vi "ADS1299EVM_Main.vi"() -> ()   [LabVIEW 2010]
doc: "ADS1292ECG-FE Software"
uses:
  Controls/Register/TYP_Reg_CHxSET.ctl
  Controls/Register/TYP_Reg_CONFIG1.ctl
  Controls/Register/TYP_Reg_CONFIG2.ctl
  Controls/Register/TYP_Reg_CONFIG3.ctl
  Controls/Register/TYP_Reg_LOFF.ctl
  Controls/Register/TYP_Reg_GPIO.ctl
  Controls/Register/TYP_Reg_MISC1.ctl
  Controls/Register/TYP_Reg_CONFIG4.ctl
  Controls/TYP_ACAnalysisParam.ctl
  lib_1299/Enqueue Classes/EVM Command class/EVMQueueCommand.lvclass
  lib_1299/Enqueue Classes/UserInput Command class/UserInput Command.lvclass
  lib_1299/Enqueue Classes/InternalState Command class/Internal State Command.lvclass
  Controls/Misc/TYP_DisableProp.ctl
  Modules/Estyx/TYP_ADS1299Estyx File Enum.ctl
  lib_1299/Enqueue Classes/UserDefined Command class/UserDefined Command class.lvclass
  Controls/Misc/TYP_PollingNotifierState.ctl
  Controls/Misc/TYP_PollingStatus.ctl
  Controls/Misc/TYP_SetTimeout.ctl
  Modules/Filter/TYP_FilterSettings.ctl
  <vilib>/event_ctls.llb/eventvkey.ctl
  lib_1299/Styx/lvstyx/Write/lvstyx_write_path_bool.vi
  <userlib>/Common/Queue with Cluster/Enqueue - Multiple Commands.vi
  lib_1299/Styx/lvstyx/Read/lvstyx_read_all_path_bool.vi
  lib_1299/Styx/lvstyx/Write/lvstyx_write_path_int.vi
  <vilib>/Utility/config.llb/Read Key (String).vi
  <vilib>/Utility/file.llb/Write To Spreadsheet File (string).vi
  <vilib>/Utility/file.llb/Write To Spreadsheet File (DBL).vi
  <vilib>/Utility/file.llb/Write To Spreadsheet File (I64).vi
  lib_1299/Styx/lvstyx/Read/lvstyx_read_all_path_hex.vi
  lib_1299/Styx/lvstyx/Read/lvstyx_read_all_path_int.vi
  lib_1299/lib1299.lvlib
  <vilib>/Analysis/NI_AALBase.lvlib
  <vilib>/Utility/config.llb/NI_LVConfig.lvlib
panel:
  in  "Normalize Data":bool=TRUE caption="Analysis Data is input referred"
  in  "Samples/CH":u32=1000
  in  "Show/Poll Lead Off Status":bool
  out "Status box":string="Connection Failure"
  in  "Acq - Single":bool
  out "Data Rate":dbl=500.0 format="%^#_6gSPS"
  in  "Acq - Continuous":bool
  out "Progress":u8(slide) caption="100%" scale=0.0..100.0
  out "ADC_ReadbackValue":u8 format="%.0x"
  in  "ADC_WriteValue":u8 format="%.0x"
  in  "ADC_Write2ADC":bool
  out "error out":errorcluster
  in  "error in (no error)":errorcluster
  in  "MainTab":T1(tab)
  out "About_FW_Ver":string caption="Firmware Version"
  out "About_DEV_ID":enum8{"ADS1299"}(ring) caption="Device ID"
  out "About_REV_ID":u8 caption="Rev"
  in  "Reset Mode":enum32{"Reset2Device", "Reset2Programmed"}(radio)=enum."Reset2Programmed"
  in  "RESET":bool caption="Reset"
  in  "STANDBY":bool caption="Standby"
  in  "Registers Tab":T2(tab)
  in  "CH8SET":T3={"PD#"=enum."Normal Operation", "GAIN#"=enum."24", "SRB2"=enum."Open (Off)", "MUX#"=enum."Normal Electrode"} caption="Channel 8 Control Register (CH8SET)"
  in  "CH7SET":T3={"PD#"=enum."Normal Operation", "GAIN#"=enum."24", "SRB2"=enum."Open (Off)", "MUX#"=enum."Normal Electrode"} caption="Channel 7 Control Register (CH7SET)"
  in  "CH6SET":T3={"PD#"=enum."Normal Operation", "GAIN#"=enum."24", "SRB2"=enum."Open (Off)", "MUX#"=enum."Normal Electrode"} caption="Channel 6 Control Register (CH6SET)"
  in  "CH5SET":T3={"PD#"=enum."Normal Operation", "GAIN#"=enum."24", "SRB2"=enum."Open (Off)", "MUX#"=enum."Normal Electrode"} caption="Channel 5 Control Register (CH5SET)"
  in  "CH4SET":T3={"PD#"=enum."Normal Operation", "GAIN#"=enum."24", "SRB2"=enum."Open (Off)", "MUX#"=enum."Normal Electrode"} caption="Channel 4 Control Register (CH4SET)"
  in  "CH3SET":T3={"PD#"=enum."Normal Operation", "GAIN#"=enum."24", "SRB2"=enum."Open (Off)", "MUX#"=enum."Normal Electrode"} caption="Channel 3 Control Register (CH3SET)"
  in  "CH2SET":T3={"PD#"=enum."Normal Operation", "GAIN#"=enum."24", "SRB2"=enum."Open (Off)", "MUX#"=enum."Normal Electrode"} caption="Channel 2 Control Register (CH2SET)"
  in  "CH1SET":T3={"PD#"=enum."Normal Operation", "GAIN#"=enum."24", "SRB2"=enum."Open (Off)", "MUX#"=enum."Normal Electrode"} caption="Channel 1 Control Register (CH1SET)"
  in  "Globally Set Channels":T3={"PD#"=enum."Normal Operation", "GAIN#"=enum."24", "SRB2"=enum."Open (Off)", "MUX#"=enum."Normal Electrode"}
  in  "CONFIG3":T4={"PD_REFBUF"=enum."Enabled", "BIAS_MEAS"=enum."Open", "BIASREF_INT"=enum."BIASREF fed externally", "PD_BIAS"=enum."Disabled"} caption="Configuration Register 3 (CONFIG3)"
  in  "CONFIG2":T5 caption="Configuration Register 2 (CONFIG2)"
  in  "CONFIG1":T6 caption="Configuration Register 1 (CONFIG1)"
  in  "LOFF":T7 caption="Lead-Off Control Register (LOFF)"
  in  "LOFF_FLIP_All":bool caption="Set All LOFF FLIP Bits"
  in  "LOFFN_All":bool caption="Set All LOFFN Bits"
  in  "LOFFP_All":bool caption="Set All LOFFP Bits"
  in  "LOFF_SENSP":bool[](array[boolean])=[FALSE, FALSE, FALSE, FALSE, FALSE, FALSE, FALSE, FALSE] caption="Lead Off Sense Positive Electrode"
  in  "LOFF_SENSN":bool[](array[boolean])=[FALSE, FALSE, FALSE, FALSE, FALSE, FALSE, FALSE, FALSE] caption="Lead Off Sense Negative Electrode"
  in  "LOFF_FLIP":bool[](array[boolean])=[FALSE, FALSE, FALSE, FALSE, FALSE, FALSE, FALSE, FALSE] caption="Lead Off Current Direction"
  in  "BIASSENSN":bool[](array[boolean])=[FALSE, FALSE, FALSE, FALSE, FALSE, FALSE, FALSE, FALSE] caption="Bias Sense Negative Electrode"
  in  "BIASSENSP":bool[](array[boolean])=[FALSE, FALSE, FALSE, FALSE, FALSE, FALSE, FALSE, FALSE] caption="Bias Sense Positive Electrode"
  in  "BIASSENSP_All":bool caption="Set All BIASSENSP Bits"
  in  "BIASSENSN_All":bool caption="Set All BIASSENSN Bits"
  in  "GPIO":T8={"GPIOC1"=TRUE, "GPIOC2"=TRUE, "GPIOC3"=TRUE, "GPIOC4"=TRUE, "GPIOD1"=FALSE, "GPIOD2"=FALSE, "GPIOD3"=FALSE, "GPIOD4"=FALSE} caption="General-Purpose I/O Register (GPIO)"
  in  "MISC1":T9
  in  "CONFIG4":T10 caption="Configuration Register 4 (CONFIG4)"
  in  "Refresh_ShadowReg":bool
  out "ShadowRegister":string[][](table) caption="Device Registers"
  in  "Analysis Control":enum32{"Scope", "Histogram", "FFT"}(tab)
  in  "Notch Freq":u16(ring)=60 items=["50Hz"=50, "60Hz"=60]
  in  "LPF Cutoff":dbl=0.1 caption="Cutoff Freq" format="%0.4fHz"
  in  "LPF Order":i32=3 caption="Filter Order"
  in  "LPF Enable":bool
  in  "Notch Order":i32=2 caption="Filter Order"
  in  "Notch Enable":bool
  in  "HPF Cutoff":dbl=0.1 caption="Cutoff Freq" format="%0.4fHz"
  in  "HPF Order":i32=3 caption="Filter Order"
  in  "HPF Enable":bool
  in  "Table_Scope":bool
  out "Graph - Scope":dbl[][](graph) caption="Scope Channels"
  in  "Plot Selector - Scope":u16(ring) caption="Plot" items=["All Channels", "Channel 1", "Channel 2", "Channel 3", "Channel 4", "Channel 5", "Channel 6", "Channel 7", "Channel 8"]
  in  "Histogram Bins":i32=10
  out "Graph - Histogram":T11(graph)
  in  "Plot Selector - Histogram":u16(ring) caption="Plot" items=["All Channels", "Channel 1", "Channel 2", "Channel 3", "Channel 4", "Channel 5", "Channel 6", "Channel 7", "Channel 8"]
  in  "Table_Histogram":bool
  in  "High Frequency":dbl=100.0 format="%.03pHz"
  out "Analysis - Dynamic Range":string[][](table) caption="Dynamic Range"
  in  "AC Analysis Parameters":T12={"DC Leakage"=5, "Number of Harmonics"=6, "HarmLeakage"=3, "FundLeakage"=15, "LoFreq (Hz)"=50.0, "HiFreq (Hz)"=100.0, "Window"=enum."None ", "Reference"=TRUE} {"HiFreq (Hz)" format="%.03pHz"; "LoFreq (Hz)" format="%.03pHz"; "FundLeakage" min=1 step=2; "HarmLeakage" min=1 step=2; "DC Leakage" min=1 step=1}
  in  "AinFreq_Desired":dbl=60.0 caption="Desired Ain Frequency" format="%0.3pHz"
  out "AinFreq_Ideal":dbl=60.1 caption="Ideal Ain Frequency" format="%.06pHz"
  in  "Input Amplitude(Vpp)":dbl=0.5 format="%.3g"
  out "Graph - FFT":cluster{i32, dbl, dbl[]}[](graph) caption="FFT Magnitude Plot (dB)"
  in  "Plot Selector - FFT":u16(ring) caption="Plot" items=["All Channels", "Channel 1", "Channel 2", "Channel 3", "Channel 4", "Channel 5", "Channel 6", "Channel 7", "Channel 8"]
  in  "Table_FFT":bool
  in  "Low Frequency":dbl=50.0 format="%.03pHz"
  in  "Save Data:Volts":bool caption="Data - Volts"
  in  "Save Analysis:FFT":bool caption="FFT Analysis"
  in  "Save_CH8":bool=TRUE caption="CH 8"
  in  "Save_CH7":bool=TRUE caption="CH 7"
  in  "Save_CH6":bool=TRUE caption="CH 6"
  in  "Save_CH5":bool=TRUE caption="CH 5"
  in  "Save_CH4":bool=TRUE caption="CH 4"
  in  "Save_CH3":bool=TRUE caption="CH 3"
  in  "Save_CH2":bool=TRUE caption="CH 2"
  in  "Save_CH1":bool=TRUE caption="CH 1"
  in  "Save Data:Histogram":bool caption="Histogram Data"
  in  "Save Data:FFT":bool caption="FFT Data"
  in  "Save Analysis:Scope":bool caption="Scope Analysis"
  in  "Save Analysis:Histogram":bool caption="Histogram Analysis"
  in  "Save Analysis:ShadowRegister":bool caption="Register Settings"
  in  "User Comments":string
  in  "Save Data:Codes":bool caption="Data - Codes"
  in  "Directory to Save Files":path=path "C:/Program Files/ADS1299ECG-FE/saved"
  in  "Record ID":i32 caption="Record Number"
  in  "Save to File":bool
  # "ADS1299EEG-FE"
  # "Debug - Manual Register Write"
  # "Product Safety Warnings, Restrictions and Disclaimers\n\nThe following Evaluation Board ADS1299ECG-FE set-up, use and application requirements must be followed:\n\n1.  NOT for diagnostic use.\n2.  NOT for for direct use with, or use in proximity of, an energized Defibrillator.\n3.  ONLY for Feasibility Evaluation in Laboratory/Development Environments.\n4.  The ADS1299ECG-FE intended application is solely for use in a laboratory/development environment, restricted to feasibility evaluation and development purposes, and not for\n     diagnostic purposes and/or interface with human beings and/or animals.\n5.  ONLY for use by qualified engineers and technicians familiar with the potential electrical shock, fire and personal injury risks associated in handling subassembly electrical and\n     mechanical components.\n6.  Use in conjunction with and/or adjacent to a defibrillator is strictly prohibited; application interface electronics shall not exceed their intended ratings. Refer to user instructions\n     and the ADS1299ECG-FE for further interface details.\n\n\nFor further information on application safety, refer to the standard TI terms and conditions documentation XXXXXXXXX"
  # "Motherboard:  MMB0\nTexas Instruments Inc (c) 2010"
  # "Reset Options"
  # "Global Channel Registers"
  # "Channel Control Registers"
  # "Lead-Off Detection and Current Direction Control Registers"
  # "LOFFP8             LOFFP7            LOFFP6             LOFFP5             LOFFP4             LOFFP3            LOFFP2             LOFFP1"
  # "LOFFN8             LOFFN7            LOFFN6             LOFFN5             LOFFN4            LOFFN3            LOFFN2             LOFFN1"
  # "LOFF_FLIP8      LOFF_FLIP7      LOFF_FLIP6      LOFF_FLIP5     LOFF_FLIP4      LOFF_FLIP3      LOFF_FLIP2     LOFF_FLIP1"
  # "BIAS Control Registers"
  # "BIASP8              BIASP7            BIASP6              BIASP5             BIASP4              BIASP3             BIASP2              BIASP1"
  # "BIASN8              BIASN7             BIASN6             BIASN5             BIASN4             BIASN3             BIASN2            BIASN1"
  # "Input"
  # "GPIOCx"
  # "Output"
  # "GPIODx"
  # "GPIO1                  GPIO2                 GPIO3                  GPIO4"
  # "(automatically updates if coming from another page)"
  # "Post Processing Filters"
  # "User Defined Dynamic Range"
  # "Coherent Frequency Calculator"
  # "User Comments/Notes"
  # "Analysis to Save:"
  # "Data to Save:"
  # "Channels to Save"
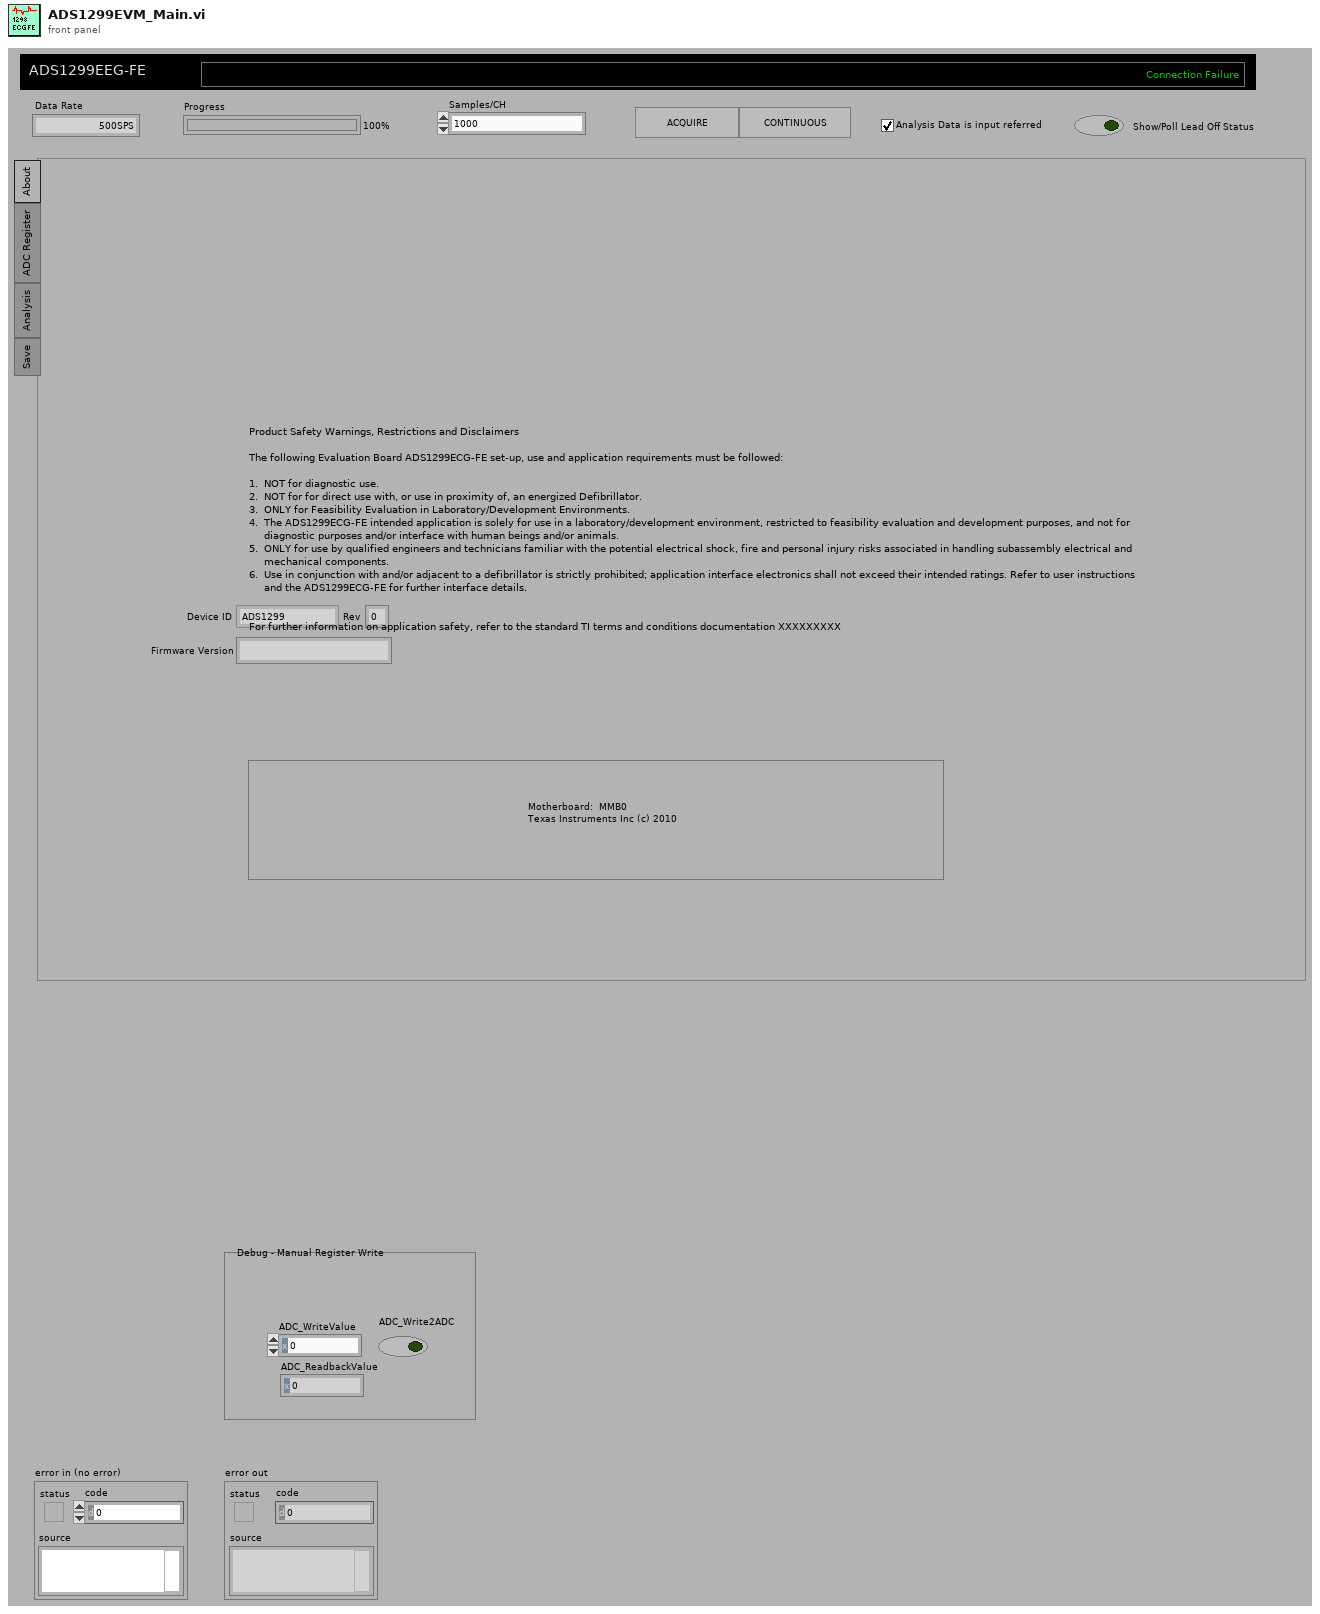
[diagram p1: front panel]
types:
  T1 = enum32{"About", "ADC Register", "Analysis", "Save"}
  T2 = enum32{"Channel Registers", "LOFF and BIAS", "GPIO and OTHER Registers", "Register Map"}
  T3 = typedef "TYP_Reg_CHxSET.ctl" = cluster{"PD#":enum16{"Normal Operation", "Power-down"}, "GAIN#":enum16{"1", "2", "4", "6", "8", "12", "24"}, "SRB2":enum16{"Open (Off)", "Closed (On)"}, "MUX#":enum16{"Normal Electrode", "Input Short", "BIAS Measurement", "MVDD", "Temperature Sensor", "Test Signal", "BIAS Positive Electrode Driver", "BIAS Negative Electrode Driver"}}
  T4 = typedef "TYP_Reg_CONFIG3.ctl" = cluster{"PD_REFBUF":enum16{"Disabled", "Enabled"}, "BIAS_MEAS":enum16{"Open", "BIASIN Routed"}, "BIASREF_INT":enum16{"BIASREF fed externally", "BIASREF = (AVDD-AVSS)/2"}, "PD_BIAS":enum16{"Disabled", "Enabled"}}
  T5 = typedef "TYP_Reg_CONFIG2.ctl" = cluster{"INT_CAL":enum16{"Driven Externally", "Generated Internally"}, "CAL_AMP":enum16{"(VREFP-VREFN)/2.4", "2x(VREFP-VREFN)/2.4"}, "CAL_FREQ":enum16{"f(CLK)/2^21", "f(CLK)/2^20", "N/A", "DC"}}
  T6 = typedef "TYP_Reg_CONFIG1.ctl" = cluster{"DAISY_EN":enum16{"Daisy Chain Mode", "Multiple Readback Mode"}, "CLK_EN":enum16{"Output Disabled", "Output Enabled"}, "DR":enum16{"f(MOD) /64", "f(MOD) /128", "f(MOD) /256", "f(MOD) /512", "f(MOD) /1024", "f(MOD) /2048", "f(MOD) /4096"}}
  T7 = typedef "TYP_Reg_LOFF.ctl" = cluster{"COMP_TH":enum16{"Positive - 95% : Negative - 5%", "Positive - 92.5% : Negative - 7.5%", "Positive - 90% : Negative - 10%", "Positive - 87.5% : Negative - 12.5%", "Positive - 85% : Negative - 15%", "Positive - 80% : Negative - 20%", "Positive - 75% : Negative - 25%", "Positive - 70% : Negative - 30%"}, "ILEAD_OFF":enum16{"6nA", "24nA", "6uA", "24uA"}, "FLEAD_OFF":enum16{"DC lead-off detection", "AC lead-off detection at SYS_CLK/(2^18)", "AC lead-off detection at SYS_CLK/(2^16)", "AC lead-off detection at fdr/4"}}
  T8 = typedef "TYP_Reg_GPIO.ctl" = cluster{"GPIOC1":bool, "GPIOC2":bool, "GPIOC3":bool, "GPIOC4":bool, "GPIOD1":bool, "GPIOD2":bool, "GPIOD3":bool, "GPIOD4":bool}
  T9 = typedef "TYP_Reg_MISC1.ctl" = cluster{"SRB1":enum16{"Open (Off)", "Closed (On)"}}
  T10 = typedef "TYP_Reg_CONFIG4.ctl" = cluster{"PD_LOFF_COMP":enum16{"Comparator Disabled", "Comparator Enabled"}}
  T11 = cluster{"X Values":dbl[], "Histogram: h(x)":i32[]}[]
  T12 = typedef "TYP_ACAnalysisParam.ctl" = cluster{"DC Leakage":i8, "Number of Harmonics":i8, "HarmLeakage":i8, "FundLeakage":i32, "LoFreq (Hz)":ext, "HiFreq (Hz)":ext, "Window":enum16{"None ", "Hanning", "Hamming", "Blackman-Harris", "Exact Blackman", "Blackman", "Flat Top", "4 Term B-Harris ", "7 Term B-Harris", "Low Sidelobe"}, "Reference":bool}
  T13 = typedef "TYP_ADS1299Estyx File Enum.ctl" = enum16{"|version", "|id", "ads1299evm|blocksize_samples", "ads1299evm|acquire", "ads1299evm|data", "conf|ch1set", "conf|ch2set", "conf|ch3set", "conf|ch4set", "conf|ch5set", "conf|ch6set", "conf|ch7set", "conf|ch8set", "conf|config1", "conf|config2", "conf|config3", "conf|devid", "conf|gpio", "conf|loff", "conf|loffflip", "conf|loffsensn", "conf|loffsensp", "conf|loffstatn", "conf|loffstatp", "conf|misc2", "conf|misc1", "conf|biassensn", "conf|biassensp", "conf|reset", "conf|sleep", "conf|config4", "led|dp", "led|seg", "led|ch", "mmb0|pll", "mmb0|clkout", "mmb0|clkfreq"}
  T14 = typedef "TYP_DisableProp.ctl" = u8
  T15 = typedef "TYP_PollingNotifierState.ctl" = cluster{"State":T16, "Data":i32}
  T16 = typedef "TYP_PollingStatus.ctl" = enum16{"Init", "Start", "Stop", "Pause", "Resume"}
  T17 = typedef "TYP_SetTimeout.ctl" = cluster{"Timeout (ms)":i16, "Timeout Enable?":bool}
  T18 = enum32{"invalid app kind", "Development System", "Run Time System", "Student Edition", "Embedded LabVIEW", "Evaluation", "Custom"}
  T19 = typedef "Rendezvous RefNum" = refnum<k1>
  T20 = typedef "TYP_AnalysisData.ctl" = cluster{"Status (Codes)":i32[], "Data (Codes)":i32[][], "Temp - Data (Volts)":dbl[][], "FFT":cluster{"FFT Data":cluster{i32, dbl, dbl[]}[], "Table Col Hdrs":string[], "Table Row Hdrs":string[], "Analysis Data":string[][], "CMRR/BW Table":string[][][]}, "Histogram":cluster{"Histogram Data":cluster{"X Values":dbl[], "Histogram: h(x)":i32[]}[], "Table Col Hdrs":string[], "Table Row Hdrs":string[], "Analysis Data":string[][]}, "Scope":cluster{"Table Col Hdrs":string[], "Table Row Hdrs":string[], "Analysis Data":string[][]}, "ECG":cluster{"AUX/LEAD":dbl[][], "Chest Leads":dbl[][], "Graph Labels (current)":string[]}, "Respiration":dbl[]}
  T21 = typedef "TYP_1299MainShifter.ctl" = cluster{"RegMap Data":T22[], "Register Names":string[], "ECG Zoom Limits":cluster{"Top":i32[], "Bottom":i32[]}, "Acq Timeout":u16, "f(CLK)":dbl, "Vref":dbl, "Word Bits":i32, "INI Info":cluster{"Data Dir":path, "Startup Dir":path, "Version":string, "Build":i16}, "Styx Enum Strings":string[]}
  T22 = typedef "TYP_ADSxxxx Register.ctl" = cluster{"Name":string, "Description":string, "Register":u16, "Default":u16, "Value":u16, "Base":u16, "RegMap Names":string[], "RegMap":T23[], "Item Count":u8}
  T23 = typedef "TYP_RegMap Item.ctl" = cluster{"Name":string, "MSB":u16, "LSB":u16, "Value":u16, "Mask":u16}
  T24 = typedef "eventvkey.ctl" = enum16{"ASCII", "Enter", "Return", "Shift", "Ctrl", "Alt", "Cmd", "Opt", "Caps", "NumLock", "Clear", "Break", "Up", "Down", "Left", "Right", "Insert", "Delete", "Home", "End", "PageUp", "PageDown", "Escape", "Help", "Pause", "ScrollLock", "F1", "F2", "F3", "F4", "F5", "F6", "F7", "F8", "F9", "F10", "F11", "F12", "F13", "F14", "F15", "F16", "F17", "F18", "F19", "F20", "F21", "F22", "F23", "F24", "Play", "VolumeUp", "VolumeDown", "Mute", "Two Byte Char"}
  T25 = enum32{"Channel Registers", "LOFF and RLD", "GPIO and OTHER Registers", "Register Map"}
  T26 = enum16{"DC lead-off detection", "AC lead-off detection at SYS_CLK/(2^18)", "AC lead-off detection at SYS_CLK/(2^16)", "AC lead-off detection at fdr/4"}
  T27 = enum16{"open", "replace", "create", "open or create", "replace or create", "replace or create with confirmation"}
  T28 = cluster{"LOFF_STATP":bool[], "LOFF_STATN":bool[]}
  T29 = enum16{"BIASREF fed externally", "BIASREF = (AVDD-AVSS)/2"}
  T30 = enum16{"Comparator Disabled", "Comparator Enabled"}
  T31 = typedef "TYP_Queue with Cluster Reference.ctl" = refnum<queue>
  T32 = typedef "lib1299.lvlib/TYP_EVM Plugin Pointers.ctl" = cluster{"Connection ptr":u32, "Client ptr":u32, "Data File ptr":u32}
  T33 = typedef "TYP_CtrlNameArray.ctl" = cluster{"References":refnum<vi>[], "Names/Labels":string[]}
  T34 = typedef "TYP_1299ShadowRegister.ctl" = cluster{"ID":T35, "Config1 ":T6, "Config2 ":T5, "Config3 ":T4, "Config4":T10, "CH1SET":T3, "CH2SET":T3, "CH3SET":T3, "CH4SET":T3, "CH5SET":T3, "CH6SET":T3, "CH7SET":T3, "CH8SET":T3, "MISC2":T36, "MISC1":T9, "LOFF ":T7, "BIASSENSP":bool[], "BIASSENSN":bool[], "LOFF_STATP":bool[], "LOFF_STATN":bool[], "LOFF_SENSP":bool[], "LOFF_SENSN":bool[], "LOFF_FLIP":bool[], "GPIO":cluster{"Data":bool[], "Direction":bool[]}}
  T35 = typedef "TYP_Reg_ID.ctl" = cluster{"REV_ID":u8, "DEV_ID":u16}
  T36 = typedef "TYP_Reg_MISC2.ctl" = cluster{"RegValue":dbl}
  T37 = typedef "TYP_CtrlRefShifter.ctl" = cluster{"Shadow Regs":cluster{"References":refnum<vi>[], "Names/Labels":string[]}, "Reg - PageCtrls":cluster{"References":refnum<vi>[], "Names/Labels":string[]}, "Reg - AllCtrls":cluster{"References":refnum<vi>[], "Names/Labels":string[]}, "Anlyz - PageCtrls":cluster{"References":refnum<vi>[], "Names/Labels":string[]}, "Anlyz - AllCtrls":cluster{"References":refnum<vi>[], "Names/Labels":string[]}}
  T38 = typedef "imagedata.ctl" = cluster{"image type":i32, "image depth":i32, "image":u8[], "mask":u8[], "colors":u32[], "Rectangle":cluster{"left":i16, "top":i16, "right":i16, "bottom":i16}}
  T39 = typedef "NI_LVConfig.lvlib/Config Data RefNum.ctl" = refnum<k1>
  T40 = typedef "TYP_Queue Cluster Element.ctl" = cluster{"Command":string, "Data":variant}
  T41 = typedef "TYP_FilterSettings.ctl" = cluster{"Cutoff":dbl, "Order":i32}
  T42 = cluster{"Freq (Hz)":dbl[][], "SNR (dBFS)":dbl[], "Fund(dB)":dbl}
  T43 = cluster{"SNR(dBFS)":dbl, "SNRD(dB)":dbl, "THD (dBc)":dbl, "SFDR(dBc)":dbl, "ENOB":dbl, "enob":dbl, "#ofHarm(SNR)":dbl, "WoSpur(dbFS)":dbl, "2nd HD (dBc)":dbl, "3rd HD (dBc)":dbl, "4th HD (dBc)":dbl, "5th HD (dBc)":dbl, "Ampl.":dbl}
  T44 = cluster{"X Values":dbl[], "Histogram: h(x)":i32[]}
  T45 = cluster{"DAISY_EN":enum16{"Daisy Chain Mode", "Multiple Readback Mode"}, "CLK_EN":enum16{"Output Disabled", "Output Enabled"}, "DR":enum16{"f(MOD) /64", "f(MOD) /128", "f(MOD) /256", "f(MOD) /512", "f(MOD) /1024", "f(MOD) /2048", "f(MOD) /4096"}}
  T46 = cluster{"INT_CAL":enum16{"Driven Externally", "Generated Internally"}, "CAL_AMP":enum16{"(VREFP-VREFN)/2.4", "2x(VREFP-VREFN)/2.4"}, "CAL_FREQ":enum16{"f(CLK)/2^21", "f(CLK)/2^20", "N/A", "DC"}}
  T47 = cluster{"PD_REFBUF":enum16{"Disabled", "Enabled"}, "BIAS_MEAS":enum16{"Open", "BIASIN Routed"}, "BIASREF_INT":enum16{"BIASREF fed externally", "BIASREF = (AVDD-AVSS)/2"}, "PD_BIAS":enum16{"Disabled", "Enabled"}}
  T48 = cluster{"PD_LOFF_COMP":enum16{"Comparator Disabled", "Comparator Enabled"}}
  T49 = enum16{"f(MOD) /64", "f(MOD) /128", "f(MOD) /256", "f(MOD) /512", "f(MOD) /1024", "f(MOD) /2048", "f(MOD) /4096"}
  T50 = cluster{"COMP_TH":enum16{"Positive - 95% : Negative - 5%", "Positive - 92.5% : Negative - 7.5%", "Positive - 90% : Negative - 10%", "Positive - 87.5% : Negative - 12.5%", "Positive - 85% : Negative - 15%", "Positive - 80% : Negative - 20%", "Positive - 75% : Negative - 25%", "Positive - 70% : Negative - 30%"}, "ILEAD_OFF":enum16{"6nA", "24nA", "6uA", "24uA"}, "FLEAD_OFF":enum16{"DC lead-off detection", "AC lead-off detection at SYS_CLK/(2^18)", "AC lead-off detection at SYS_CLK/(2^16)", "AC lead-off detection at fdr/4"}}
  T51 = cluster{"SRB1":enum16{"Open (Off)", "Closed (On)"}}
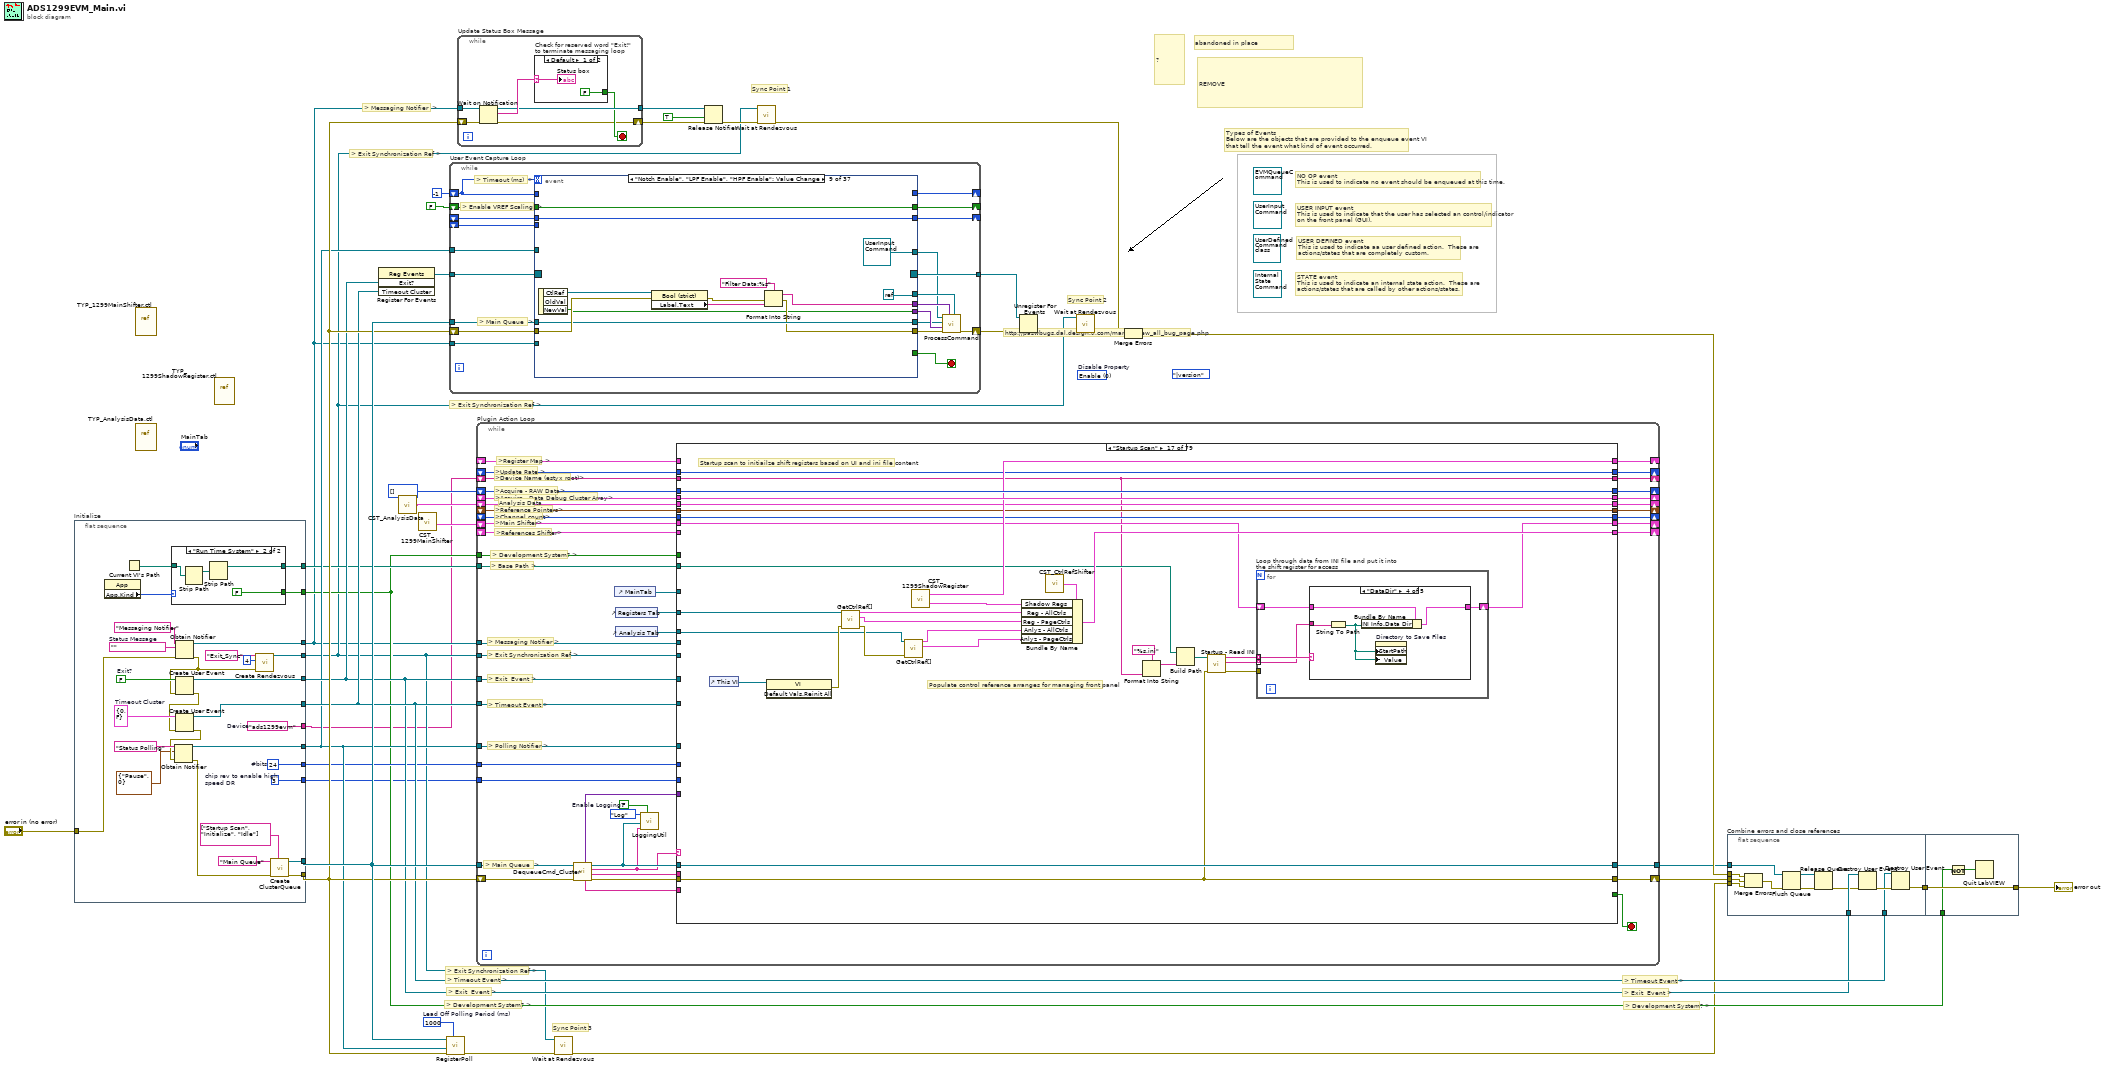
[diagram p0: block diagram]
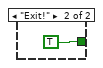
[diagram p2: hidden frame]
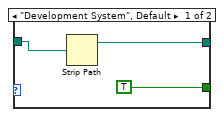
[diagram p3: hidden frame]
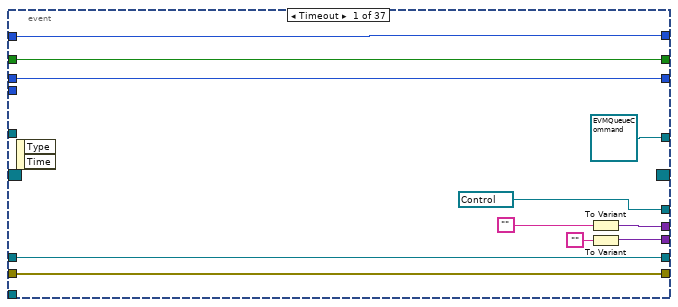
[diagram p4: hidden frame]
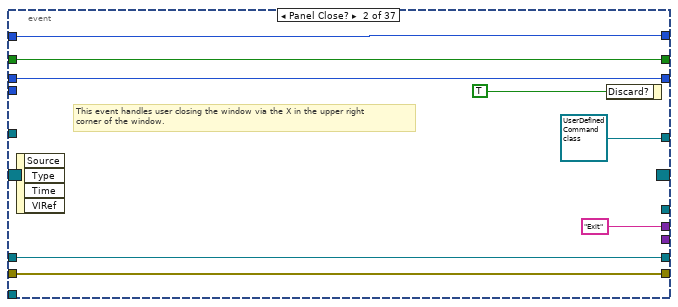
[diagram p5: hidden frame]
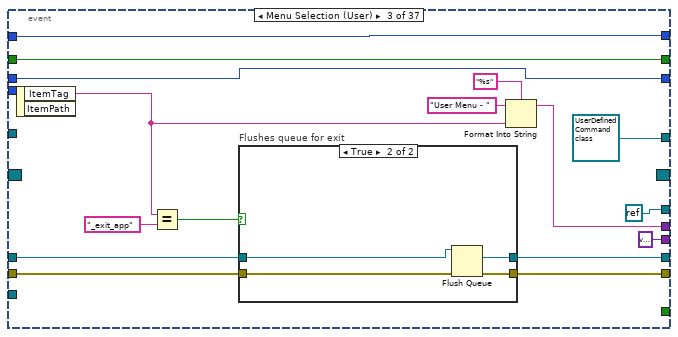
[diagram p6: hidden frame]
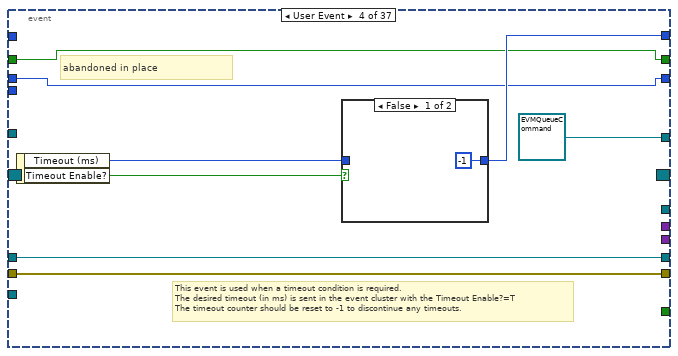
[diagram p8: hidden frame]
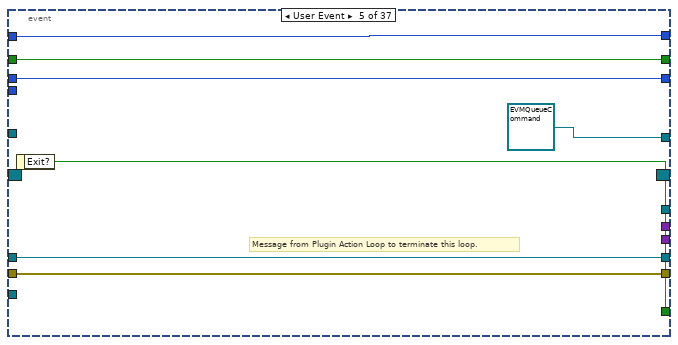
[diagram p10: hidden frame]
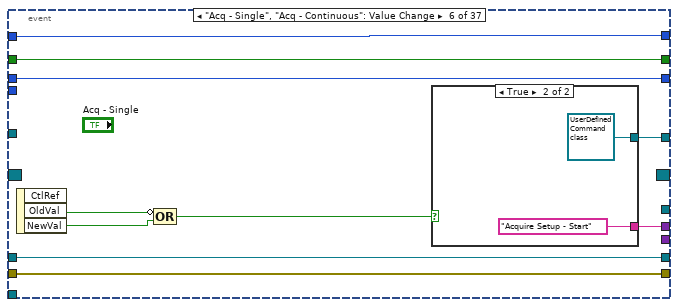
[diagram p11: hidden frame]
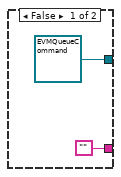
[diagram p12: hidden frame]
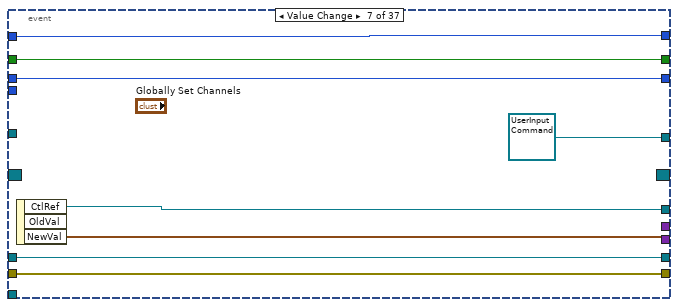
[diagram p13: hidden frame]
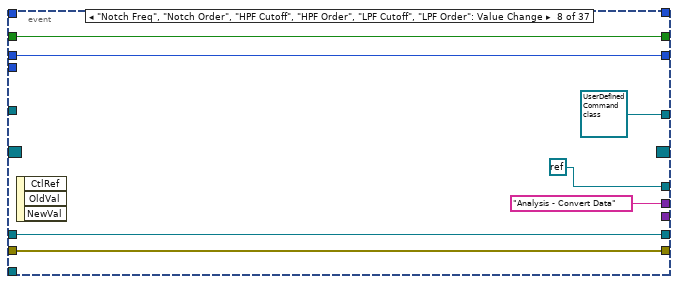
[diagram p14: hidden frame]
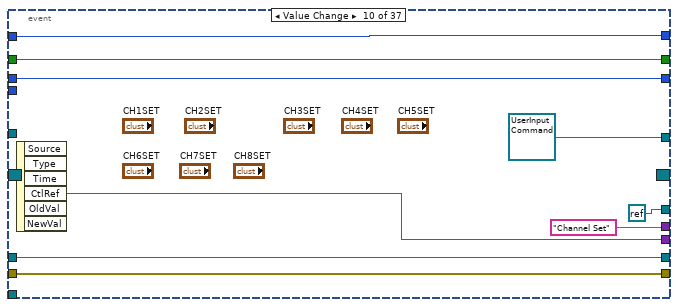
[diagram p15: hidden frame]
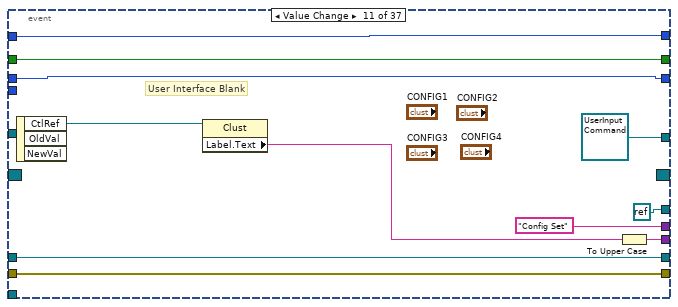
[diagram p16: hidden frame]
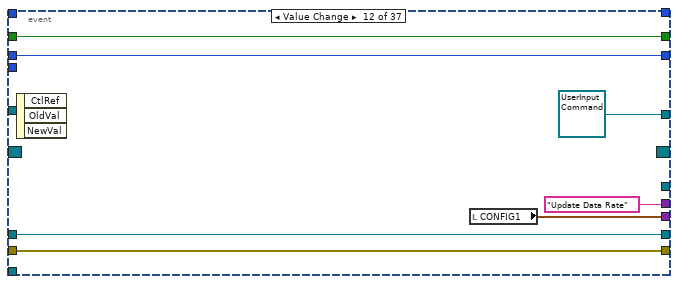
[diagram p17: hidden frame]
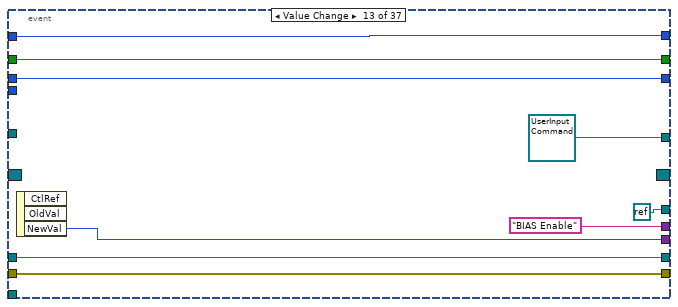
[diagram p18: hidden frame]
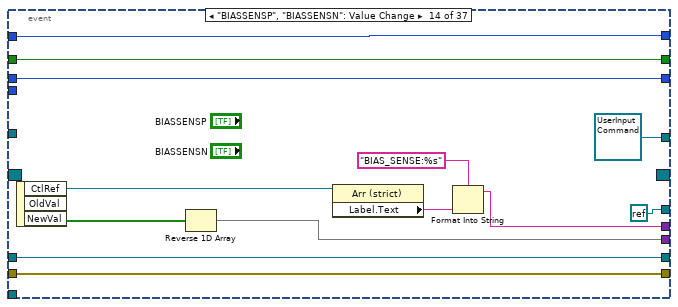
[diagram p19: hidden frame]
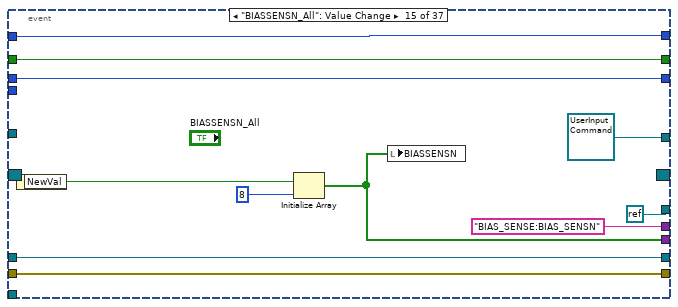
[diagram p20: hidden frame]
diagram:
  (unwired) refnum<class "UserDefined Command class.lvclass"> refnum ("UserDefined Command class.lvclass")
  (unwired) TYP_ADS1299Estyx_File_Enum."|version" ("Styx File Tags - Enum")
  w25 = 1000  # Lead Off Polling Period (ms)
  (unwired) T14 0 items=["Enable", "Disable", "Disable/Gray"]  # Disable Property
  (unwired) refnum<class "Internal State Command.lvclass"> refnum ("Internal State Command.lvclass")
  (unwired) refnum<class "UserInput Command.lvclass"> refnum ("UserInput Command.lvclass")
  (unwired) refnum<class "EVMQueueCommand.lvclass"> refnum ("EVMQueueCommand.lvclass")
  # "http://paswbugs.dal.design.ti.com/mantis/view_all_bug_page.php"
  # "Sync Point 3"
  # "Sync Point 2"
  # "Sync Point 1"
  # "> Exit Synchronization Ref >"
  # "> Exit Synchronization Ref >"
  # "> Exit Synchronization Ref >"
  # "> Development System? >"
  # "> Development System? >"
  # "abandoned in place"
  # "USER DEFINED event\nThis is used to indicate aa user defined action.  These are \nactions/states that are completely custom."
  # "REMOVE"
  # "?"
  # "STATE event\nThis is used to indicate an internal state action.  These are \nactions/states that are called by other actions/states."
  # "USER INPUT event\nThis is used to indicate that the user has selected an control/indicator\non the front panel (GUI)."
  # "NO OP event\nThis is used to indicate no event should be enqueued at this time."
  # "Types of Events\nBelow are the objects that are provided to the enqueue event VI\nthat tell the event what kind of event occurred."
  # "> Messaging Notifier  >"
  # "> Timeout Event >"
  # "> Exit  Event >"
  # "> Timeout Event >"
  # "> Exit  Event >"
  n1 = flat-sequence "Initialize" {
    tunnel: [w54] -> w24
    tunnel: [w55] -> w26
    tunnel: [w65] -> w21
    tunnel: [w62] -> w22
    tunnel: "error in (no error)" -> [w60]
    tunnel: [w58] -> w2
    tunnel: [w49] -> w20
    tunnel: [w47] -> w16
    tunnel: [w44] -> w15
    tunnel: [w43] -> w12
    tunnel: [w39] -> w5
    tunnel: [w38] -> w4
    tunnel: [w37] -> w1
    frame #0 {
      w37 = "ads1299evm"  # Device
      w38 = 3  # chip rev to enable high speed DR
      w47 = 24  # #bits
      w57 = ""  # Status Message
      w63 = T17 {"Timeout (ms)"=0, "Timeout Enable?"=FALSE}  # Timeout Cluster
      w64 = FALSE  # Exit?
      n2 = property class="App"() -> ("App.Kind"=w46:T18)  [unwired: 2 in, 2 out]
      n3 = Current VI's Path() -> (path=w45:path)
      n4 = case shown="\"Run Time System\"" w46 {
        tunnel: w45 -> [w68 w72]
        tunnel: [w67 w70] -> w44
        tunnel: [TRUE FALSE] -> w43
        frame "Development System", Default {
          n5 = Strip Path(path=w68) -> (stripped path=w67:path)  [unwired: 1 out]
        }
        frame "Run Time System" {
          n6 = Strip Path(path=w72) -> (stripped path=w71:path)  [unwired: 1 out]
          n7 = Strip Path(path=w71) -> (stripped path=w70:path)  [unwired: 1 out]
        }
      }
      n8 = Obtain Notifier(name (unnamed)="Messaging Notifier", notification data type=w57, error in (no error)=w60) -> (notifier out=w58:refnum<notifier>, error out=w42:errorcluster)  [unwired: 1 in, 1 out]
      n9 = Create User Event(user event datatype=w64, error in=w42) -> (user event=w65:refnum<user-event>, error out=w61:errorcluster)
      n10 = Create User Event(user event datatype=w63, error in=w61) -> (user event=w62:refnum<user-event>, error out=w51:errorcluster)
      n11 = Obtain Notifier(name (unnamed)="Status Polling", notification data type=T15 {"State"=enum."Pause", "Data"=0} ("PollingNotifier"), error in (no error)=w51) -> (notifier out=w49:refnum<notifier>, error out=w50:errorcluster)  [unwired: 1 in, 1 out]
      n12 = call <vilib>:"Create Rendezvous.vi"("error in (no error)"=w42, "size (2)"=4, "name (unnamed)"="Exit_Sync") -> ("rendezvous"=w39:T19)  [unwired: 4 out]
      n13 = call <userlib>:"Create ClusterQueue.vi"("Initial Commands"=string[] ["Startup Scan", "Initialize", "Idle"], "error in"=w50, "Queue Name"="Main Queue" ("name (unnamed)")) -> ("error out"=w54:errorcluster, "Queue Out"=w55:refnum<queue>)  [unwired: 7 out]
    }
  }
  n14 = vi-ref "TYP_1299MainShifter.ctl"() -> ()  [unwired: 1 out]
  n15 = vi-ref "TYP_AnalysisData.ctl"() -> ()  [unwired: 1 out]
  n16 = vi-ref "TYP_1299ShadowRegister.ctl"() -> ()  [unwired: 1 out]
  n17 = register-events(w21, w22) -> (reference out=w35:refnum<event-registration>)  [unwired: 2 in, 1 out]
  n18 = call "CST_AnalysisData.vi"() -> ("Analysis Data"=w18:T20)  [unwired: 1 out]
  n19 = call "CST_1299MainShifter.vi"() -> ("Main Shifter"=w19:T21)  [unwired: 11 out]
  n20 = call "RegisterPoll.vi"("Timeout (ms)"=w25, "error in (no error)"=w24, "Polling Notifier"=w20, "Main App Queue"=w26) -> ("error out"=w11:errorcluster)  [unwired: 7 out]
  n21 = while "User Event Capture Loop" {
    shift-right: [w85] -> w34
    shift-left: w24 -> [w93]
    tunnel: w26 -> [w92]
    shift-right: [w89] -> _
    shift-left: -1 -> [w90]
    tunnel: w35 -> [w88]
    tunnel: [w87] -> w33
    tunnel: w20 -> [w79]
    shift-right: [w78] -> _
    shift-left: _ -> [w77]
    shift-left: _ -> [w76]
    shift-right: [w74] -> _
    shift-left: FALSE -> [w75]
    tunnel: w2 -> [w73]
    stop <- w91 stop-if-true
    # "> Enable VREF Scaling  >"
    # "> Timeout (ms)  >"
    # "> Main Queue  >"
    n22 = event shown="[8] \"Notch Enable\", \"LPF Enable\", \"HPF Enable\": Value Change" {
      selector: w88 -> [_ _ _ _ _ _ _ _ _ _ _ _ _ _ _ _ _ _ _ _ _ _ _ _ _ _ _ _ _ _ _ _ _ _ _ _ _]
      dyn-events: [_ _ _ _ _ _ _ _ _ _ _ _ _ _ _ _ _ _ _ _ _ _ _ _ _ _ _ _ _ _ _ _ _ _ _ _ _] -> w87
      timeout: w90 -> [_ _ _ _ _ _ _ _ _ _ _ _ _ _ _ _ _ _ _ _ _ _ _ _ _ _ _ _ _ _ _ _ _ _ _ _ _]
      tunnel: [w103 w110 w123 w142 w151 w159 w172 w175 w184 w201 w212 w215 w228 w241 w248 w259 w272 w275 w312 w320 w328 w339 w350 w365 w379 w392 w398 w411 w420 w431 w437 w444 w450 w456 w468 w477 w487] -> w86
      tunnel: w93 -> [w103 w110 w115 w142 w151 w159 w172 w175 w188 w201 w212 w215 w228 w241 w248 w259 w272 w275 w312 w320 w328 w339 w350 w365 w379 w392 w398 w411 w420 w431 w437 w444 w450 w456 w468 w477 w487]
      tunnel: w92 -> [w96 w109 w124 w137 w147 w158 w169 w176 w187 w199 w210 w214 w227 w239 w249 w260 w270 w276 w310 w321 w329 w340 w351 w363 w377 w391 w399 w412 w419 w430 w436 w445 w451 w457 w471 w478 w484]
      tunnel: [_ _ _ _ w150 _ _ _ _ _ _ _ _ _ _ _ _ _ _ _ _ _ _ _ _ _ _ _ _ _ _ _ _ _ _ _ _] -> w91
      tunnel: w90 -> [w104 w111 w116 _ w149 w161 w173 _ _ w202 w213 _ w229 w242 w253 w264 w273 w279 w313 w322 w333 w344 w355 w366 w380 w393 w401 w414 w421 w432 w439 w446 w453 w460 w472 w480 w488]
      tunnel: [w104 w111 w116 w139 w149 w161 w173 _ _ w202 w213 _ w229 w242 w253 w264 w273 w279 w313 w322 w333 w344 w355 w366 w380 w393 w401 w414 w421 w432 w439 w446 w453 w460 w472 w480 w488] -> w89
      tunnel: [refnum<class "EVMQueueCommand.lvclass"> refnum ("EVMQueueCommand.lvclass") refnum<class "UserDefined Command class.lvclass"> refnum ("UserDefined Command class.lvclass") refnum<class "UserDefined Command class.lvclass"> refnum ("UserDefined Command class.lvclass") refnum<class "EVMQueueCommand.lvclass"> refnum ("EVMQueueCommand.lvclass") refnum<class "EVMQueueCommand.lvclass"> refnum ("EVMQueueCommand.lvclass") w160 refnum<class "UserInput Command.lvclass"> refnum ("UserInput Command.lvclass") refnum<class "UserDefined Command class.lvclass"> refnum ("UserDefined Command class.lvclass") refnum<class "UserInput Command.lvclass"> refnum ("UserInput Command.lvclass") refnum<class "UserInput Command.lvclass"> refnum ("UserInput Command.lvclass") refnum<class "UserInput Command.lvclass"> refnum ("UserInput Command.lvclass") refnum<class "UserInput Command.lvclass"> refnum ("UserInput Command.lvclass") refnum<class "UserInput Command.lvclass"> refnum ("UserInput Command.lvclass") refnum<class "UserInput Command.lvclass"> refnum ("UserInput Command.lvclass") refnum<class "UserInput Command.lvclass"> refnum ("UserInput Command.lvclass") refnum<class "UserInput Command.lvclass"> refnum ("UserInput Command.lvclass") refnum<class "UserInput Command.lvclass"> refnum ("UserInput Command.lvclass") refnum<class "EVMQueueCommand.lvclass"> refnum ("EVMQueueCommand.lvclass") refnum<class "UserInput Command.lvclass"> refnum ("UserInput Command.lvclass") refnum<class "UserInput Command.lvclass"> refnum ("UserInput Command.lvclass") refnum<class "UserInput Command.lvclass"> refnum ("UserInput Command.lvclass") refnum<class "UserInput Command.lvclass"> refnum ("UserInput Command.lvclass") refnum<class "UserInput Command.lvclass"> refnum ("UserInput Command.lvclass") refnum<class "UserInput Command.lvclass"> refnum ("UserInput Command.lvclass") refnum<class "UserInput Command.lvclass"> refnum ("UserInput Command.lvclass") refnum<class "UserDefined Command class.lvclass"> refnum ("UserDefined Command class.lvclass") refnum<class "Internal State Command.lvclass"> refnum ("Internal State Command.lvclass") w408 refnum<class "UserDefined Command class.lvclass"> refnum ("UserDefined Command class.lvclass") refnum<class "UserDefined Command class.lvclass"> refnum ("UserDefined Command class.lvclass") refnum<class "UserDefined Command class.lvclass"> refnum ("UserDefined Command class.lvclass") refnum<class "UserDefined Command class.lvclass"> refnum ("UserDefined Command class.lvclass") refnum<class "UserDefined Command class.lvclass"> refnum ("UserDefined Command class.lvclass") refnum<class "UserDefined Command class.lvclass"> refnum ("UserDefined Command class.lvclass") refnum<class "EVMQueueCommand.lvclass"> refnum ("EVMQueueCommand.lvclass") refnum<class "UserDefined Command class.lvclass"> refnum ("UserDefined Command class.lvclass") refnum<class "UserInput Command.lvclass"> refnum ("UserInput Command.lvclass")] -> w81
      tunnel: [w102 "Exit" w118 _ _ w157 _ "Analysis - Convert Data" w183 "Channel Set" "Config Set" "Update Data Rate" "BIAS Enable" w233 "BIAS_SENSE:BIAS_SENSN" "BIAS_SENSE:BIAS_SENSP" _ _ w304 "Lead-off Detect Enable" "LOFF_ARRAY:LOFF_SENSN" "LOFF_ARRAY:LOFF_SENSP" "LOFF_ARRAY:LOFF_FLIP" w360 w371 w384 "ReadUserRegisters" "ReadUserRegisters" "Analysis - Convert Data" "Analysis Table" ("initial string") "Analysis - Histogram" "CalculateFin" "CalculateFin" "Analysis - FFT" _ "Save to File" "WriteReadADC"] -> w83
      tunnel: [refnum<vi> refnum ("CtlRef") _ refnum<k0> refnum ("Not a Refnum Constant") _ _ _ w170 refnum<k0> refnum ("Not a Refnum Constant") refnum<k0> refnum ("Not a Refnum Constant") refnum<k0> refnum ("Not a Refnum Constant") refnum<k0> refnum ("Not a Refnum Constant") _ refnum<k0> refnum ("Not a Refnum Constant") refnum<k0> refnum ("Not a Refnum Constant") refnum<k0> refnum ("Not a Refnum Constant") refnum<k0> refnum ("Not a Refnum Constant") w268 _ refnum<k0> refnum ("Not a Refnum Constant") refnum<k0> refnum refnum<k0> refnum ("Not a Refnum Constant") refnum<k0> refnum ("Not a Refnum Constant") refnum<k0> refnum ("Not a Refnum Constant") refnum<k0> refnum refnum<k0> refnum ("Not a Refnum Constant") _ _ _ _ _ _ _ _ _ _ _ _] -> w84
      tunnel: [w98 _ variant ("NewVal") _ _ _ w168 _ w181 w198 w206 w216 w223 w237 w245 w256 w267 _ w308 w317 w325 w336 w347 w359 w376 _ FALSE FALSE _ w425 _ _ _ _ _ _ w483] -> w82
      tunnel: [w96 w109 w122 w137 w147 w158 w169 w176 w187 w199 w210 w214 w227 w239 w249 w260 w270 w276 w310 w321 w329 w340 w351 w363 w377 w391 w399 w412 w419 w430 w436 w445 w451 w457 w471 w478 w484] -> w80
      tunnel: w79 -> [_ _ _ _ _ _ _ _ _ _ _ _ _ _ _ _ _ _ _ _ _ _ _ _ _ _ _ _ _ _ _ _ _ _ w469 _ _]
      tunnel: [w95 w106 w114 w136 w146 w153 w167 w180 w193 w194 w204 w220 w222 w231 w244 w255 w266 w282 w302 w315 w324 w335 w346 w357 w368 w382 w395 w403 w416 w423 w434 w441 w448 w455 w462 w475 w482] -> w78
      tunnel: w77 -> [w95 w106 w114 w136 w146 w153 w167 w180 w193 w194 w204 w220 w222 w231 w244 w255 w266 w280 w302 w315 w324 w335 w346 w357 w368 w382 w395 w403 w416 w423 w434 w441 w448 w455 w462 w475 w482]
      tunnel: w76 -> [_ _ _ _ _ _ _ _ _ _ _ _ _ _ _ _ _ w281 _ _ _ _ _ _ _ _ _ _ _ _ _ _ _ _ _ _ _]
      tunnel: w75 -> [w94 w105 w113 w135 w145 w152 w166 w179 w192 w195 w203 w219 w221 w230 w243 w254 w265 w278 w301 w314 w323 w334 w345 w356 w367 w381 w394 w402 w415 w422 w433 w440 w447 w454 w461 w474 w481]
      tunnel: [w94 w105 w113 w135 w145 w152 w166 w179 w192 w195 w203 w219 w221 w230 w243 w254 w265 w277 w301 w314 w323 w334 w345 w356 w367 w381 w394 w402 w415 w422 w433 w440 w447 w454 w461 w474 w481] -> w74
      tunnel: w73 -> [_ _ _ _ _ _ _ _ _ _ _ _ _ _ _ _ _ w274 _ _ _ _ _ _ _ _ _ _ _ _ _ _ _ _ _ _ _]
      event Timeout {
        n23 = event-data() -> ()  [unwired: 3 out]
        n24 = To Variant(anything="" ("Empty String Constant")) -> (Variant=w102:variant)
        n25 = To Variant(anything="" ("Empty String Constant")) -> (Variant=w98:variant)
      }
      event Panel Close? {
        # "This event handles user closing the window via the X in the upper right\ncorner of the window."
        n26 = event-data() -> ()  [unwired: 5 out]
        n27 = event-data ("Event Filter Node")("Discard?"=TRUE) -> ()  [unwired: 1 in, 1 out]
      }
      event Menu Selection (User) {
        n28 = event-data() -> ("ItemTag"=w121:string)  [unwired: 2 out]
        n29 = Equal?(x=w121, y="_exit_app") -> (x = y?=w125:bool)
        n30 = case "Flushes queue for exit" shown="True" w125 {
          tunnel: w115 -> [w129 w131]
          tunnel: w124 -> [w130 w134]
          tunnel: [w130 w133] -> w122
          tunnel: [w129 w132] -> w123
          frame False {
          }
          frame True {
            n31 = Flush Queue(queue=w134, error in (no error)=w131) -> (queue out=w133:refnum<queue>, error out=w132:errorcluster)  [unwired: 1 out]
          }
        }
        n32 = Format Into String(format string="%s", initial string="User Menu - ", w121) -> (resulting string=w118:string)  [unwired: 1 in, 1 out]
      }
      event User Event {
        # "abandoned in place"
        # "This event is used when a timeout condition is required.\nThe desired timeout (in ms) is sent in the event cluster with the Timeout Enable?=T\nThe timeout counter should be reset to -1 to discontinue any timeouts."
        n33 = event-data() -> ("Timeout (ms)"=w140:i16, "Timeout Enable?"=w141:bool)  [unwired: 1 out]
        n34 = case shown="False" w141 {
          tunnel: w140 -> [_ w144]
          tunnel: [i16 -1 ("Timeout (ms)") w144] -> w139
          frame False {
          }
          frame True {
          }
        }
      }
      event User Event {
        # "Message from Plugin Action Loop to terminate this loop."
        n35 = event-data() -> ("Exit?"=w150:bool)  [unwired: 1 out]
      }
      event "Acq - Single", "Acq - Continuous": Value Change {
        n36 = event-data() -> ("OldVal"=w156:bool, "NewVal"=w155:bool)  [unwired: 2 out]
        n37 = Compound Arithmetic op=OR(invert w156, w155) -> (w154:bool)
        n38 = case shown="True" w154 {
          tunnel: [refnum<class "EVMQueueCommand.lvclass"> refnum ("EVMQueueCommand.lvclass") refnum<class "UserDefined Command class.lvclass"> refnum ("UserDefined Command class.lvclass")] -> w160
          tunnel: ["" "Acquire Setup - Start"] -> w157
          frame False {
          }
          frame True {
          }
        }
      }
      event Value Change {
        n39 = event-data() -> ("CtlRef"=w170:refnum<vi>, "NewVal"=w168:T3)  [unwired: 2 out]
      }
      event "Notch Freq", "Notch Order", "HPF Cutoff", "HPF Order", "LPF Cutoff", "LPF Order": Value Change {
        n40 = event-data() -> ()  [unwired: 4 out]
      }
      event "Notch Enable", "LPF Enable", "HPF Enable": Value Change {
        n41 = event-data() -> ("CtlRef"=w189:refnum<vi>, "NewVal"=w181:bool)  [unwired: 2 out]
        n42 = property class="Bool (strict)"(reference=w189, error in=w188) -> (error out=w185:errorcluster, "Label.Text"=w191:string)  [unwired: 1 out]
        n43 = Format Into String(format string="Filter Data:%s", error in=w185, w191) -> (resulting string=w183:string, error out=w184:errorcluster)  [unwired: 1 in]
      }
      event Value Change {
        n44 = event-data() -> ("CtlRef"=w198:refnum<vi>)  [unwired: 6 out]
      }
      event Value Change {
        # "User Interface Blank"
        n45 = event-data() -> ("CtlRef"=w208:refnum<vi>)  [unwired: 3 out]
        n46 = property on="Property Node" class="Clust"(reference=w208) -> ("Label.Text"=w205:string)  [unwired: 1 in, 2 out]
        n47 = To Upper Case(1:w205) -> (0:w206:string)
      }
      event Value Change {
        n48 = event-data() -> ()  [unwired: 4 out]
        n49 = local read "CONFIG1"() -> (w216:T6)
      }
      event Value Change {
        n50 = event-data() -> ("NewVal"=w223:enum16{"Disabled", "Enabled"})  [unwired: 3 out]
      }
      event "BIASSENSP", "BIASSENSN": Value Change {
        n51 = event-data() -> ("CtlRef"=w236:refnum<vi>, "NewVal"=w238:bool[])  [unwired: 2 out]
        n52 = Reverse 1D Array(array=w238) -> (reversed array=w237:bool[])
        n53 = property on="Property Node" class="Arr (strict)"(reference=w236) -> ("Label.Text"=w235:string)  [unwired: 1 in, 2 out]
        n54 = Format Into String(format string="BIAS_SENSE:%s", w235) -> (resulting string=w233:string)  [unwired: 2 in, 1 out]
      }
      event "BIASSENSN_All": Value Change {
        n55 = event-data() -> ("NewVal"=w246:bool)  [unwired: 1 out]
        n56 = Initialize Array(w246, 8 ("dimension size")) -> (w245:bool[])
        n57 = local write "BIASSENSN"(w245) -> ()
      }
      event "BIASSENSP_All": Value Change {
        n58 = event-data() -> ("NewVal"=w257:bool)  [unwired: 3 out]
        n59 = Initialize Array(w257, 8 ("dimension size")) -> (w256:bool[])
        n60 = local write "BIASSENSP"(w256) -> ()
      }
      event Value Change {
        n61 = event-data() -> ("CtlRef"=w269:refnum<vi>)  [unwired: 6 out]
        n62 = property on="Property Node" class="Clust"(reference=w269) -> (reference out=w268:refnum<vi>, "Label.Text"=w267:string)  [unwired: 1 in, 1 out]
      }
      event Key Down {
        w288 = i16 71  # "G"
        n63 = event-data() -> ("Char"=w283:i16, "VKey"=w282:T24)  [unwired: 2 out]
        n64 = Equal?(x=w280, y=eventvkey."Shift") -> (x = y?=w289:bool)
        n65 = Equal?(x=w288, y=w283) -> (x = y?=w292:bool)
        n66 = Equal?(x=w281, y=eventvkey."Ctrl") -> (x = y?=w290:bool)
        n67 = Equal?(x=eventvkey."ASCII" ("y"), y=w282) -> (x = y?=w291:bool)
        n68 = Compound Arithmetic op=AND(w289, w290, w291, w292) -> (w293:bool)
        n69 = case shown="True" w293 {
          tunnel: w278 -> [w294 w300]
          tunnel: [w294 w296] -> w277
          tunnel: w274 -> [_ w299]
          frame False {
          }
          frame True {
            n70 = Not(x=w300) -> (.not. x?=w296:bool)
            n71 = Select(t="Vref Scaling Mode Active" ("notification"), s=w296, f="Ready..." ("notification")) -> (s? t:f=w297:string)
            n72 = Send Notification(notification=w297, notifier=w299) -> ()  [unwired: 1 in, 2 out]
          }
        }
      }
      event "LOFF_SENSP", "LOFF_SENSN", "LOFF_FLIP": Value Change {
        n73 = event-data() -> ("CtlRef"=w307:refnum<vi>, "NewVal"=w309:bool[])  [unwired: 2 out]
        n74 = Reverse 1D Array(array=w309) -> (reversed array=w308:bool[])
        n75 = property on="Property Node" class="Arr (strict)"(reference=w307) -> ("Label.Text"=w306:string)  [unwired: 1 in, 2 out]
        n76 = Format Into String(format string="LOFF_ARRAY:%s", w306) -> (resulting string=w304:string)  [unwired: 2 in, 1 out]
      }
      event Value Change {
        n77 = event-data() -> ("NewVal"=w317:T26)  [unwired: 3 out]
      }
      event "LOFFN_All": Value Change {
        n78 = event-data() -> ("NewVal"=w326:bool)  [unwired: 1 out]
        n79 = Initialize Array(w326, 8 ("dimension size")) -> (w325:bool[])
        n80 = local write "LOFF_SENSN"(w325) -> ()
      }
      event "LOFFP_All": Value Change {
        n81 = event-data() -> ("NewVal"=w337:bool)  [unwired: 3 out]
        n82 = Initialize Array(w337, 8 ("dimension size")) -> (w336:bool[])
        n83 = local write "LOFF_SENSP"(w336) -> ()
      }
      event "LOFF_FLIP_All": Value Change {
        n84 = event-data() -> ("NewVal"=w348:bool)  [unwired: 1 out]
        n85 = Initialize Array(w348, 8 ("dimension size")) -> (w347:bool[])
        n86 = local write "LOFF_FLIP"(w347) -> ()
      }
      event Value Change {
        n87 = event-data() -> ("OldVal"=w362:T8, "NewVal"=w361:T8)  [unwired: 2 out]
        n88 = call "GPIO_RegChangeID.vi"("GPIO Register New"=w361, "GPIO Register Old"=w362) -> ("GPIO Reg Value"=w359:u32, "Command String"=w360:string)  [unwired: 8 out]
      }
      event "STANDBY", "RESET": Value Change {
        n89 = event-data() -> ("CtlRef"=w375:refnum<vi>, "NewVal"=w376:bool)  [unwired: 2 out]
        n90 = property on="Property Node" class="Bool"(reference=w375) -> ("Label.Text"=w374:string)  [unwired: 1 in, 2 out]
        n91 = To Upper Case(1:w374) -> (0:w369:string)
        n92 = Format Into String(format string="%s", initial string="Device Status:", w369) -> (resulting string=w371:string)  [unwired: 1 in, 1 out]
      }
      event "Plot Selector - Scope", "Plot Selector - Histogram", "Plot Selector - FFT": Value Change {
        n93 = event-data() -> ("CtlRef"=w389:refnum<vi>)  [unwired: 3 out]
        n94 = property on="Property Node" class="Ring (strict)"(reference=w389) -> ("Label.Text"=w388:string)  [unwired: 1 in, 2 out]
        n95 = Scan From String(format string="%[^-]- %s", input string=w388) -> (output 2=w386:string)  [unwired: 2 in, 6 out]
        n96 = Format Into String(format string="%s", initial string="Plot - Update " ("format string"), w386) -> (resulting string=w384:string)  [unwired: 1 in, 1 out]
      }
      event "Refresh_ShadowReg": Value Change {
        n97 = event-data() -> ()  [unwired: 7 out]
      }
      event "Registers Tab": Value Change {
        n98 = event-data() -> ("NewVal"=w409:T2)  [unwired: 6 out]
        n99 = Equal?(x=T25."Register Map" ("Registers Tab"), y=w409) -> (x = y?=w405:bool)
        n100 = Select(t=refnum<class "Internal State Command.lvclass"> refnum ("Internal State Command.lvclass"), s=w405, f=refnum<class "EVMQueueCommand.lvclass"> refnum ("EVMQueueCommand.lvclass")) -> (s? t:f=w408:refnum<class "EVMQueueCommand.lvclass">)
      }
      event "Analysis Control": Value Change {
        n101 = event-data() -> ()  [unwired: 4 out]
      }
      event "Table_Scope", "Table_Histogram", "Table_FFT": Value Change {
        n102 = event-data() -> ("CtlRef"=w428:refnum<vi>)  [unwired: 3 out]
        n103 = property class="Bool"(reference=w428) -> ("Label.Text"=w427:string)  [unwired: 1 in, 2 out]
        n104 = Scan From String(format string="Table_%s", input string=w427) -> (output 1=w425:string)  [unwired: 2 in, 4 out]
      }
      event "Histogram Bins": Value Change {
        n105 = event-data() -> ()  [unwired: 4 out]
      }
      event "Samples/CH": Value Change {
        n106 = event-data() -> ()  [unwired: 7 out]
      }
      event "AinFreq_Desired", "Data Rate": Value Change {
        n107 = event-data() -> ()  [unwired: 7 out]
      }
      event "Input Amplitude(Vpp)": Value Change {
        n108 = event-data() -> ()  [unwired: 4 out]
      }
      event "Show/Poll Lead Off Status": Value Change {
        n109 = event-data() -> ("NewVal"=w470:bool)  [unwired: 3 out]
        n110 = Select(t=TYP_PollingStatus."Resume" ("notification"), s=w470, f=TYP_PollingStatus."Pause" ("notification")) -> (s? t:f=w464:T16)
        n111 = Bundle By Name(cluster=cluster{"State":T16, "Data":i32} {"State"=enum."Pause", "Data"=0}, "State"=w464) -> (w463:cluster{"State":T16, "Data":i32})
        n112 = Send Notification(notification=w463, notifier=w469, error in (no error)=w468) -> ()  [unwired: 2 out]
      }
      event "Save to File": Value Change {
        n113 = event-data() -> ()  [unwired: 4 out]
      }
      event "ADC_Write2ADC": Value Change {
        # "abandoned in place"
        n114 = event-data() -> ("NewVal"=w483:bool)  [unwired: 3 out]
      }
    }
    n115 = call-dynamic "ProcessCommand.vi"("Ctl Refnum"=w84, "Command"=w83, "error in (no error)"=w86, "Data"=w82, "Queue with Cluster Reference"=w80, "EVM Command in"=w81) -> ("error out"=w85:errorcluster)  [unwired: 5 out]
  }
  n116 = while "Update Status Box Message" {
    tunnel: w2 -> [w493]
    tunnel: [w491] -> w32
    shift-right: [w489] -> w31
    shift-left: w24 -> [w494]
    stop <- w490 stop-if-true
    n117 = Wait on Notification(notifier=w493, error in (no error)=w494) -> (notifier out=w491:refnum<notifier>, notification=w492:string, error out=w489:errorcluster)  [unwired: 3 out]
    n118 = case "Check for reserved word \"Exit!\"\nto terminate messaging loop" shown="Default" w492 {
      selector: w492 -> [w495 _]
      tunnel: [FALSE TRUE] -> w490
      frame Default {
        "Status box" <- w495
      }
      frame "Exit!" {
      }
    }
  }
  n119 = while "Plugin Action Loop" {
    shift-right: [w538] -> _
    shift-left: w1 -> [w540]
    shift-right: [w537] -> _
    shift-left: u32[] [] -> [w539]
    shift-right: [w536] -> _
    shift-left: _ -> [w535]
    shift-right: [w505] -> w23
    shift-left: w24 -> [w506]
    shift-right: [w533] -> _
    shift-left: _ -> [w522]
    shift-right: [w534] -> _
    shift-left: _ -> [w532]
    tunnel: w26 -> [w507]
    tunnel: [w521] -> w27
    shift-right: [w530] -> _
    shift-left: _ -> [w531]
    tunnel: w21 -> [w529]
    tunnel: w22 -> [w528]
    tunnel: w2 -> [w527]
    shift-right: [w526] -> _
    shift-left: _ -> [w525]
    shift-right: [w524] -> _
    shift-left: w18 -> [w523]
    tunnel: w20 -> [w520]
    shift-right: [w517] -> _
    shift-left: _ -> [w518]
    shift-right: [w515] -> _
    shift-left: w19 -> [w516]
    tunnel: w16 -> [w512]
    tunnel: w15 -> [w510]
    tunnel: w12 -> [w509]
    tunnel: w5 -> [w508]
    tunnel: w4 -> [w504]
    stop <- w541 stop-if-true
    w502 = FALSE  # Enable Logging?
    # "> Exit Synchronization Ref >"
    # ">References Shifter>"
    # "> Development System? >"
    # "> Base Path >"
    # "> Polling Notifier >"
    # ">Register Map >"
    # "> Main Queue  >"
    # "> Timeout Event >"
    # "> Exit  Event >"
    # "> Messaging Notifier >"
    # ">Update Rate >"
    # ">Acquire - Data Debug Cluster Array>"
    # ">Main Shifter>"
    # ">Channel count>"
    # ">Reference Pointers>"
    # "Analysis Data"
    # ">Acquire - RAW Data>"
    # ">Device Name (estyx root)>"
    n120 = call <userlib>:"DequeueCmd_Cluster.vi"("error in (no error)"=w506, "Queue In"=w507) -> ("error out"=w542:errorcluster, "arg[0]"=w498:string, "command"=w501:string, "queue (dup)"=w503:T31, "arguments"=w499:string[], "Data"=w519:variant)  [unwired: 1 in, 3 out]
    n121 = control-ref of="MainTab"() -> (w513:refnum<vi>)
    n122 = control-ref of="Registers Tab"() -> (w514:refnum<vi>)
    n123 = control-ref of="Analysis Tab"() -> (w511:refnum<vi>)
    n124 = call "LoggingUtil.vi"("Enable"=w502, "Log Item"=w501, "Queue"=w503, "Command"=enum16{"Log", "Terminate"}."Log") -> ()  [unwired: 8 in]
    n125 = case shown="\"Startup Scan\"" w501 {
      selector: w501 -> [_ _ _ _ _ _ _ _ _ _ _ _ _ _ _ _ _ w1088 _ _ _ _ _ _ _ _ _ _ _ _ _ _ _ _ _ _ _ _ _ _ _ _ _ _ _ _ _ _ _ _ _ _ _ _ _ _ w2771 _ _ _ _ _ _ _ _ _ _ _ _ _ _ _ _ _ _ _ _ _ _]
      tunnel: w498 -> [_ _ _ _ _ _ _ _ _ _ _ _ _ _ _ _ _ _ _ _ _ _ _ _ _ _ _ _ _ _ _ w1455 w1535 w1661 _ _ _ _ _ w1963 _ _ _ w2197 _ _ _ _ _ _ _ _ w2530 _ _ _ _ _ _ _ _ _ _ _ w2981 w3012 _ _ _ _ _ w3300 w3329 _ _ w3424 _ _ _]
      tunnel: w542 -> [w553 w561 w594 w607 w676 w694 w740 w770 w822 w853 w870 w909 w937 w949 w959 w973 w1029 w1080 w1105 w1128 w1137 w1156 w1162 w1193 w1219 w1286 w1303 w1319 w1335 w1375 w1385 w1492 _ w1679 w1862 w1886 w1904 w1925 w1939 w1965 w2154 w2171 w2182 w2214 w2231 w2246 w2261 w2293 w2350 w2391 w2446 w2473 w2551 w2601 w2637 w2709 w2785 w2823 w2848 w2861 w2890 w2918 w2952 w2967 w2985 w3016 w3094 w3150 w3220 w3249 w3259 w3312 w3341 w3366 w3407 w3446 w3475 w3513 _]
      tunnel: w503 -> [w554 w562 w588 w608 w680 w695 w735 w777 w823 w838 w888 w914 w933 w950 w960 w1000 w1033 w1079 w1106 w1129 w1138 w1157 w1185 w1194 w1221 w1287 w1301 w1321 w1359 w1376 w1392 w1487 w1554 w1677 w1855 w1887 w1912 w1926 w1940 w1966 w2155 w2172 w2193 w2220 w2232 w2247 w2269 w2294 w2352 w2401 w2447 w2467 w2547 w2602 w2629 w2710 w2786 w2824 w2849 w2873 w2900 w2930 w2953 w2968 w2979 w3018 w3108 w3151 w3221 w3250 w3260 w3313 w3342 w3367 w3415 w3454 w3465 w3514 w3553]
      tunnel: [_ _ _ _ _ _ _ _ _ _ _ _ _ _ _ _ _ _ _ _ _ _ TRUE _ _ _ _ _ _ _ _ _ _ _ _ _ _ _ _ _ _ _ _ _ _ _ _ _ _ _ _ _ _ _ _ _ _ _ _ _ _ _ _ _ _ _ _ _ _ _ _ _ _ _ _ _ _ _ _] -> w541
      tunnel: w540 -> [w557 w569 w602 w622 w683 w703 w747 w780 w830 w864 w891 w917 w945 w957 w971 w978 w1020 w1086 w1109 w1132 w1145 w1160 w1189 w1201 w1230 w1299 w1318 w1333 w1371 w1383 w1411 w1506 w1564 w1690 w1874 w1894 w1921 w1933 w1962 w1988 w2162 w2178 w2196 w2223 w2238 w2253 w2282 w2302 w2375 w2396 w2453 w2487 w2562 w2612 w2652 w2730 w2788 w2833 w2859 w2882 w2909 w2939 w2963 w2975 w2996 w3032 w3113 w3167 w3229 w3253 w3270 w3319 w3348 w3381 w3422 w3461 w3491 w3524 w3556]
      tunnel: w539 -> [w556 w568 w601 w621 w659 w691 w725 w779 w829 w863 w890 w916 _ w956 w970 w1006 w1048 w1085 w1108 w1131 w1144 w1159 w1188 w1200 w1229 w1298 w1317 w1332 w1370 w1382 w1402 w1497 w1556 w1671 w1865 w1893 w1920 w1932 w1961 w1987 w2161 w2177 w2195 w2222 w2237 w2252 w2281 w2301 w2374 w2403 w2452 w2486 w2561 w2611 w2651 w2729 w2787 w2832 w2858 w2881 w2908 w2938 w2962 w2974 w2995 w3031 w3112 w3166 w3228 w3252 w3269 w3318 w3347 w3380 w3421 w3460 w3490 w3523 w3555]
      tunnel: [w557 w569 w602 w622 w683 w703 w747 w780 w830 w864 w891 w917 w945 w957 w971 w978 w1020 w1086 w1109 w1132 w1145 w1160 w1189 w1201 w1230 w1299 w1318 w1333 w1371 w1383 w1411 w1506 w1564 w1690 w1874 w1894 w1921 w1933 w1962 w1988 w2162 w2178 w2196 w2223 w2238 w2253 w2282 w2302 w2375 w2396 w2453 w2487 w2562 w2612 w2652 w2730 w2788 w2833 w2859 w2882 w2909 w2939 w2963 w2975 w2996 w3032 w3113 w3167 w3229 w3253 w3270 w3319 w3348 w3381 w3422 w3461 w3491 w3524 w3556] -> w538
      tunnel: [w556 w568 w601 w621 w659 w691 w723 w779 w829 w863 w890 w916 u32[] [] w956 w970 w1006 w1048 w1085 w1108 w1131 w1144 w1159 w1188 w1200 w1229 w1298 w1317 w1332 w1370 w1382 w1402 w1497 w1556 w1671 w1865 w1893 w1920 w1932 w1961 w1987 w2161 w2177 w2195 w2222 w2237 w2252 w2281 w2301 w2374 w2403 w2452 w2486 w2561 w2611 w2651 w2729 w2787 w2832 w2858 w2881 w2908 w2938 w2962 w2974 w2995 w3031 w3112 w3166 w3228 w3252 w3269 w3318 w3347 w3380 w3421 w3460 w3490 w3523 w3555] -> w537
      tunnel: [w555 w567 w600 w616 w682 w693 w722 w778 w828 w862 w889 w915 w944 w955 w969 w1007 w1049 w1084 w1107 w1130 w1143 w1158 w1187 w1199 w1228 w1297 w1316 w1331 w1369 w1381 w1410 w1505 w1563 w1689 w1873 w1892 w1919 w1931 w1960 w1986 w2160 w2176 w2194 w2221 w2236 w2251 w2272 w2295 w2373 w2402 w2451 w2485 w2560 w2610 w2650 w2728 w2774 w2825 w2857 w2874 w2901 w2931 w2961 w2973 w2994 w3030 w3111 w3165 w3227 w3251 w3268 w3317 w3346 w3379 w3420 w3459 w3489 w3522 w3554] -> w536
      tunnel: w535 -> [w555 w567 w600 w616 w682 w693 _ w778 w828 w862 w889 w915 w944 w955 w969 w1007 w1049 w1084 w1107 w1130 w1143 w1158 w1187 w1199 w1228 w1297 w1316 w1331 w1369 w1381 w1410 w1505 w1563 w1689 w1873 w1892 w1919 w1931 w1960 w1986 w2160 w2176 w2194 w2221 w2236 w2251 w2272 w2295 w2373 w2402 w2451 w2485 w2560 w2610 w2650 w2728 w2774 w2825 w2857 w2874 w2901 w2931 w2961 w2973 w2994 w3030 w3111 w3165 w3227 w3251 w3268 w3317 w3346 w3379 w3420 w3459 w3489 w3522 w3554]
      tunnel: [w552 w562 w587 w620 w671 w695 w737 w775 w823 w834 w887 w913 w932 w950 w960 w999 w1033 w1078 w1104 w1127 w1138 w1155 w1185 w1194 w1220 w1278 w1301 w1323 w1361 w1376 w1394 w1486 w1554 w1677 w1855 w1887 w1911 w1926 w1940 w1966 w2155 w2172 w2185 w2219 w2232 w2247 w2265 w2294 w2364 w2400 w2447 w2466 w2547 w2602 w2635 w2708 w2784 w2824 w2849 w2873 w2900 w2930 w2953 w2968 w2976 w3017 w3108 w3151 w3219 w3248 w3258 w3313 w3342 w3369 w3415 w3454 w3465 w3512 w3552] -> w521
      tunnel: [w551 w561 w586 w619 w669 w694 w736 w774 w822 w833 w886 w912 w931 w949 w959 w998 w1029 w1077 w1103 w1126 w1137 w1154 w1172 w1193 w1203 w1277 w1300 w1322 w1360 w1375 w1393 w1485 w1555 w1678 w1853 w1886 w1910 w1925 w1939 w1965 w2154 w2171 w2186 w2218 w2231 w2246 w2264 w2293 w2365 w2399 w2446 w2459 w2549 w2601 w2636 w2707 w2783 w2823 w2848 w2860 w2889 w2917 w2952 w2967 w2977 w3015 w3093 w3150 w3218 w3247 w3257 w3312 w3341 w3368 w3406 w3445 w3475 w3511 w3551] -> w505
      tunnel: w522 -> [w548 w564 w597 w615 w681 w700 w745 w776 w825 w858 w884 w910 w943 w952 w966 _ w1032 w1083 w1102 w1125 w1141 w1153 w1176 w1196 w1205 w1294 w1310 w1325 w1363 w1378 w1407 w1503 w1561 w1686 w1870 w1889 w1915 w1928 w1957 w1983 w2157 w2170 w2190 w2217 w2235 w2250 w2278 w2298 w2369 w2395 w2445 w2480 w2555 w2607 w2649 w2727 w2780 w2829 w2854 w2878 w2905 w2935 w2958 w2970 w2992 w3019 w3107 w3162 w3226 w3245 w3266 w3311 w3340 w3375 w3414 w3453 w3486 w3520 w3545]
      tunnel: w532 -> [w550 w566 w599 w618 w657 w702 w720 w764 w827 w860 w882 w907 w942 w954 w967 _ w1031 w1082 w1101 w1124 w1140 w1152 w1184 w1198 w1227 w1295 w1315 w1330 w1368 w1380 w1409 w1504 w1562 w1688 w1872 w1891 w1918 w1930 w1959 w1985 w2159 w2175 w2192 w2216 w2234 w2249 w2280 w2300 w2372 w2398 w2450 w2484 w2559 w2609 w2648 w2701 w2782 w2831 w2856 w2880 w2907 w2937 w2960 w2972 w2991 w3029 w3110 w3164 w3225 w3246 w3267 w3316 w3345 w3378 w3419 w3458 w3488 w3521 w3550]
      tunnel: [w548 w564 w597 w615 w681 w700 w745 w776 w825 w857 w884 w910 w943 w952 w966 w1002 w1032 w1083 w1102 w1125 w1141 w1153 w1176 w1196 w1205 w1294 w1310 w1325 w1363 w1378 w1407 w1503 w1561 w1686 w1870 w1889 w1914 w1928 w1957 w1983 w2157 w2170 w2190 w2217 w2235 w2250 w2278 w2298 w2368 w2394 w2445 w2480 w2555 w2607 w2649 w2727 w2780 w2829 w2854 w2878 w2905 w2935 w2958 w2970 w2992 w3019 w3107 w3162 w3226 w3245 w3266 w3311 w3340 w3375 w3414 w3453 w3486 w3520 w3545] -> w533
      tunnel: [w550 w566 w599 w618 w657 w702 w720 w764 w827 w860 w882 w907 w942 w954 w967 w1005 w1031 w1082 w1101 w1124 w1140 w1152 w1184 w1198 w1227 w1295 w1315 w1330 w1368 w1380 w1409 w1504 w1562 w1688 w1872 w1891 w1918 w1930 w1959 w1985 w2159 w2175 w2192 w2216 w2234 w2249 w2280 w2300 w2372 w2398 w2450 w2484 w2559 w2609 w2648 w2701 w2782 w2831 w2856 w2880 w2907 w2937 w2960 w2972 w2991 w3029 w3110 w3164 w3225 w3246 w3267 w3316 w3345 w3378 w3419 w3458 w3488 w3521 w3550] -> w534
      tunnel: [w549 w565 w598 w617 w654 w701 w746 w760 w826 w861 w885 w911 w919 w953 w968 w975 w1024 w1081 w1100 w1123 w1139 w1151 w1183 w1197 w1208 w1296 w1314 w1329 w1367 w1379 w1408 w1496 w1538 w1687 w1871 w1890 w1917 w1929 w1958 w1974 w2158 w2174 w2191 w2215 w2233 w2248 w2271 w2292 w2371 w2380 w2449 w2464 w2528 w2608 w2645 w2703 w2781 w2830 w2855 w2879 w2906 w2936 w2959 w2971 w2990 w3028 w3088 w3149 w3202 w3235 w3261 w3315 w3344 w3377 w3418 w3457 w3474 w3515 w3549] -> w515
      tunnel: w516 -> [w549 w565 w598 w617 w654 w701 w746 w762 w826 w861 w885 w911 w920 w953 w968 w976 w1025 w1081 w1100 w1123 w1139 w1151 w1183 w1197 w1208 w1296 w1314 w1329 w1367 w1379 w1408 w1496 w1538 w1687 w1871 w1890 w1917 w1929 w1958 w1974 w2158 w2174 w2191 w2215 w2233 w2248 w2263 w2292 w2371 w2380 w2449 w2464 w2528 w2608 w2645 w2703 w2781 w2830 w2855 w2879 w2906 w2936 w2959 w2971 w2990 w3028 w3088 w3149 w3203 w3236 w3261 w3315 w3344 w3377 w3418 w3457 w3474 w3515 w3549]
      tunnel: w519 -> [_ _ _ w611 _ _ _ _ _ _ w881 _ _ _ _ _ _ _ _ _ _ _ _ _ _ _ _ _ _ _ _ w1499 w1558 w1682 w1863 _ _ _ _ w1981 _ _ _ w2212 w2230 w2245 _ _ _ _ w2443 w2469 w2550 _ _ _ _ w2821 _ _ _ _ _ _ w2986 w3024 w3105 w3160 w3214 w3239 w3262 w3307 w3336 w3373 w3417 w3456 w3484 w3516 _]
      tunnel: w531 -> [w547 w563 w596 w614 w679 w699 w743 w773 w824 w844 w878 _ w939 w951 w965 _ w1030 w1076 w1094 w1122 w1136 w1150 w1182 w1195 w1226 w1293 w1313 w1328 w1366 w1377 w1406 w1502 w1560 w1685 w1869 w1888 w1908 w1927 w1956 w1984 w2156 w2173 w2183 w2213 w2228 w2243 w2279 w2299 w2363 w2392 w2448 w2483 w2558 w2606 w2653 w2726 w2779 w2828 w2853 w2877 w2904 w2934 w2957 w2969 w2997 w3027 w3109 w3163 w3224 w3244 w3265 w3314 w3343 w3376 w3416 w3455 w3487 w3519 w3548]
      tunnel: [w547 w563 w596 w614 w679 w699 w743 w772 w824 w844 w878 w895 w939 w951 w965 w1001 w1030 w1076 w1094 w1122 w1136 w1150 w1182 w1195 w1226 w1293 w1313 w1328 w1366 w1377 w1406 w1502 w1560 w1685 w1869 w1888 w1908 w1927 w1956 w1984 w2156 w2173 w2183 w2213 w2228 w2243 w2279 w2299 w2363 w2392 w2448 w2483 w2558 w2606 w2653 w2726 w2779 w2828 w2853 w2877 w2904 w2934 w2957 w2969 w2997 w3027 w3109 w3163 w3224 w3244 w3265 w3314 w3343 w3376 w3416 w3455 w3487 w3519 w3548] -> w530
      tunnel: w529 -> [_ _ _ _ _ _ _ _ _ _ _ _ _ _ _ _ _ _ _ _ _ _ w1165 _ _ _ _ _ _ _ _ _ _ _ _ _ _ _ _ _ _ _ _ _ _ _ _ _ _ _ _ _ _ _ _ _ _ _ _ _ _ _ _ _ _ _ _ _ _ _ _ _ _ _ _ _ _ _ _]
      tunnel: w528 -> [_ _ _ _ _ _ _ _ _ _ _ _ _ _ _ _ _ _ _ _ _ _ _ _ _ _ _ _ _ _ _ _ _ _ _ _ _ _ _ _ _ _ _ _ _ _ _ _ _ _ _ _ _ _ _ _ _ _ _ _ _ _ _ _ _ _ _ _ _ _ _ _ _ _ _ _ _ _ _]
      tunnel: w527 -> [_ _ w595 _ w678 _ w742 _ _ w850 _ _ _ _ w961 _ _ _ _ _ _ _ w1163 _ w1222 w1289 _ _ _ _ _ _ _ _ w1854 _ w1906 _ _ w1979 _ _ _ _ _ _ _ _ _ w2379 _ w2477 w2553 _ w2638 _ _ _ _ w2862 w2891 w2916 _ _ _ w3013 _ _ _ _ _ _ _ _ _ _ _ _ _]
      tunnel: [w545 w560 w591 w613 w673 w698 w727 w768 w820 w845 w876 w904 w936 w947 w963 w983 w1047 w1072 w1092 w1119 w1134 w1148 w1180 w1191 w1224 w1291 w1311 w1326 w1364 w1373 w1405 w1501 w1559 w1684 w1868 w1884 w1901 w1923 w1955 w1975 w2152 w2168 w2180 w2210 w2226 w2241 w2274 w2296 w2360 w2388 w2438 w2482 w2557 w2605 w2654 w2725 w2778 w2827 w2852 w2876 w2903 w2933 w2956 w2966 w2998 w3026 w3100 w3153 w3223 w3241 w3256 w3309 w3338 w3371 w3412 w3451 w3477 w3510 w3546] -> w526
      tunnel: w525 -> [w545 w560 w591 w613 w673 w698 w727 w768 w820 w845 w876 w904 w936 w947 w963 w983 _ w1072 w1092 w1119 w1134 w1148 w1180 w1191 w1224 w1291 w1311 w1326 w1364 w1373 w1405 w1501 w1559 w1684 w1868 w1884 w1901 w1923 w1955 w1976 w2152 w2168 w2180 w2210 w2226 w2241 w2274 w2296 w2360 w2388 w2439 w2482 w2557 w2605 w2654 w2725 w2778 w2827 w2852 w2876 w2903 w2933 w2956 w2966 w2998 w3026 w3101 w3152 w3223 w3241 w3256 w3310 w3339 w3372 w3413 w3452 w3476 w3510 w3546]
      tunnel: [w544 w559 w590 w612 w655 w697 w733 w767 w821 w846 w877 w905 w921 w948 w964 w996 w1046 w1073 w1093 w1120 w1135 w1147 w1181 w1192 w1225 w1292 w1312 w1327 w1365 w1374 w1404 w1500 w1537 w1670 w1867 w1885 w1903 w1924 w1954 w1982 w2153 w2169 w2181 w2211 w2227 w2242 w2275 w2297 w2361 w2389 w2444 w2481 w2556 w2604 w2642 w2717 w2772 w2822 w2851 w2872 w2899 w2929 w2955 w2965 w2993 w3025 w3106 w3161 w3222 w3242 w3264 w3308 w3337 w3374 w3411 w3450 w3485 w3518 w3537] -> w524
      tunnel: w523 -> [w544 w559 w590 w612 w656 w697 w733 w767 w821 w846 w877 w905 _ w948 w964 w996 w1046 w1073 w1093 w1120 w1135 w1147 w1181 w1192 w1225 w1292 w1312 w1327 w1365 w1374 w1404 w1500 w1537 w1670 w1867 w1885 w1903 w1924 w1954 w1982 w2153 w2169 w2181 w2211 w2227 w2242 w2275 w2297 w2361 w2389 w2444 w2481 w2556 w2604 w2643 w2718 w2773 w2822 w2851 w2872 w2899 w2929 w2955 w2965 w2993 w3025 w3106 w3161 w3222 w3242 w3264 w3308 w3337 w3374 w3411 w3450 w3485 w3518 w3537]
      tunnel: w520 -> [_ _ w584 _ _ _ _ _ _ _ _ _ w929 _ _ _ _ _ _ _ _ _ w1164 _ _ _ _ _ _ _ _ _ _ _ _ _ _ _ _ _ _ _ _ _ _ _ _ _ _ w2382 _ _ _ _ _ _ _ _ _ _ _ _ _ _ _ w3014 _ _ _ _ _ _ _ _ _ _ _ _ _]
      tunnel: w518 -> [w543 w558 w583 w606 w658 w696 w726 w766 w819 w843 w875 w896 w927 w946 w958 w982 _ w1071 w1091 w1117 w1133 w1146 w1175 w1190 w1218 w1285 w1309 w1324 w1362 w1372 w1403 w1495 w1536 w1683 w1866 w1883 w1898 w1922 w1937 w1977 w2151 w2167 w2179 w2209 w2225 w2240 w2270 w2291 w2355 w2383 w2442 w2472 w2540 w2603 w2655 w2721 w2777 w2826 w2850 w2875 w2902 w2932 w2954 w2964 w2999 w3023 w3104 w3146 w3215 w3240 w3263 w3306 w3335 w3363 w3405 w3440 w3471 w3517 w3536]
      tunnel: [w543 w558 w583 w606 w658 w696 w726 w766 w819 w843 w875 w896 w927 w946 w958 w982 w1042 w1071 w1091 w1117 w1133 w1146 w1175 w1190 w1218 w1285 w1309 w1324 w1362 w1372 w1403 w1495 w1536 w1683 w1866 w1883 w1898 w1922 w1937 w1977 w2151 w2167 w2179 w2209 w2225 w2240 w2270 w2291 w2355 w2383 w2442 w2472 w2540 w2603 w2655 w2721 w2777 w2826 w2850 w2875 w2902 w2932 w2954 w2964 w2999 w3023 w3104 w3146 w3215 w3240 w3263 w3306 w3335 w3363 w3405 w3440 w3471 w3517 w3536] -> w517
      tunnel: w514 -> [_ _ _ _ _ _ _ _ _ _ _ _ _ _ _ _ w1045 _ _ _ _ _ _ _ _ _ _ _ _ _ _ _ _ _ _ _ _ _ _ _ _ _ _ _ _ _ _ _ _ _ _ _ _ _ _ _ _ _ _ _ _ _ _ _ _ _ _ _ _ _ _ _ _ _ _ _ _ _ _]
      tunnel: w513 -> [_ _ _ _ _ _ _ _ _ _ _ _ _ _ _ _ _ _ _ _ _ _ _ _ _ _ _ _ _ _ _ w1459 _ _ _ _ _ _ _ _ _ _ _ _ _ _ _ _ _ _ _ _ _ _ _ _ _ _ _ _ _ _ _ _ _ _ _ _ _ _ _ _ _ _ _ _ _ _ _]
      tunnel: w512 -> [_ _ _ _ _ _ _ _ _ _ _ _ _ _ _ _ _ _ _ _ _ _ _ _ _ _ _ _ _ _ _ _ _ _ _ _ _ _ _ _ _ _ _ _ _ _ w2254 _ _ _ _ _ _ _ _ w2704 _ _ _ _ _ _ _ _ _ _ _ _ w3204 _ _ _ _ _ _ _ _ _ _]
      tunnel: w511 -> [_ _ _ _ _ _ _ _ _ _ _ _ _ _ _ _ w1036 _ _ _ _ _ _ _ _ _ _ _ _ _ _ _ _ _ _ _ _ _ _ _ _ _ _ _ _ _ _ _ _ _ _ _ _ _ _ _ _ _ _ _ _ _ _ _ _ _ _ _ _ _ _ _ _ _ _ _ _ _ _]
      tunnel: w510 -> [_ _ _ _ _ _ _ _ _ _ _ _ _ _ _ _ w1022 _ _ _ _ _ _ _ _ _ _ _ w1356 _ _ _ _ _ _ _ _ _ _ _ _ _ _ _ _ _ _ _ _ _ _ _ _ _ _ _ _ w2811 _ _ _ _ _ _ _ _ _ _ _ _ _ _ _ _ _ _ _ _ _]
      tunnel: w509 -> [_ _ _ _ _ _ _ _ _ _ _ _ _ _ _ _ _ _ _ _ _ _ _ _ _ _ _ _ _ _ _ _ _ _ _ _ _ _ _ _ _ _ _ _ _ _ _ _ _ _ _ _ _ _ _ _ _ _ _ _ _ _ _ _ _ _ _ _ _ _ _ _ _ _ _ _ _ _ _]
      tunnel: w508 -> [_ _ _ _ _ _ _ _ _ _ _ _ _ _ _ _ _ _ _ _ _ _ w1171 _ _ _ _ _ _ _ _ _ _ _ _ _ _ _ _ _ _ _ _ _ _ _ _ _ _ _ _ _ _ _ _ _ _ _ _ _ _ _ _ _ _ _ _ _ _ _ _ _ _ _ _ _ _ _ _]
      tunnel: w504 -> [_ _ _ _ _ _ _ _ _ _ _ _ _ _ _ _ _ _ _ _ _ _ _ _ _ _ _ _ _ _ _ _ _ _ _ _ _ _ _ w1964 _ _ _ _ _ _ _ _ _ _ _ _ _ _ _ _ _ _ _ _ _ _ _ _ _ _ _ _ _ _ _ _ _ _ _ _ _ _ _]
      tunnel: w499 -> [_ _ _ _ _ _ _ _ _ _ _ _ _ _ _ _ _ _ w1090 _ _ _ _ _ _ _ _ _ _ _ _ _ _ _ _ _ _ _ _ _ _ _ _ _ _ _ _ _ _ _ _ _ _ _ _ _ _ _ _ _ _ _ _ _ _ _ _ _ _ _ _ _ _ _ _ _ _ _ _]
      frame "<Blank>" {
        # "1.  Select duplicate case by right clicking on the case selector above.\n2.  Rename the case and add code.\n3.  Rearrange cases as needed."
        # "Use this case as a template to create new cases."
        n126 = call-poly <userlib>:"Enqueue - ClusterQueue.vi"("error in (no error)"=w553, "Command"="Idle", "Queue with Cluster Reference"=w554) -> ("error out"=w551:errorcluster, "Queue Out (dup)"=w552:T31)  [unwired: 3 in, 4 out]
      }
      frame ">-----Acquire Actions-------------------------" {
        # "List separator case"
      }
      frame "Acquire - Stop" {
        w585 = u16 0 items=["Enabled", "Disabled", "Disabled and Grayed"]
        # "Write data file to 0 and stop acquire"
        # "Close data file"
        n127 = Send Notification(notification="Data available" ("Message"), notifier=w595, error in (no error)=w594) -> (error out=w593:errorcluster)  [unwired: 1 out]
        n128 = Unbundle By Name(w597) -> ("Client ptr"=w581:u32, "Data File ptr"=w589:u32)
        n129 = call "lvstyx_close.vi"("error in (no error)"=w593, "file ptr"=w589) -> ("error out"=w580:errorcluster)  [unwired: 9 in]
        n130 = call "FG_ADS1299EVMEstyxFiles.vi"("Storage Info"=TYP_ADS1299Estyx_File_Enum."ads1299evm|data" ("Styx File Tags - Enum")) -> ("File Path"=w577:string)  [unwired: 2 in, 8 out]
        n131 = call-poly "lvstyx_file_write.vi"("error in (no error)"=w580, "buf"="0", "path"=w577, "client ptr"=w581) -> ("error out"=w575:errorcluster, "dup client ptr"=w576:u32)  [unwired: 5 in, 1 out]
        n132 = call "FG_ADS1299EVMEstyxFiles.vi"("Storage Info"=TYP_ADS1299Estyx_File_Enum."ads1299evm|acquire" ("Styx File Tags - Enum")) -> ("File Path"=w573:string)  [unwired: 2 in, 8 out]
        n133 = call-poly "lvstyx_file_write.vi"("error in (no error)"=w575, "boolean"=FALSE, "path"=w573, "client ptr"=w576) -> ("error out"=w572:errorcluster)  [unwired: 6 in, 1 out]
        n134 = local read "Show/Poll Lead Off Status"() -> (w571:bool)
        n135 = case "Enable Polling of Lead-off registers" shown="True" w571 {
          tunnel: w584 -> [_ w605]
          tunnel: w572 -> [_ w603]
          frame False {
          }
          frame True {
            n136 = Send Notification(notification=T15 {"State"=enum."Resume", "Data"=0}, notifier=w605, error in (no error)=w603) -> ()  [unwired: 2 out]
          }
        }
        n137 = call-poly <userlib>:"Enqueue - ClusterQueue.vi"("error in (no error)"=w572, "Data"=w585, "Command"="State - Enable Controls", "Queue with Cluster Reference"=w588) -> ("error out"=w586:errorcluster, "Queue Out (dup)"=w587:T31)  [unwired: 2 in, 4 out]
      }
      frame "Acquire - Update FP" {
        n138 = Variant To Data(Variant=w611, type=TRUE) -> (data=w609:bool)  [unwired: 1 in, 1 out]
        n139 = case "Update the front panel controls/indicators\nTRUE = end of acquisition cycle\nFALSE = get more data" shown="True" w609 {
          tunnel: w608 -> [w627 w633]
          tunnel: [w626 w635] -> w620
          tunnel: [w625 w634] -> w619
          tunnel: w607 -> [w624 w632]
          frame False {
            n140 = call-poly <userlib>:"Enqueue - ClusterQueue.vi"("error in (no error)"=w624, "Command"="Acquire - Get Data", "Queue with Cluster Reference"=w627) -> ("error out"=w625:errorcluster, "Queue Out (dup)"=w626:T31)  [unwired: 2 in, 5 out]
          }
          frame True {
            w629 = T14 0 items=["Enable", "Disable", "Disable/Gray"] ("Disable Property")
            n141 = call-poly <userlib>:"Enqueue - ClusterQueue.vi"("error in (no error)"=w632, "Command"="Analysis - Convert Data", "Queue with Cluster Reference"=w633) -> ("error out"=w630:errorcluster, "Queue Out (dup)"=w631:T31)  [unwired: 2 in, 5 out]
            n142 = property on="Save Data:Volts" class="Bool (strict)"("Disabled"=w629) -> ()  [unwired: 2 in, 2 out]
            n143 = property on="Save Data:Codes" class="Bool (strict)"("Disabled"=w629) -> ()  [unwired: 2 in, 2 out]
            n144 = case "Continuous acquisition mode selected?" shown="True" "Acq - Continuous" {
              tunnel: w631 -> [w640 w645]
              tunnel: w630 -> [w641 w644]
              tunnel: [w638 w643] -> w635
              tunnel: [w637 w642] -> w634
              frame False {
                n145 = call-poly <userlib>:"Enqueue - ClusterQueue.vi"("error in (no error)"=w641, "Command"="Acquire - Stop", "Queue with Cluster Reference"=w640) -> ("error out"=w637:errorcluster, "Queue Out (dup)"=w638:T31)  [unwired: 3 in, 4 out]
              }
              frame True {
                n146 = call-poly <userlib>:"Enqueue - ClusterQueue.vi"("error in (no error)"=w644, "Command"="Acquire Setup - Start", "Queue with Cluster Reference"=w645) -> ("error out"=w642:errorcluster, "Queue Out (dup)"=w643:T31)  [unwired: 3 in, 4 out]
              }
            }
          }
        }
      }
      frame "Acquire - Sort Data" {
        # "Sort Data Into Array and remove status"
        n147 = Send Notification(notification="Sorting Data" ("Message"), notifier=w678, error in (no error)=w676) -> (notifier out=w670:refnum<notifier>, error out=w674:errorcluster)
        n148 = Decimate 1D Array(w659) -> (w662:u32[], w663:u32[], w664:u32[], w665:u32[], w666:u32[], w661:u32[], w660:u32[], w667:u32[], w668:u32[])
        n149 = Build Array(w662, w663, w664, w665, w666, w661, w660, w667, w668) -> (w653:u32[][])
        n150 = Delete From Array(array=w653, index (row)=0) -> (deleted portion=w651:u32[], array with subset deleted=w650:u32[][])  [unwired: 2 in]
        n151 = To Long Integer(number=w651) -> (32bit integer=w647:i32[])
        n152 = To Long Integer(number=w650) -> (32bit integer=w648:i32[][])
        n153 = for "Loop through data sets and compare\n min & max values" {
          tunnel: w648 -> [w685] mode=indexing
          tunnel: [w684] -> w649
          stop <- w684 stop-if-true
          n154 = Array Max & Min(array=w685) -> (max value=w686:i32, min value=w687:i32)  [unwired: 2 out]
          n155 = Equal?(x=w686, y=w687) -> (x = y?=w684:bool)
        }
        n156 = Bundle By Name(cluster=w656, "Data (Codes)"=w648, "Status (Codes)"=w647) -> (w655:T20)
        n157 = call <userlib>:"Enqueue - ClusterBoth.vi"("error in (no error)"=w674, "Data"=TRUE, "Command"="Acquire - Update FP", "Queue with Cluster Reference"=w680) -> ("error out"=w669:errorcluster, "Queue Out (dup)"=w671:T31)  [unwired: 2 in, 4 out]
        n158 = case "Check to see if the min and max value are equal\n(TRUE = error in data read/sort)" shown="True" w649 {
          tunnel: w670 -> [_ w689]
          tunnel: w669 -> [_ w688]
          frame False {
          }
          frame True {
            n159 = Send Notification(notification="Data Capture Error" ("Message"), notifier=w689, error in (no error)=w688) -> ()  [unwired: 2 out]
          }
        }
      }
      frame "Acquire - Write Debug" {
        n160 = case shown="True" FALSE {
          tunnel: w691 -> [_ w707]
          frame False {
          }
          frame True {
            w705 = TRUE ("append to file? (new file:F)")
            n161 = Decimate 1D Array(w707) -> (w710:u32[], w711:u32[], w712:u32[], w713:u32[], w714:u32[], w709:u32[], w708:u32[], w715:u32[], w716:u32[])
            n162 = Build Array(w710, w711, w712, w713, w714, w709, w708, w715, w716) -> (w704:u32[][])
            n163 = call-poly <vilib>:"Write To Spreadsheet File.vi"("transpose? (no:F)"=w705, "format (%d)"="%08x", "append to file? (new file:F)"=w705, "2D data"=w704, "file path (dialog if empty)"=path "C:/Process Raw.txt") -> ()  [unwired: 1 in, 3 out]
          }
        }
      }
      frame "Acquire - Get Data" {
        n164 = Send Notification(notification="Retrieving data" ("Message"), notifier=w742, error in (no error)=w740) -> (error out=w739:errorcluster)  [unwired: 1 out]
        n165 = Unbundle By Name(w745) -> ("Data File ptr"=w744:u32)
        n166 = call "DataStream_Retrieve.vi"("error in (no error)"=w739, "data file pointer"=w744, "transferSize"=256, "no. of channels"=1 ("transferSize")) -> ("error out"=w734:errorcluster, "Debug Data"=w722:cluster{"4byte word":u8[], "word":u32}[], "32bit data"=w724:u32[])  [unwired: 1 in, 1 out]
        n167 = local read "Samples/CH"() -> (w728:u32)
        n168 = Insert Into Array(array=w725, new element=w724) -> (w723:u32[])  [unwired: 1 in]
        n169 = Increment(x=w720) -> (x+1=w721:i32)
        n170 = Multiply(x=w721, y=w728) -> (x*y=w729:u32)
        n171 = Array Size(array=w723) -> (size(s)=w732:i32)
        n172 = Greater?(x=w732, y=w729) -> (0:w738:bool)
        n173 = case shown="True" w738 {
          tunnel: [w752 w754] -> w737
          tunnel: [w751 w757] -> w736
          tunnel: w735 -> [w749 w755]
          tunnel: w734 -> [w748 w756]
          frame False {
            n174 = call <userlib>:"Enqueue - ClusterCommand.vi"("error in (no error)"=w748, "Command"="Acquire - Get Data", "Queue with Cluster Reference"=w749) -> ("error out"=w751:errorcluster, "Queue Out (dup)"=w752:T31)  [unwired: 2 in, 5 out]
          }
          frame True {
            n175 = call-poly <userlib>:"Enqueue - ClusterQueue.vi"("error in"=w756, "Array of Commands"=string[] ["Acquire - Write Debug", "Acquire - Sort Data"], "Queue with Cluster Reference"=w755) -> ("error out"=w757:errorcluster, "Queue (dup)"=w754:T31)  [unwired: 2 in, 5 out]
          }
        }
        n176 = call "EVM_ProgressBar.vi"("Goal points"=w729, "Current points"=w732) -> ("Progress Caption Text"=w730:string, "Progress Value"=w731:dbl)  [unwired: 1 in, 7 out]
        n177 = property on="Progress" class="Slide (strict)"("Value"=w731, "Caption.Text"=w730) -> ()  [unwired: 2 in, 2 out]
      }
      frame "Acquire - Start" {
        n178 = Unbundle By Name(w776) -> ("Client ptr"=w771:u32)
        n179 = call "FG_ADS1299EVMEstyxFiles.vi"("Storage Info"=TYP_ADS1299Estyx_File_Enum."ads1299evm|acquire" ("Styx File Tags - Enum")) -> ("File Path"=w759:string)  [unwired: 2 in, 8 out]
        n180 = call-poly "lvstyx_file_read.vi"("error in (no error)"=w770, "path"=w759, "client ptr"=w771) -> ("error out"=w769:errorcluster, "bool"=w758:bool)  [unwired: 6 in, 1 out]
        n181 = Unbundle By Name(w762) -> ("Acq Timeout"=w763:u16)
        n182 = case "Check if DSP is finished collecting data (acquire = 0)" shown="True" w758 {
          tunnel: w777 -> [w787 w798]
          tunnel: [w785 w801] -> w775
          tunnel: [w784 w800] -> w774
          tunnel: w773 -> [w782 w805]
          tunnel: w769 -> [w783 w803]
          tunnel: [w782 w790] -> w772
          tunnel: w763 -> [w781 w796]
          tunnel: [w781 w789] -> w761
          frame False {
            n183 = call <userlib>:"Enqueue - ClusterCommand.vi"("error in (no error)"=w783, "Command"="Acquire - Get Data", "Queue with Cluster Reference"=w787) -> ("error out"=w784:errorcluster, "Queue Out (dup)"=w785:T31)  [unwired: 2 in, 5 out]
          }
          frame True {
            w802 = 2000  # Divide wait by 2 & convert to msec (/1000)
            # "Limit wait time to 1 msec\n - 2msec due to /2"
            n184 = Decrement(x=w796) -> (x-1=w789:u16)
            n185 = Less?(x=w789, y=0) -> (x < y?=w795:bool)
            n186 = Divide(x=w805, y=w802) -> (x/y=w788:dbl)
            n187 = call <userlib>:"Timer.vi"("error in (no error)"=w803, "Command"=enum16{"Reset", "Get Time", "Check Time"}."Reset") -> ("error out"=w799:errorcluster)  [unwired: 1 in, 8 out]
            n188 = Round Toward +Infinity(x=w788) -> (ceil(x): smallest int >= x=w797:dbl)
            n189 = case shown="True" w795 {
              tunnel: [w811 w813] -> w801
              tunnel: [w810 w814] -> w800
              tunnel: w799 -> [w806 w815]
              tunnel: w798 -> [w809 w818]
              tunnel: w797 -> [w807 w816]
              frame True {
                n190 = One Button Dialog(message="Acquire Error:\nLikely Reason->\nNo DRDY from ADS1299") -> ()  [unwired: 2 out]
                n191 = call <userlib>:"Enqueue - Delayed.vi"("error in (no error)"=w806, "Delay Time (ms)"=w807, "Command"="Command - Stop", "Queue with Cluster Reference"=w809) -> ("error out"=w810:errorcluster, "Queue Out (dup)"=w811:T31)  [unwired: 6 out]
              }
              frame False {
                n192 = call <userlib>:"Enqueue - Delayed.vi"("error in (no error)"=w815, "Delay Time (ms)"=w816, "Command"="Acquire - Start", "Queue with Cluster Reference"=w818) -> ("error out"=w814:errorcluster, "Queue Out (dup)"=w813:T31)  [unwired: 6 out]
              }
            }
            n193 = In Range and Coerce(upper limit=inf ("Positive Infinity"), x=w788, lower limit=2) -> (coerced(x)=w793:dbl)  [unwired: 1 out]
            n194 = To Long Integer(number=w793) -> (32bit integer=w790:i32)
          }
        }
        n195 = Bundle By Name(cluster=w762, "Acq Timeout"=w761) -> (w760:T21)
      }
      frame ">-----Acquire Setup Actions-----------------" {
        # "List separator case"
      }
      frame "Acquire Setup - Open Data File" {
        w859 = u16 1 items=["read"=1, "write"=2, "read/write"=3] ("mode")
        # "open data file"
        # "start acquire"
        n196 = Unbundle By Name(w858) -> ("Client ptr"=w854:u32)
        n197 = call "FG_ADS1299EVMEstyxFiles.vi"("Storage Info"=TYP_ADS1299Estyx_File_Enum."ads1299evm|acquire" ("Styx File Tags - Enum")) -> ("File Path"=w840:string)  [unwired: 2 in, 8 out]
        n198 = call-poly "lvstyx_file_write.vi"("error in (no error)"=w853, "boolean"=TRUE ("Data RCVD"), "path"=w840, "client ptr"=w854) -> ("error out"=w848:errorcluster, "dup client ptr"=w855:u32)  [unwired: 6 in]
        n199 = call <userlib>:"Timer.vi"("error in (no error)"=w848, "Command"=enum16{"Reset", "Get Time", "Check Time"}."Reset") -> ("error out"=w852:errorcluster)  [unwired: 1 in, 8 out]
        n200 = Send Notification(notification="DSP Collecting Data", notifier=w850, error in (no error)=w852) -> (error out=w847:errorcluster)  [unwired: 1 out]
        n201 = call "FG_ADS1299EVMEstyxFiles.vi"("Storage Info"=TYP_ADS1299Estyx_File_Enum."ads1299evm|data" ("Styx File Tags - Enum")) -> ("File Path"=w831:string)  [unwired: 2 in, 8 out]
        n202 = call "lvstyx_open.vi"("error in (no error)"=w847, "mode"=w859, "path"=w831, "client ptr"=w855) -> ("error out"=w835:errorcluster, "file ptr"=w856:u32)  [unwired: 6 in]
        n203 = Bundle By Name(cluster=w858, "Data File ptr"=w856) -> (w857:T32)
        n204 = Divide(x=w844, y=1000.0) -> (x/y=w836:dbl)
        n205 = call <userlib>:"Enqueue - Delayed.vi"("error in (no error)"=w835, "Delay Time (ms)"=w836, "Command"="Acquire - Start", "Queue with Cluster Reference"=w838) -> ("error out"=w833:errorcluster, "Queue Out (dup)"=w834:T31)  [unwired: 6 out]
      }
      frame "Acquire Setup - Setup EVM" {
        w880 = 0  # I32
        # "Write block size"
        # "Zero the data file"
        n206 = Variant To Data(Variant=w881, type=w880) -> (data=w865:i32)  [unwired: 1 in, 1 out]
        n207 = Unbundle By Name(w884) -> ("Client ptr"=w871:u32)
        n208 = call "FG_ADS1299EVMEstyxFiles.vi"("Storage Info"=TYP_ADS1299Estyx_File_Enum."ads1299evm|data" ("Styx File Tags - Enum")) -> ("File Path"=w869:string)  [unwired: 2 in, 8 out]
        n209 = call-poly "lvstyx_file_write.vi"("error in (no error)"=w870, "buf"="0", "path"=w869, "client ptr"=w871) -> ("error out"=w866:errorcluster, "dup client ptr"=w867:u32)  [unwired: 5 in, 1 out]
        n210 = call "FG_ADS1299EVMEstyxFiles.vi"("Storage Info"=TYP_ADS1299Estyx_File_Enum."ads1299evm|blocksize_samples" ("Styx File Tags - Enum")) -> ("File Path"=w872:string)  [unwired: 2 in, 8 out]
        n211 = call-poly "lvstyx_file_write.vi"("error in (no error)"=w866, "int64"=w865, "path"=w872, "client ptr"=w867) -> ("error out"=w879:errorcluster)  [unwired: 6 in, 1 out]
        n212 = call-poly <userlib>:"Enqueue - ClusterQueue.vi"("error in (no error)"=w879, "Command"="Acquire Setup - Open Data File", "Queue with Cluster Reference"=w888) -> ("error out"=w886:errorcluster, "Queue Out (dup)"=w887:T31)  [unwired: 2 in, 5 out]
      }
      frame "Acquire Setup - Acquire calcs" {
        # "Minimum wait time (10ms)"
        # "Calculate data rate"
        # "Pre-Acquisition mode state machine"
        n213 = local read "Data Rate"() -> (w897:dbl)
        n214 = local read "Samples/CH"() -> (w892:u32)
        n215 = Multiply(x=w892, y=u32 9) -> (x*y=w893:u32)
        n216 = Divide(x=w892, y=w897) -> (x/y=w902:dbl)
        n217 = Multiply(x=w902, y=1000.0) -> (x*y=w900:dbl)
        n218 = Round To Nearest(number=w900) -> (nearest integer value=w899:dbl)
        n219 = In Range and Coerce(upper limit=inf ("Positive Infinity"), x=w899, lower limit=10.0) -> (coerced(x)=w906:dbl)  [unwired: 1 out]
        n220 = To Long Integer(number=w906) -> (32bit integer=w895:i32)
        n221 = call <userlib>:"Enqueue - ClusterBoth.vi"("error in (no error)"=w909, "Data"=w893, "Command"="Acquire Setup - Setup EVM", "Queue with Cluster Reference"=w914) -> ("error out"=w912:errorcluster, "Queue Out (dup)"=w913:T31)  [unwired: 2 in, 4 out]
      }
      frame "Acquire Setup - Start" {
        w940 = u16 2 items=["Enabled", "Disabled", "Disabled and Grayed"]
        # "Zero Progress Bar"
        n222 = property on="Progress" class="Slide (strict)"(error in=w937, "Value"=u8 0 ("Collecting")) -> (error out=w928:errorcluster)  [unwired: 1 in, 1 out]
        n223 = Send Notification(notification=T15 {"State"=enum."Pause", "Data"=0} ("PollingNotifier"), notifier=w929, error in (no error)=w928) -> (error out=w923:errorcluster)  [unwired: 1 out]
        n224 = Flush Queue(queue=w933, error in (no error)=w923) -> (queue out=w924:T31, error out=w922:errorcluster)  [unwired: 1 out]
        n225 = call-poly <userlib>:"Enqueue - ClusterQueue.vi"("error in (no error)"=w922, "Command"="Acquire Setup - Acquire calcs", "Queue with Cluster Reference"=w924) -> ("error out"=w934:errorcluster, "Queue Out (dup)"=w935:T31)  [unwired: 2 in, 5 out]
        n226 = call-poly <userlib>:"Enqueue - ClusterQueue.vi"("error in (no error)"=w934, "Data"=w940, "Command"="State - Enable Controls", "Queue with Cluster Reference"=w935) -> ("error out"=w931:errorcluster, "Queue Out (dup)"=w932:T31)  [unwired: 2 in, 4 out]
        n227 = Bundle By Name(cluster=w920, "Acq Timeout"=100 ("AcquireTimeOut")) -> (w919:T21)
        n228 = call "CST_AnalysisData.vi"() -> ("Analysis Data"=w921:T20)  [unwired: 1 out]
      }
      frame ">-----Generic State Machine Actions-------" {
        # "List separator case"
      }
      frame "Idle" {
        # "This case can be used for idle conditions."
        n229 = Send Notification(notification="Ready" ("Message"), notifier=w961, error in (no error)=w959) -> ()  [unwired: 2 out]
      }
      frame "Initialize" {
        w977 = TYP_ADS1299Estyx_File_Enum."|version" ("Styx File Tags - Enum")
        w995 = T14 0 items=["Enable", "Disable", "Disable/Gray"] ("Disable Property")
        w1001 = 1  # Update Rate (ms)
        w1003 = u32 0
        w1005 = 8  # number of channels
        # "Clear Styx History log"
        # "Initalialize Estyx FG"
        # "Initialize/Startup case"
        n230 = Unbundle By Name(w976) -> ("INI Info.Data Dir"=w981:path)
        n231 = call <vilib>:"Check if File or Folder Exists.vi"("error in (no error)"=w973, "path"=w981) -> ("error out"=w986:errorcluster, "file or folder exists?"=w987:bool, "dup path"=w984:path)  [unwired: 7 out]
        n232 = case shown="False" w987 {
          tunnel: w984 -> [w1015 w1017]
          tunnel: w986 -> [w1016 w1018]
          tunnel: [w1014 w1018] -> w985
          tunnel: [w1013 w1017] -> w972
          frame False {
            n233 = Create Folder(path (use dialog)=w1015, error in=w1016) -> (created path=w1013:path, error out=w1014:errorcluster)  [unwired: 2 out]
          }
          frame True {
          }
        }
        n234 = Build Path(base path=w972, name or relative path="Estyx History.txt") -> (appended path=w988:path)
        n235 = while "Create String array of Enum Labels\n (for indexing purposes)" {
          shift-right: [w1009] -> _
          shift-left: w977 -> [w1012]
          tunnel: [w1011] -> w974 mode=indexing
          tunnel: w977 -> [w1008]
          stop <- w1010 continue-if-true
          n236 = Format Into String(w1012) -> (resulting string=w1011:string)  [unwired: 3 in, 1 out]
          n237 = Increment(x=w1012) -> (x+1=w1009:T13)
          n238 = Not Equal?(x=w1009, y=w1008) -> (x != y?=w1010:bool)
        }
        n239 = Write to Text File(file (use dialog)=w988, text="") -> ()  [unwired: 1 in, 4 out]
        n240 = property on="Registers Tab" class="TabCtl (strict)"("Disabled"=w995) -> ()  [unwired: 2 in, 2 out]
        n241 = property on="MainTab" class="TabCtl (strict)"("Disabled"=w995) -> ()  [unwired: 2 in, 2 out]
        n242 = Bundle By Name(cluster=w976, "Styx Enum Strings"=w974) -> (w975:T21)
        n243 = To Upper Case(1:w978) -> (0:w994:string)
        n244 = Unbundle By Name(w975) -> ("INI Info.Startup Dir"=w980:path)
        n245 = Format Into String(format string="%s Styx Index.txt" ("name or relative path"), initial string="", w994) -> (resulting string=w992:string)  [unwired: 1 in, 1 out]
        n246 = call-poly <userlib>:"Enqueue - ClusterQueue.vi"("error in (no error)"=w985, "Command"="State - Load Firmware", "Queue with Cluster Reference"=w1000) -> ("error out"=w998:errorcluster, "Queue Out (dup)"=w999:T31)  [unwired: 2 in, 5 out]
        n247 = Build Path(base path=w980, name or relative path=w992) -> (appended path=w991:path)
        n248 = call "CST_EVM Plugin pointers.vi"() -> ("Pointers"=w1004:T32)  [unwired: 1 out]
        n249 = Bundle By Name(cluster=w1004, "Connection ptr"=w1003, "Client ptr"=w1003, "Data File ptr"=w1003) -> (w1002:T32)
        n250 = call "FG_ADS1299EVMEstyxFiles.vi"("Initialization File Path"=w991) -> ()  [unwired: 2 in, 9 out]
      }
      frame "Startup Scan" {
        # "Populate control reference arranges for managing front panel"
        # "Startup scan to initiailze shift registers based on UI and ini file content"
        n251 = control-ref of="This VI"() -> (w1039:refnum<vi>)
        n252 = invoke on="Invoke Node" class="VI" method="Default Vals.Reinit All"(reference=w1039) -> (error out=w1038:errorcluster)  [unwired: 2 in, 2 out]
        n253 = call "GetCtrlRef[].vi"("error in (no error)"=w1038, "Tab Reference"=w1045) -> ("error out"=w1037:errorcluster, "Page Controls"=w1040:T33, "All Controls in Tab"=w1041:T33)  [unwired: 7 out]
        n254 = call "GetCtrlRef[].vi"("error in (no error)"=w1037, "Tab Reference"=w1036) -> ("Page Controls"=w1034:T33, "All Controls in Tab"=w1035:T33)  [unwired: 8 out]
        n255 = call "CST_1299ShadowRegister.VI"() -> ("DUTRegisters"=w1047:T34, "ShadowReg Reg Refs"=w1043:T33)  [unwired: 1 out]
        n256 = call "CST_CtrlRefShifter.vi"() -> ("App Ctrl Refs"=w1044:T37)  [unwired: 1 out]
        n257 = Bundle By Name(cluster=w1044, "Shadow Regs"=w1043, "Reg - AllCtrls"=w1041, "Reg - PageCtrls"=w1040, "Anlyz - AllCtrls"=w1035, "Anlyz - PageCtrls"=w1034) -> (w1042:T37)
        n258 = Format Into String(format string="%s.ini", w1020) -> (resulting string=w1021:string)  [unwired: 2 in, 1 out]
        n259 = Build Path(base path=w1022, name or relative path=w1021) -> (appended path=w1023:path)
        n260 = call "Startup - Read INI.vi"("error IO"=w1029, "ini path"=w1023) -> ("error out"=w1026:errorcluster, "Key Values"=w1027:string[], "Key Names"=w1028:string[])  [unwired: 7 in]
        n261 = for "Loop through data from INI file and put it into the shift register for access" {
          tunnel: w1028 -> [w1053] mode=indexing
          tunnel: w1027 -> [w1050] mode=indexing
          tunnel: w1026 -> [_]
          shift-right: [w1052] -> w1024
          shift-left: w1025 -> [w1051]
          n262 = case shown="\"DataDir\"" w1053 {
            tunnel: [w1054 w1056 w1061 w1065 w1069] -> w1052
            tunnel: w1051 -> [w1054 w1057 w1062 w1066 w1070]
            tunnel: w1050 -> [_ w1055 w1060 w1064 w1068]
            frame Default {
            }
            frame "Version" {
              n263 = Bundle By Name(cluster=w1057, "INI Info.Version"=w1055) -> (w1056:T21)
            }
            frame "Build" {
              n264 = Decimal String To Number(string=w1060, default (0L)=i16 0 ("default (0 I32)")) -> (number=w1059:i16)  [unwired: 1 in, 1 out]
              n265 = Bundle By Name(cluster=w1062, "INI Info.Build"=w1059) -> (w1061:T21)
            }
            frame "DataDir" {
              n266 = String To Path(string=w1064) -> (path=w1063:path)
              n267 = Bundle By Name(cluster=w1066, "INI Info.Data Dir"=w1063) -> (w1065:T21)
              n268 = property on="Directory to Save Files" class="Path"("StartPath"=w1063, "Value"=w1063) -> ()  [unwired: 2 in, 2 out]
            }
            frame "StartupDir" {
              n269 = String To Path(string=w1068) -> (path=w1067:path)
              n270 = Bundle By Name(cluster=w1070, "INI Info.Startup Dir"=w1067) -> (w1069:T21)
            }
          }
        }
      }
      frame "Developer Error", Default {
        # "Developer Error\n  - This is to warn of typos or invalid cases that have been pushed into the queue."
        n271 = Format Into String(format string="Developer Error...the command \"%s\" is not a valid item" ("initial string"), w1088) -> (resulting string=w1089:string)  [unwired: 2 in, 1 out]
        n272 = One Button Dialog(message=w1089) -> ()  [unwired: 2 out]
        n273 = call-poly <userlib>:"Enqueue - ClusterQueue.vi"("At Front?"=TRUE, "error in (no error)"=w1080, "Command"="Exit" ("Commmand"), "Queue with Cluster Reference"=w1079) -> ("error out"=w1077:errorcluster, "Queue Out (dup)"=w1078:T31)  [unwired: 1 in, 5 out]
      }
      frame "Error" {
        n274 = Index Array(array=w1090, index #2=1 ("index")) -> (element #1=w1097:string, element #2=w1095:string)  [unwired: 1 in]
        n275 = Format Into String(format string="An error occured with error code %s\n%s" ("initial string"), w1097, w1095) -> (resulting string=w1099:string)  [unwired: 2 in, 1 out]
        n276 = One Button Dialog(message=w1099) -> ()  [unwired: 2 out]
        n277 = disable-structure "Enable other diagram to exit plugin\nwhen an error occurs" shown="Enabled" {
          disable-tunnel: w1106 -> [w1114 w1116]
          disable-tunnel: w1105 -> [w1113 w1115]
          disable-tunnel: [w1112 w1116] -> w1104
          disable-tunnel: [w1111 w1115] -> w1103
          frame Disabled {
            n278 = call-poly <userlib>:"Enqueue - ClusterQueue.vi"("error in (no error)"=w1113, "Command"="Exit" ("Commmand"), "Queue with Cluster Reference"=w1114) -> ("error out"=w1111:errorcluster, "Queue Out (dup)"=w1112:T31)  [unwired: 7 in]
          }
          frame Enabled {
          }
        }
      }
      frame "Cancel" {
        # "Use this case for cancelled user prompts or actions"
        n279 = call-poly <userlib>:"Enqueue - ClusterQueue.vi"("At Front?"=TRUE, "error in (no error)"=w1128, "Command"="Exit" ("Commmand"), "Queue with Cluster Reference"=w1129) -> ("error out"=w1126:errorcluster, "Queue Out (dup)"=w1127:T31)  [unwired: 1 in, 5 out]
      }
      frame "About" {
        # "This case can be used to display About Information"
        n280 = One Button Dialog(message="Created by: Me\nModified by:\nDate:\nVersion: 1.0.0.0") -> ()  [unwired: 2 out]
      }
      frame "Update Display" {
        # "Use this case when the front panel needs to be updated"
        n281 = call-poly <userlib>:"Enqueue - ClusterQueue.vi"("error in (no error)"=w1156, "Command"="Idle" ("Commmand"), "Queue with Cluster Reference"=w1157) -> ("error out"=w1154:errorcluster, "Queue Out (dup)"=w1155:T31)  [unwired: 3 in, 4 out]
      }
      frame "Exit" {
        # "Exit Condition\n\nExit Event Loop\n- Inform User Event Capture Loop to exit\n\nExit Message Loop\n- Send \"Exit!\" to Message Loop to exit\n\nExit Polling Loop\n- Stop and Exit Polling Loop"
        # "Wait here until all parallel loops have\nsuccessfully exited before closing\npointers and exiting while loop\n\nExit requires 4 items be ready before final exit:\n1. Messaging/Status Loop\n2. User Interface Capture Loop\n3. Lead-off Polling Loop\n4. Above condition (before closing pointers)"
        # "Sync Point 4"
        n282 = Send Notification(notification=T15 {"State"=enum."Stop", "Data"=0}, notifier=w1164, error in (no error)=w1162) -> (error out=w1166:errorcluster)  [unwired: 1 out]
        n283 = Generate User Event(user event=w1165, event data cluster=TRUE ("event data"), error in=w1166) -> (error out=w1169:errorcluster)  [unwired: 1 out]
        n284 = Send Notification(notification="Exit!", notifier=w1163, error in (no error)=w1169) -> (error out=w1161:errorcluster)  [unwired: 1 out]
        n285 = call <vilib>:"Wait at Rendezvous.vi"("error in (no error)"=w1161, "rendezvous"=w1171) -> ("error out"=w1174:errorcluster)  [unwired: 1 in, 4 out]
        n286 = Unbundle By Name(w1176) -> ("Connection ptr"=w1177:u32, "Client ptr"=w1178:u32)
        n287 = call "lvstyx_close_client.vi"("error in (no error)"=w1174, "client ptr"=w1178) -> ("error out"=w1179:errorcluster)  [unwired: 1 in]
        n288 = call "lvstyx_close_connection.vi"("error in (no error)"=w1179, "connection ptr"=w1177) -> ("error out"=w1173:errorcluster)  [unwired: 1 in]
        n289 = call <vilib>:"Destroy Rendezvous.vi"("error in (no error)"=w1173, "rendezvous"=w1171) -> ("error out"=w1172:errorcluster)  [unwired: 5 out]
      }
      frame ">----- User Menu  Cases -------------------" {
        # "List separator case"
      }
      frame "User Menu - _load_config" {
        # "To Load a configuration file:\n1.  Select configuration file to load.\n2.  Scan through file and write values in file to ADC.\n3.  Read back ADC registers using existing code and update controls."
        n290 = Send Notification(notification="Load Config Settings" ("Message"), notifier=w1222, error in (no error)=w1219) -> (error out=w1214:errorcluster)  [unwired: 1 out]
        n291 = call "File Dialog3"("prompt"="Select the configuration file to load", "error in"=w1214, "pattern (all files)"="*.cfg", "pattern label"="ADS1299EVM Config File") -> ("selected path"=w1210:path, "cancelled"=w1212:bool, "error out"=w1209:errorcluster)  [unwired: 3 in, 6 out]
        n292 = Unbundle By Name(w1209) -> ("status"=w1213:bool)
        n293 = Or(x=w1212, y=w1213) -> (x .or. y?=w1211:bool)
        n294 = Unbundle By Name(w1205) -> ("Client ptr"=w1206:u32)
        n295 = Unbundle By Name(w1208) -> ("Styx Enum Strings"=w1207:string[])
        n296 = case "TRUE = if error OR dialog was canceled\nFALSE = valid file selected (still may be improper format)" shown="False" w1211 {
          tunnel: w1221 -> [w1244 w1273]
          tunnel: [w1243 w1273] -> w1220
          tunnel: w1219 -> [w1242 w1274]
          tunnel: [w1241 w1274] -> w1204
          tunnel: w1210 -> [w1240 _]
          tunnel: w1209 -> [w1239 w1272]
          tunnel: w1207 -> [w1236 _]
          tunnel: w1206 -> [w1235 _]
          tunnel: [w1231 w1272] -> w1202
          frame False {
            n297 = Read from Text File(file (use dialog)=w1240, count=-1, error in=w1239) -> (text=w1237:string[], error out=w1234:errorcluster)  [unwired: 1 in, 2 out]
            n298 = for "Loop through each register setting in the config file and load it to ADC" {
              tunnel: w1237 -> [w1259] mode=indexing
              tunnel: w1236 -> [w1253]
              tunnel: w1235 -> [w1249]
              shift-right: [w1247] -> w1231
              shift-left: w1234 -> [w1248]
              w1254 = 0 ("index (row)")
              # "Parse line into array\n(tab delimited columns)"
              n299 = Spreadsheet String To Array(format string="%s", spreadsheet string=w1259, array type (2D Dbl)="") -> (array=w1256:string[][])  [unwired: 1 in]
              n300 = Index Array(array=w1256, index (row) #1=w1254, index (col) #1=w1254, index (row) #2=w1254, index (col) #2=2 ("disabled index (col)")) -> (element #1=w1246:string, element #2=w1245:string)
              n301 = Search 1D Array(1D array=w1253, element=w1246) -> (index of element=w1250:i32)  [unwired: 1 in]
              n302 = Greater Or Equal To 0?(x=w1250) -> (x >= 0?=w1252:bool)
              n303 = To Variant(anything=w1250) -> (Variant=w1251:variant)
              n304 = case "If register in file matches an existing fw file, write the \nvalue to the file" shown="True" w1252 {
                tunnel: w1245 -> [_ w1270]
                tunnel: w1251 -> [_ w1267]
                tunnel: w1249 -> [_ w1264]
                tunnel: w1248 -> [w1260 w1263]
                tunnel: [w1260 w1262] -> w1247
                frame False {
                }
                frame True {
                  n305 = Variant To Data(Variant=w1267, type=TYP_ADS1299Estyx_File_Enum."conf|ch1set" ("Styx File Tags - Enum")) -> (data=w1266:T13)  [unwired: 1 in, 1 out]
                  n306 = Hexadecimal String To Number(string=w1270, offset=2, default (0uL)=0 ("default (0 U32)")) -> (number=w1261:i32)  [unwired: 1 out]
                  n307 = call "FG_ADS1299EVMEstyxFiles.vi"("Storage Info"=w1266) -> ("File Path"=w1271:string)  [unwired: 2 in, 8 out]
                  n308 = call-poly "lvstyx_file_write.vi"("error in (no error)"=w1263, "int64"=w1261, "path"=w1271, "client ptr"=w1264) -> ("error out"=w1262:errorcluster)  [unwired: 6 in, 1 out]
                }
              }
            }
            n309 = call-poly <userlib>:"Enqueue - ClusterQueue.vi"("error in (no error)"=w1242, "Data"=TRUE, "Command"="State - ReadUserRegisters", "Queue with Cluster Reference"=w1244) -> ("error out"=w1241:errorcluster, "Queue Out (dup)"=w1243:T31)  [unwired: 2 in, 4 out]
          }
          frame True {
          }
        }
        n310 = Merge Errors(w1202, w1204) -> (w1203:errorcluster)
      }
      frame "User Menu - _save_config" {
        # "To save a configuration file:\n1. Specify file name and location \n2. Update the regsiter map table (read all registers values from ADC)\n3. Write configuration file."
        n311 = Send Notification(notification="Saving Settings" ("Message"), notifier=w1289, error in (no error)=w1286) -> ()  [unwired: 2 out]
        n312 = call "File Dialog2"("prompt"="Select the file/location to save the configuation data", "pattern (all files)"="*.cfg", "pattern label"="ADS1299EVM Config File") -> ("selected path"=w1275:path)  [unwired: 4 in, 8 out]
        n313 = call-poly <userlib>:"Enqueue - ClusterQueue.vi"("error in (no error)"=w1286, "Data"=FALSE, "Command"="State - ReadUserRegisters", "Queue with Cluster Reference"=w1287) -> ("error out"=w1276:errorcluster, "Queue Out (dup)"=w1279:T31)  [unwired: 2 in, 4 out]
        n314 = call-poly <userlib>:"Enqueue - ClusterQueue.vi"("error in (no error)"=w1276, "Data"=w1275, "Command"="State - Save Config:ShadowRegister", "Queue with Cluster Reference"=w1279) -> ("error out"=w1277:errorcluster, "Queue Out (dup)"=w1278:T31)  [unwired: 2 in, 4 out]
      }
      frame "User Menu - _capture_image" {
        n315 = control-ref of="This VI"() -> (w1302:refnum<vi>)
        n316 = invoke on="Invoke Node" class="VI" method="FP.Get Image"(reference=w1302) -> ("image data"=w1308:T38)  [unwired: 5 in, 5 out]
        n317 = call "File Dialog"("prompt"="Please select the location of the image file to save/create", "pattern (all files)"="JPEG", "pattern label"="*.jpg") -> ("selected path"=w1304:path)  [unwired: 4 in, 8 out]
        n318 = call <vilib>:"Write JPEG File.vi"("error in (no error)"=w1303, "image data"=w1308, "path to JPEG file"=w1304) -> ("error out"=w1300:errorcluster)  [unwired: 8 out]
      }
      frame "User Menu - _exit_app" {
        n319 = call-poly <userlib>:"Enqueue - ClusterQueue.vi"("error in (no error)"=w1319, "Command"="Exit", "Queue with Cluster Reference"=w1321) -> ("error out"=w1322:errorcluster, "Queue Out (dup)"=w1323:T31)  [unwired: 2 in, 5 out]
      }
      frame "User Menu - _about" {
        w1350 = "ADS1299EVM" ("name or relative path")
        n320 = Build Path(base path=w1356, name or relative path="ADS1299EVM.ini") -> (appended path=w1355:path)
        n321 = call <vilib>:"Open Config Data.vi"("error in (no error)"=w1335, "create file if necessary (T)"=FALSE ("create file if necessary? (T)"), "configuration file path"=w1355) -> ("error out"=w1352:errorcluster, "refnum"=w1353:T39)  [unwired: 6 in, 1 out]
        n322 = call-poly <vilib>:"Read Key.vi"("section"=w1350, "error in (no error)"=w1352, "default value"="X.X.X" ("name or relative path"), "key"="Version" ("name or relative path"), "refnum"=w1353) -> ("error out"=w1349:errorcluster, "value"=w1341:string, "refnum out"=w1348:T39)  [unwired: 1 in, 3 out]
        n323 = call-poly <vilib>:"Read Key.vi"("section"=w1350, "error in (no error)"=w1349, "default value"="Y" ("name or relative path"), "key"="Build" ("name or relative path"), "refnum"=w1348) -> ("error out"=w1345:errorcluster, "value"=w1338:string, "refnum out"=w1346:T39)  [unwired: 1 in, 3 out]
        n324 = call <vilib>:"Close Config Data.vi"("error in (no error)"=w1345, "write file if changed (T)"=FALSE ("write configuration file? (T)"), "refnum"=w1346) -> ("error out"=w1336:errorcluster)  [unwired: 8 out]
        n325 = Format Into String(format string="ADS1299EVM Software\nVersion %s.%s" ("name or relative path"), w1341, w1338) -> (resulting string=w1337:string)  [unwired: 2 in, 1 out]
        n326 = call "Display Message to User"("error in (no error)"=w1336, "Enable"=TRUE, "Message"=w1337) -> ("error out"=w1334:errorcluster)  [unwired: 8 out]
        n327 = call-poly <userlib>:"Enqueue - ClusterQueue.vi"("error in (no error)"=w1334, "Command"="Idle", "Queue with Cluster Reference"=w1359) -> ("error out"=w1360:errorcluster, "Queue Out (dup)"=w1361:T31)  [unwired: 2 in, 5 out]
      }
      frame ">-----Save (File Output) Cases -------" {
        # "List separator case"
      }
      frame "Save to File" {
        n328 = Compound Arithmetic op=OR("Save Analysis:FFT", "Save Analysis:Histogram", "Save Analysis:Scope", "Save Analysis:ShadowRegister") -> (w1390:bool)
        n329 = Compound Arithmetic op=OR("Save Data:Histogram", "Save Data:Codes", "Save Data:FFT", "Save Data:Volts") -> (w1389:bool)
        n330 = Build Array(w1390, w1389) -> (w1395:bool[])
        n331 = call <vilib>:"Check if File or Folder Exists.vi"("error in (no error)"=w1385, "path"="Directory to Save Files") -> ("file or folder exists?"=w1384:bool, "dup path"=w1386:path)  [unwired: 8 out]
        n332 = case "Check for valid directory" shown="True" w1384 {
          tunnel: w1395 -> [_ w1428]
          tunnel: [w1415 w1426] -> w1394
          tunnel: [w1414 w1425] -> w1393
          tunnel: w1392 -> [w1415 w1421]
          tunnel: "Save Analysis:ShadowRegister" -> [_ w1418]
          tunnel: w1386 -> [_ w1417]
          tunnel: w1385 -> [w1414 w1416]
          frame False {
            n333 = local write "Save to File"(FALSE ("Save to File")) -> ()
            n334 = One Button Dialog(message="Invalid Directory - Please try again.") -> ()  [unwired: 2 out]
          }
          frame True {
            n335 = case "Update the Register Table if it is to be saved" shown="True" w1418 {
              tunnel: w1421 -> [w1430 w1436]
              tunnel: [w1430 w1435] -> w1420
              tunnel: w1416 -> [w1429 w1434]
              tunnel: [w1429 w1433] -> w1419
              frame False {
              }
              frame True {
                n336 = call-poly <userlib>:"Enqueue - ClusterQueue.vi"("error in (no error)"=w1434, "Data"=FALSE, "Command"="State - ReadUserRegisters", "Queue with Cluster Reference"=w1436) -> ("error out"=w1433:errorcluster, "Queue Out (dup)"=w1435:T31)  [unwired: 2 in, 4 out]
              }
            }
            n337 = for "Insert case into queue if data or analysis options were selected to save" {
              tunnel: [w1446] -> w1423
              tunnel: w1417 -> [w1444]
              tunnel: w1428 -> [w1437] mode=indexing
              tunnel: w1420 -> [w1440]
              tunnel: string[] ["Analysis", "Data"] -> [w1438] mode=indexing
              shift-right: [w1445] -> w1422
              shift-left: w1419 -> [w1439]
              n338 = Format Into String(format string="%s", initial string="Save Create List:" ("Command"), w1438) -> (resulting string=w1441:string)  [unwired: 1 in, 1 out]
              n339 = case "Enqueue saved case if selected" shown="True" w1437 {
                tunnel: w1440 -> [w1448 w1454]
                tunnel: w1439 -> [w1447 w1453]
                tunnel: w1444 -> [_ w1452]
                tunnel: [w1448 w1451] -> w1446
                tunnel: [w1447 w1450] -> w1445
                tunnel: w1441 -> [_ w1449]
                frame False {
                }
                frame True {
                  n340 = call-poly <userlib>:"Enqueue - ClusterQueue.vi"("error in (no error)"=w1453, "Data"=w1452, "Command"=w1449, "Queue with Cluster Reference"=w1454) -> ("error out"=w1450:errorcluster, "Queue Out (dup)"=w1451:T31)  [unwired: 2 in, 4 out]
                }
              }
            }
            n341 = call-poly <userlib>:"Enqueue - ClusterQueue.vi"("error in (no error)"=w1422, "Data"=w1417, "Command"="Save Clean-up", "Queue with Cluster Reference"=w1423) -> ("error out"=w1425:errorcluster, "Queue Out (dup)"=w1426:T31)  [unwired: 2 in, 4 out]
          }
        }
      }
      frame "Save Create List" {
        w1489 = refnum<vi> refnum  # Page
        # "Create template file containing header info\nFiles will be created as copies of this file and analysis/data added"
        # "Find the 'Save Tab' and get an array of all controls on the tab"
        # "Generate file header"
        n342 = property class="TabCtl (strict)"(reference=w1459) -> ("Pages"=w1457:refnum<vi>[])  [unwired: 1 in, 2 out]
        n343 = Variant To Data(Variant=w1499, type=path "" ("Not A Path Constant")) -> (data=w1482:path)  [unwired: 1 in, 1 out]
        n344 = Get Date/Time String(want seconds? (F)=TRUE) -> (date string=w1479:string, time string=w1480:string)  [unwired: 2 out]
        n345 = for {
          tunnel: w1457 -> [w1508] mode=indexing
          tunnel: [w1507] -> w1458 mode=indexing
          n346 = property class="Page"(reference=w1508) -> ("PageLabel"=w1507:string)  [unwired: 1 in, 2 out]
        }
        n347 = Format Into String(format string="%s %d\n%s\n%s\n\n%s%s", "Record #: " ("string"), "Record ID", "Notes :" ("string"), "User Comments", w1479, w1480) -> (resulting string=w1475:string)  [unwired: 2 in, 1 out]
        n348 = Format Into String(format string="_%d_%s", initial string="Device", "Record ID", "temp.xls" ("format string")) -> (resulting string=w1464:string)  [unwired: 1 in, 1 out]
        n349 = Search 1D Array(1D array=w1458, element="Save") -> (index of element=w1493:i32)  [unwired: 1 out]
        n350 = Build Path(base path=w1482, name or relative path=w1464) -> (appended path=w1463:path)
        n351 = Index Array(array=w1457, index=w1493) -> (element=w1460:refnum<vi>)
        n352 = Open/Create/Replace File(file path (use dialog)=w1463, error in=w1492, operation (0:open)=T27."open or create") -> (refnum out=w1470:refnum<file>, error out=w1469:errorcluster)  [unwired: 4 out]
        n353 = Set File Position(refnum=w1470, from (0:start)=enum16{"start", "end", "current"}."end", error in=w1469) -> (refnum out=w1473:refnum<file>, error out=w1472:errorcluster)  [unwired: 1 in]
        n354 = To More Specific Class(target class=w1489, reference=w1460) -> (specific class reference=w1490:refnum<vi>)  [unwired: 1 in, 1 out]
        n355 = Write to Text File(file (use dialog)=w1473, text=w1475, error in=w1472) -> (refnum out=w1467:refnum<file>, error out=w1468:errorcluster)  [unwired: 2 out]
        n356 = case "Text to check controls for to determine\nif they should be read for save decision" shown="\"Data\"" w1455 {
          tunnel: ["Save Data" ("true string") "Save Analysis" ("true string")] -> w1483
          frame "Data" {
          }
          frame "Analysis", Default {
          }
        }
        n357 = property class="Page"(reference=w1490) -> ("ControlsOnPage"=w1488:refnum<vi>[])  [unwired: 1 in, 2 out]
        n358 = Close File(refnum=w1467, error in=w1468) -> (path=w1491:path, error out=w1484:errorcluster)
        n359 = for "Find controls corresponding to Analysis or Data save and read their condition\nIf control is TRUE, then enter the corresponding function into the queue to save" {
          tunnel: w1491 -> [w1515]
          tunnel: w1488 -> [w1525] mode=indexing
          tunnel: w1487 -> [w1522]
          tunnel: [w1514] -> w1486
          shift-right: [w1513] -> w1485
          shift-left: w1484 -> [w1512]
          tunnel: w1483 -> [w1511]
          n360 = property class="Ctl"(reference=w1525) -> ("Value"=w1520:variant, "Label.Text"=w1523:string)  [unwired: 1 in, 2 out]
          n361 = Match True/False String(2:"", 3:w1511, 4:w1523) -> (0:w1518:bool)  [unwired: 1 out]
          n362 = Variant To Data(Variant=w1520, type=FALSE) -> (error out=w1516:errorcluster, data=w1519:bool)  [unwired: 1 in]
          n363 = call <vilib>:"Clear Errors.vi"("error in (no error)"=w1516) -> ()  [unwired: 7 out]
          n364 = And(x=w1519, y=w1518) -> (x .and. y?=w1517:bool)
          n365 = case "TRUE = save item\nFALSE = do not save item" shown="True" w1517 {
            tunnel: w1523 -> [_ w1534]
            tunnel: w1522 -> [w1527 w1533]
            tunnel: w1515 -> [_ w1532]
            tunnel: [w1527 w1531] -> w1514
            tunnel: w1512 -> [w1526 w1530]
            tunnel: [w1526 w1529] -> w1513
            frame False {
            }
            frame True {
              n366 = call-poly <userlib>:"Enqueue - ClusterQueue.vi"("At Front? (F)"=TRUE, "error in (no error)"=w1530, "Data"=w1532, "Command"=w1534, "Queue with Cluster Reference"=w1533) -> ("error out"=w1529:errorcluster, "Queue Out (dup)"=w1531:T31)  [unwired: 1 in, 4 out]
            }
          }
        }
      }
      frame "Save Analysis" {
        # "Create Filename"
        n367 = Variant To Data(Variant=w1558, type=path "" ("Not A Path Constant")) -> (data=w1539:path)  [unwired: 1 in, 1 out]
        n368 = Strip Path(path=w1539) -> (stripped path=w1548:path, name=w1553:string)
        n369 = Match Pattern(string=w1553, regular expression="_[0-9]+_") -> (before substring=w1551:string, match substring=w1549:string)  [unwired: 3 out]
        n370 = Format Into String(format string="%s%s%s", w1551, w1549, "Analysis.xls") -> (resulting string=w1547:string)  [unwired: 2 in, 1 out]
        n371 = Build Path(base path=w1548, name or relative path=w1547) -> (appended path=w1545:path)
        n372 = call <vilib>:"Check if File or Folder Exists.vi"("path"=w1545) -> ("error out"=w1542:errorcluster, "file or folder exists?"=w1544:bool, "dup path"=w1540:path)  [unwired: 1 in, 7 out]
        n373 = case "Create file if doesn't\nexist" shown="False" w1544 {
          tunnel: [w1656 w1660] -> w1543
          tunnel: w1542 -> [w1655 w1660]
          tunnel: [w1657 w1659] -> w1541
          tunnel: w1540 -> [w1654 w1659]
          tunnel: w1539 -> [w1653 _]
          frame False {
            n374 = Copy(8:w1655, 9:FALSE ("overwrite (F)"), 10:w1654, 11:w1653) -> (0:w1656:errorcluster, 3:w1657:path)  [unwired: 2 out]
          }
          frame True {
          }
        }
        n375 = case "Analysis selected to save" shown="\"FFT\", \"Histogram\", \"Scope\", Default" w1535 {
          selector: w1535 -> [w1569 w1588 w1630]
          tunnel: [w1581 w1613 w1652] -> w1555
          tunnel: w1543 -> [w1580 w1612 w1651]
          tunnel: w1541 -> [w1579 w1611 w1650]
          tunnel: w1537 -> [w1565 w1592 _]
          tunnel: w1536 -> [_ _ w1635]
          frame "CMRR" {
            n376 = Unbundle By Name(w1565) -> ("FFT.CMRR/BW Table"=w1570:string[][][])
            n377 = Open/Create/Replace File(file path (use dialog)=w1579, error in=w1580, operation (0:open)=T27."open or create") -> (refnum out=w1573:refnum<file>, error out=w1574:errorcluster)  [unwired: 4 out]
            n378 = Format Into String(format string="\n\n%s Analysis\n", w1569) -> (resulting string=w1571:string)  [unwired: 2 in, 1 out]
            n379 = Set File Position(refnum=w1573, from (0:start)=enum16{"start", "end", "current"}."end", error in=w1574) -> (refnum out=w1576:refnum<file>, error out=w1575:errorcluster)  [unwired: 1 in]
            n380 = Write to Text File(file (use dialog)=w1576, text=w1571, error in=w1575) -> (refnum out=w1568:refnum<file>, error out=w1567:errorcluster)  [unwired: 2 out]
            n381 = for {
              tunnel: w1570 -> [w1585] mode=indexing
              tunnel: w1568 -> [w1584]
              shift-right: [w1582] -> w1566
              shift-left: w1567 -> [w1582]
              n382 = Refnum to Path(1:w1584) -> (0:w1583:path)
              n383 = call-poly <vilib>:"Write To Spreadsheet File.vi"("format (%s)"="%^s" ("format (%.3f)"), "append to file? (new file:F)"=TRUE, "2D data"=w1585, "file path (dialog if empty)"=w1583) -> ()  [unwired: 2 in, 3 out]
            }
            n384 = Close File(refnum=w1568, error in=w1566) -> (error out=w1581:errorcluster)  [unwired: 1 out]
          }
          frame "FFT", "Histogram", "Scope", Default {
            w1596 = 0 ("index (row)")
            n385 = case shown="\"Scope\", Default" w1588 {
              tunnel: w1592 -> [w1617 w1621 w1622]
              tunnel: [w1616 w1620 w1625] -> w1591
              tunnel: [w1615 w1619 w1624] -> w1590
              tunnel: [w1614 w1618 w1623] -> w1589
              frame "Histogram" {
                n386 = Unbundle By Name(w1617) -> ("Histogram.Analysis Data"=w1616:string[][], "Histogram.Table Row Hdrs"=w1615:string[], "Histogram.Table Col Hdrs"=w1614:string[])
              }
              frame "Scope", Default {
                n387 = Unbundle By Name(w1621) -> ("Scope.Analysis Data"=w1620:string[][], "Scope.Table Row Hdrs"=w1619:string[], "Scope.Table Col Hdrs"=w1618:string[])
              }
              frame "FFT" {
                n388 = Unbundle By Name(w1622) -> ("FFT.Analysis Data"=w1625:string[][], "FFT.Table Row Hdrs"=w1624:string[], "Histogram.Table Col Hdrs"=w1623:string[])
              }
            }
            n389 = Open/Create/Replace File(file path (use dialog)=w1611, error in=w1612, operation (0:open)=T27."open or create") -> (refnum out=w1603:refnum<file>, error out=w1604:errorcluster)  [unwired: 4 out]
            n390 = Set File Position(refnum=w1603, from (0:start)=enum16{"start", "end", "current"}."end", error in=w1604) -> (refnum out=w1608:refnum<file>, error out=w1607:errorcluster)  [unwired: 1 in]
            n391 = Insert Into Array(array=w1591, index (col)=w1596, new element=w1590) -> (w1598:string[][])  [unwired: 1 in]
            n392 = Format Into String(format string="\n\n%s Analysis\n", w1588) -> (resulting string=w1600:string)  [unwired: 2 in, 1 out]
            n393 = Write to Text File(file (use dialog)=w1608, text=w1600, error in=w1607) -> (refnum out=w1605:refnum<file>, error out=w1606:errorcluster)  [unwired: 2 out]
            n394 = Close File(refnum=w1605, error in=w1606) -> (path=w1599:path, error out=w1613:errorcluster)
            n395 = Insert Into Array(array=w1589, index=w1596, new element="") -> (w1595:string[])
            n396 = Insert Into Array(array=w1598, index (row)=w1596, new element=w1595) -> (w1593:string[][])  [unwired: 1 in]
            n397 = call-poly <vilib>:"Write To Spreadsheet File.vi"("format (%s)"="%^s" ("format (%.3f)"), "append to file? (new file:F)"=TRUE, "2D data"=w1593, "file path (dialog if empty)"=w1599) -> ()  [unwired: 2 in, 3 out]
          }
          frame "ShadowRegister" {
            w1633 = refnum<vi> refnum  # Table
            n398 = Unbundle By Name(w1635) -> ("Reg - AllCtrls.References"=w1637:refnum<vi>[], "Reg - AllCtrls.Names/Labels"=w1638:string[])
            n399 = Search 1D Array(1D array=w1638, element=w1630) -> (index of element=w1636:i32)  [unwired: 1 out]
            n400 = Index Array(array=w1637, index=w1636) -> (element=w1634:refnum<vi>)
            n401 = To More Specific Class(target class=w1633, reference=w1634) -> (specific class reference=w1632:refnum<vi>)  [unwired: 1 in, 1 out]
            n402 = Open/Create/Replace File(file path (use dialog)=w1650, error in=w1651, operation (0:open)=T27."open or create") -> (refnum out=w1642:refnum<file>, error out=w1643:errorcluster)  [unwired: 4 out]
            n403 = property class="Tbl"(reference=w1632) -> ("Value"=w1627:string[][], "Column Headers[]"=w1631:string[])  [unwired: 1 in, 2 out]
            n404 = Set File Position(refnum=w1642, from (0:start)=enum16{"start", "end", "current"}."end", error in=w1643) -> (refnum out=w1647:refnum<file>, error out=w1646:errorcluster)  [unwired: 1 in]
            n405 = Insert Into Array(array=w1627, index (row)=0, new element=w1631) -> (w1626:string[][])  [unwired: 1 in]
            n406 = Write to Text File(file (use dialog)=w1647, text="\nADC Register Settings\n\n", error in=w1646) -> (refnum out=w1644:refnum<file>, error out=w1645:errorcluster)  [unwired: 2 out]
            n407 = Close File(refnum=w1644, error in=w1645) -> (path=w1639:path, error out=w1652:errorcluster)
            n408 = call-poly <vilib>:"Write To Spreadsheet File.vi"("format (%s)"="%^s" ("format (%.3f)"), "append to file? (new file:F)"=TRUE, "2D data"=w1626, "file path (dialog if empty)"=w1639) -> ()  [unwired: 2 in, 3 out]
          }
        }
      }
      frame "Save Data" {
        n409 = Variant To Data(Variant=w1682, type=path "" ("Not A Path Constant")) -> (data=w1680:path)  [unwired: 1 in, 1 out]
        n410 = Insert Into Array(array=bool[] [], new element #1="Save_CH1", new element #2="Save_CH2", new element #3="Save_CH3", new element #4="Save_CH4", new element #5="Save_CH5", new element #6="Save_CH6", new element #7="Save_CH7", new element #8="Save_CH8") -> (w1674:bool[])  [unwired: 1 in]
        n411 = call "Create_SaveFile.vi"("File Header Format"="%s Data\n\n" ("format string"), "error in"=w1679, "Operation Type"=w1661, "Template File"=w1680) -> ("error out"=w1672:errorcluster, "refnum out"=w1673:refnum<file>)  [unwired: 6 out]
        n412 = case "Data selected to save" shown="\"Volts\"" w1661 {
          tunnel: w1673 -> [_ w1701 w1735 w1780 w1816]
          tunnel: w1670 -> [_ w1706 w1751 w1786 w1822]
          tunnel: [w1691 w1692 w1750 w1785 w1821] -> w1678
          tunnel: w1674 -> [_ w1705 w1746 w1783 w1819]
          tunnel: w1672 -> [w1691 w1702 w1736 w1779 w1815]
          frame Default {
          }
          frame "Volts" {
            n413 = Unbundle By Name(w1706) -> ("Temp - Data (Volts)"=w1700:dbl[][])
            n414 = for "Select channels to be output" {
              tunnel: w1705 -> [w1713] mode=indexing
              tunnel: w1700 -> [w1716] mode=indexing
              shift-right: [w1718] -> w1699
              shift-left: dbl[][] [] ("Data (Volts)") -> [w1717]
              shift-right: [w1714] -> w1698
              shift-left: "" -> [w1715]
              i -> [w1719]
              n415 = case shown="True" w1713 {
                tunnel: w1719 -> [_ w1729]
                tunnel: [w1721 w1726] -> w1718
                tunnel: w1717 -> [w1721 w1725]
                tunnel: w1716 -> [_ w1724]
                tunnel: w1715 -> [w1720 w1723]
                tunnel: [w1720 w1722] -> w1714
                frame False {
                }
                frame True {
                  n416 = Increment(x=w1729) -> (x+1=w1727:i32)
                  n417 = Insert Into Array(array=w1725, new element=w1724) -> (w1726:dbl[][])  [unwired: 2 in]
                  n418 = Format Into String(format string="CH%d\t", initial string=w1723, w1727) -> (resulting string=w1722:string)  [unwired: 1 in, 1 out]
                }
              }
            }
            n419 = Format Into String(format string="%s\n", w1698) -> (resulting string=w1697:string)  [unwired: 2 in, 1 out]
            n420 = Write to Text File(file (use dialog)=w1701, text=w1697, error in=w1702) -> (refnum out=w1695:refnum<file>, error out=w1694:errorcluster)  [unwired: 2 out]
            n421 = flat-sequence "Write data to file" {
              tunnel: w1699 -> [w1710]
              tunnel: w1695 -> [w1709]
              tunnel: [w1708] -> w1693
              tunnel: w1694 -> [w1708]
              frame #0 {
                w1707 = TRUE ("append to file? (new file:F)")
                n422 = Refnum to Path(1:w1709) -> (0:w1712:path)
                n423 = call-poly <vilib>:"Write To Spreadsheet File.vi"("transpose? (no:F)"=w1707, "format (%.3f)"="%^e", "append to file? (new file:F)"=w1707, "2D data"=w1710, "file path (dialog if empty)"=w1712) -> ()  [unwired: 1 in, 3 out]
              }
            }
            n424 = Close File(refnum=w1695, error in=w1693) -> (error out=w1692:errorcluster)  [unwired: 1 out]
          }
          frame "Codes" {
            # "Include status registers"
            n425 = Unbundle By Name(w1751) -> ("Data (Codes)"=w1748:i32[][], "Status (Codes)"=w1740:i32[])
            n426 = Insert Into Array(array=w1748, index (row)=0, new element=w1740) -> (w1749:i32[][])  [unwired: 1 in]
            n427 = Insert Into Array(array=w1746, index=0, new element=TRUE) -> (w1745:bool[])
            n428 = for "Select channels to be output" {
              tunnel: w1749 -> [w1763] mode=indexing
              tunnel: w1745 -> [w1764] mode=indexing
              shift-right: [w1760] -> w1733
              shift-left: i32[][] [] ("Data (Volts)") -> [w1761]
              shift-right: [w1758] -> w1737
              shift-left: "" -> [w1759]
              i -> [w1762]
              n429 = case "T = output channel, F = don't output channel" shown="True" w1764 {
                tunnel: w1763 -> [_ w1770]
                tunnel: w1762 -> [_ w1773]
                tunnel: w1761 -> [w1766 w1772]
                tunnel: [w1766 w1771] -> w1760
                tunnel: w1759 -> [w1765 w1769]
                tunnel: [w1765 w1767] -> w1758
                frame False {
                }
                frame True {
                  n430 = Not Equal To 0?(x=w1773) -> (x != 0?=w1768:bool)
                  n431 = Insert Into Array(array=w1772, new element=w1770) -> (w1771:i32[][])  [unwired: 2 in]
                  n432 = case shown="True" w1768 {
                    tunnel: ["Status Bits\t" ("format string") w1777] -> w1767
                    tunnel: w1773 -> [_ w1776]
                    tunnel: w1769 -> [_ w1775]
                    frame False {
                    }
                    frame True {
                      n433 = Format Into String(format string="CH%d\t", initial string=w1775, w1776) -> (resulting string=w1777:string)  [unwired: 1 in, 1 out]
                    }
                  }
                }
              }
            }
            n434 = Format Into String(format string="%s\n", w1737) -> (resulting string=w1739:string)  [unwired: 2 in, 1 out]
            n435 = Write to Text File(file (use dialog)=w1735, text=w1739, error in=w1736) -> (refnum out=w1734:refnum<file>, error out=w1731:errorcluster)  [unwired: 2 out]
            n436 = flat-sequence "Write data to file" {
              tunnel: w1734 -> [w1754]
              tunnel: w1733 -> [w1755]
              tunnel: [w1754] -> w1732
              tunnel: w1731 -> [w1753]
              tunnel: [w1753] -> w1730
              frame #0 {
                w1752 = TRUE ("append to file? (new file:F)")
                n437 = Refnum to Path(1:w1754) -> (0:w1757:path)
                n438 = call-poly <vilib>:"Write To Spreadsheet File.vi"("transpose? (no:F)"=w1752, "format (%d)"="%08x", "append to file? (new file:F)"=w1752, "2D data"=w1755, "file path (dialog if empty)"=w1757) -> ()  [unwired: 1 in, 3 out]
              }
            }
            n439 = Close File(refnum=w1732, error in=w1730) -> (error out=w1750:errorcluster)  [unwired: 1 out]
          }
          frame "Histogram" {
            n440 = Unbundle By Name(w1786) -> ("Histogram.Histogram Data"=w1784:T11)
            n441 = for "Select channels to be output" {
              tunnel: w1780 -> [w1796]
              tunnel: w1784 -> [w1793] mode=indexing
              tunnel: w1783 -> [w1794] mode=indexing
              tunnel: [w1789] -> w1782
              shift-right: [w1787] -> w1781
              shift-left: w1779 -> [w1795]
              i -> [w1792]
              n442 = case "Channel selected to save\nTRUE = save channel\nFALSE = don't save channel" shown="True" w1794 {
                tunnel: w1796 -> [w1798 w1808]
                tunnel: w1795 -> [w1797 w1807]
                tunnel: w1793 -> [_ w1802]
                tunnel: w1792 -> [_ w1806]
                tunnel: [w1798 w1804] -> w1790
                tunnel: [w1797 w1803] -> w1788
                frame False {
                }
                frame True {
                  n443 = Unbundle By Name(w1802) -> ("X Values"=w1801:dbl[], "Histogram: h(x)"=w1800:i32[])
                  n444 = Increment(x=w1806) -> (x+1=w1810:i32)
                  n445 = Build Array(w1801, w1800) -> (w1799:dbl[][])
                  n446 = Format Into String(format string="%d\n", initial string="\nCH" ("string"), w1810) -> (resulting string=w1809:string)  [unwired: 1 in, 1 out]
                  n447 = Write to Text File(file (use dialog)=w1808, text=w1809, error in=w1807) -> (refnum out=w1804:refnum<file>, error out=w1803:errorcluster)  [unwired: 2 out]
                  n448 = Refnum to Path(1:w1804) -> (0:w1805:path)
                  n449 = call-poly <vilib>:"Write To Spreadsheet File.vi"("format (%.3f)"="%^e", "append to file? (new file:F)"=TRUE, "2D data"=w1799, "file path (dialog if empty)"=w1805) -> ()  [unwired: 2 in, 3 out]
                }
              }
              n450 = Set File Position(refnum=w1790, from (0:start)=enum16{"start", "end", "current"}."end", error in=w1788) -> (refnum out=w1789:refnum<file>, error out=w1787:errorcluster)  [unwired: 1 out]
            }
            n451 = Close File(refnum=w1782, error in=w1781) -> (error out=w1785:errorcluster)  [unwired: 1 out]
          }
          frame "FFT" {
            n452 = Unbundle By Name(w1822) -> ("FFT.FFT Data"=w1820:cluster{i32, dbl, dbl[]}[])
            n453 = for "Select channels to be output" {
              tunnel: w1816 -> [w1832]
              tunnel: w1820 -> [w1829] mode=indexing
              tunnel: w1819 -> [w1830] mode=indexing
              tunnel: [w1826] -> w1818
              shift-right: [w1824] -> w1817
              shift-left: w1815 -> [w1831]
              i -> [w1828]
              n454 = case "Channel selected to save\nTRUE = save channel\nFALSE = don't save channel" shown="True" w1830 {
                tunnel: w1832 -> [w1834 w1844]
                tunnel: w1831 -> [w1833 w1843]
                tunnel: w1829 -> [_ w1842]
                tunnel: w1828 -> [_ w1839]
                tunnel: [w1834 w1836] -> w1827
                tunnel: [w1833 w1835] -> w1825
                frame False {
                }
                frame True {
                  n455 = Unbundle(w1842) -> (w1841:i32, w1840:dbl, w1838:dbl[])
                  n456 = Increment(x=w1839) -> (x+1=w1846:i32)
                  n457 = Format Into String(format string="%d\nStarting Frequency (Hz) = %d\nIncrement (Hz) = %f\n", initial string="\nCH" ("string"), w1846, w1841, w1840) -> (resulting string=w1845:string)  [unwired: 1 in, 1 out]
                  n458 = Write to Text File(file (use dialog)=w1844, text=w1845, error in=w1843) -> (refnum out=w1836:refnum<file>, error out=w1835:errorcluster)  [unwired: 2 out]
                  n459 = Refnum to Path(1:w1836) -> (0:w1837:path)
                  n460 = call-poly <vilib>:"Write To Spreadsheet File.vi"("format (%.3f)"="%^e", "append to file? (new file:F)"=TRUE, "1D data"=w1838, "file path (dialog if empty)"=w1837) -> ()  [unwired: 2 in, 3 out]
                }
              }
              n461 = Set File Position(refnum=w1827, from (0:start)=enum16{"start", "end", "current"}."end", error in=w1825) -> (refnum out=w1826:refnum<file>, error out=w1824:errorcluster)  [unwired: 1 out]
            }
            n462 = Close File(refnum=w1818, error in=w1817) -> (error out=w1821:errorcluster)  [unwired: 1 out]
          }
        }
      }
      frame "Save Clean-up" {
        n463 = Variant To Data(Variant=w1863, type=path "" ("Not A Path Constant")) -> (data=w1859:path)  [unwired: 1 in, 1 out]
        n464 = List Folder(path=w1859, error in=w1862) -> (filenames=w1861:string[], error out=w1856:errorcluster)  [unwired: 4 out]
        n465 = for "Find template file created" {
          tunnel: w1861 -> [w1880] mode=indexing
          tunnel: [w1880] -> w1860
          tunnel: [w1879] -> w1858
          stop <- w1879 stop-if-true
          n466 = Match Pattern(string=w1880, regular expression="temp") -> (offset past match=w1881:i32)  [unwired: 4 out]
          n467 = Greater Or Equal To 0?(x=w1881) -> (x >= 0?=w1879:bool)
        }
        n468 = Build Path(base path=w1859, name or relative path=w1860) -> (appended path=w1857:path)
        n469 = case "Delete template file if found" shown="True" w1858 {
          tunnel: w1857 -> [_ w1878]
          tunnel: w1856 -> [w1875 w1877]
          tunnel: [w1875 w1876] -> w1853
          frame False {
          }
          frame True {
            n470 = Delete(path (use dialog)=w1878, error in=w1877) -> (error out=w1876:errorcluster)  [unwired: 5 out]
          }
        }
        n471 = Send Notification(notification="Files saved....", notifier=w1854, error in (no error)=w1853) -> ()  [unwired: 2 out]
        n472 = local write "Save to File"(FALSE ("Save to File")) -> ()
      }
      frame ">-----Shell Command Actions----------------" {
        # "List separator case"
      }
      frame "Command - Stop" {
        w1909 = u16 0 items=["Enabled", "Disabled", "Disabled and Grayed"]
        n473 = Send Notification(notification="Connected" ("Status box"), notifier=w1906, error in (no error)=w1904) -> (error out=w1902:errorcluster)  [unwired: 1 out]
        n474 = Unbundle By Name(w1915) -> ("Client ptr"=w1916:u32)
        n475 = call "FG_ADS1299EVMEstyxFiles.vi"("Storage Info"=TYP_ADS1299Estyx_File_Enum."ads1299evm|acquire" ("Styx File Tags - Enum")) -> ("File Path"=w1896:string)  [unwired: 2 in, 8 out]
        n476 = call-poly "lvstyx_file_write.vi"("error in (no error)"=w1902, "boolean"=FALSE, "path"=w1896, "client ptr"=w1916) -> ("error out"=w1907:errorcluster)  [unwired: 6 in, 1 out]
        n477 = Bundle By Name(cluster=w1915, "Data File ptr"=u32 0 ("data file pointer")) -> (w1914:T32)
        n478 = call <userlib>:"Enqueue - ClusterBoth.vi"("At Front? (F)"=TRUE, "error in (no error)"=w1907, "Data"=w1909, "Command"="State - Enable Controls", "Queue with Cluster Reference"=w1912) -> ("error out"=w1910:errorcluster, "Queue Out (dup)"=w1911:T31)  [unwired: 1 in, 4 out]
      }
      frame ">-----User Register Input--------------------" {
        # "List separator case"
      }
      frame "CalculateFin" {
        # "Make sure Tone Bin# is ODD\n(Best if prime)"
        # "Even+1"
        # "Odd"
        n479 = local read "Samples/CH"() -> (w1936:u32)
        n480 = local read "Data Rate"() -> (w1938:dbl)
        n481 = Multiply(x=w1936, y=u32 9) -> (x*y=w1935:u32)
        n482 = Multiply(x="AinFreq_Desired", y=w1935) -> (x*y=w1952:dbl)
        n483 = Divide(x=w1952, y=w1938) -> (x/y=w1950:dbl)
        n484 = Add(x=w1950, y=0.5) -> (x+y=w1951:dbl)
        n485 = Round Toward -Infinity(1:w1951) -> (0:w1943:dbl)
        n486 = Quotient & Remainder(x=w1943, y=2) -> (x-y*floor(x/y)=w1946:dbl)  [unwired: 1 out]
        n487 = Equal To 0?(x=w1946) -> (x = 0?=w1945:bool)
        n488 = Increment(x=w1943) -> (x+1=w1944:dbl)
        n489 = Select(t=w1944, s=w1945, f=w1943) -> (s? t:f=w1953:dbl)
        n490 = Multiply(x=w1938, y=w1953) -> (x*y=w1942:dbl)
        n491 = Divide(x=w1942, y=w1935) -> (x/y=→"AinFreq_Ideal":dbl)
      }
      frame "Update Front Panel" {
        n492 = Unbundle By Name(w1974) -> ("RegMap Data"=w1973:T22[], "Register Names"=w1972:string[])
        n493 = Variant To Data(Variant=w1981, type=u8 0) -> (data=w1968:u8)  [unwired: 1 in, 1 out]
        n494 = Send Notification(notification="Sync Display with Device..." ("Message"), notifier=w1979) -> (notifier out=w1970:refnum<notifier>)  [unwired: 1 in, 1 out]
        n495 = call "Register Set Parse2.vi"("Register Name"=w1963, "Register value"=w1968, "Register Names"=w1972, "RegMap Data"=w1973) -> ("Register Value Array"=w1967:u8[])  [unwired: 1 in, 6 out]
        n496 = case "Select appropriate register to update" shown="\"ID\"" w1963 {
          selector: w1963 -> [_ _ w2000 _ _ _ _ _ _ w2101]
          tunnel: [w1989 w1991 w2006 w2045 w2054 w2068 w2079 w2087 w2097 w2102] -> w1975
          tunnel: w1976 -> [w1989 w1995 w2003 w2047 w2058 w2070 w2080 w2089 w2098 w2103]
          tunnel: w1967 -> [_ w1992 w2004 w2046 w2052 w2066 w2077 w2085 w2095 w2104]
          tunnel: [_ _ errorcluster {"status"=FALSE, "code"=0, "source"=""} ("error out") _ _ _ _ _ _ _] -> w1969
          tunnel: w1966 -> [_ _ _ w2044 _ _ _ _ _ _]
          tunnel: w1965 -> [_ _ _ w2043 _ _ _ _ _ _]
          tunnel: w1964 -> [_ _ _ _ _ _ _ _ _ _]
          frame Default {
          }
          frame "ID" {
            n497 = Index Array(array=w1992, index #2=1 ("index")) -> (element #1=w1994:u8, element #2=w1993:u8)  [unwired: 1 in]
            n498 = in-place "In Place Element Structure" {
              in-place-border: w1994 -> [w1996]
              in-place-border: w1993 -> [w1997]
              n499 = in-place-cluster #1(w1995) -> ()  [unwired: 2 out]
              n500 = in-place-cluster #1("ID.REV_ID"=w1996, "ID.DEV_ID"=w1997) -> (w1991:T34)
              "About_REV_ID" <- w1996
            }
          }
          frame "CH1SET", "CH2SET", "CH3SET", "CH4SET", "CH5SET", "CH6SET", "CH7SET", "CH8SET" {
            n501 = Index Array(array=w2004, index #3=2 ("index")) -> (element #1=w2007:u8, element #2=w2008:u8, element #3=w2009:u8)  [unwired: 2 in]
            n502 = Scan From String(format string="CH%dSET", input string=w2000) -> (output 1=w1998:i32)  [unwired: 2 in, 4 out]
            n503 = call "CST_Reg_CHxSET.vi"() -> ("CH1SET"=w2011:T3)  [unwired: 1 out]
            n504 = Bundle By Name(cluster=w2011, "PD#"=w2007, "GAIN#"=w2008, "MUX#"=w2009) -> (w1999:T3)
            n505 = control-ref of="This VI"() -> (w2001:refnum<vi>)
            n506 = invoke on="Invoke Node" class="VI" method="Ctrl Val.Set"(reference=w2001, "Control Name"=w2000, "Value"=w1999) -> ()  [unwired: 2 in, 5 out]
            n507 = case shown="5" w1998 {
              tunnel: w2003 -> [w2012 w2015 w2018 w2021 w2024 w2027 w2030 w2033 w2036]
              tunnel: [w2012 w2014 w2017 w2020 w2023 w2026 w2029 w2032 w2035] -> w2006
              tunnel: w1999 -> [_ w2013 w2016 w2019 w2022 w2025 w2028 w2031 w2034]
              frame Default {
              }
              frame 1 {
                n508 = Bundle By Name(cluster=w2015, "CH1SET"=w2013) -> (w2014:T34)
              }
              frame 2 {
                n509 = Bundle By Name(cluster=w2018, "CH2SET"=w2016) -> (w2017:T34)
              }
              frame 3 {
                n510 = Bundle By Name(cluster=w2021, "CH3SET"=w2019) -> (w2020:T34)
              }
              frame 4 {
                n511 = Bundle By Name(cluster=w2024, "CH4SET"=w2022) -> (w2023:T34)
              }
              frame 5 {
                n512 = Bundle By Name(cluster=w2027, "CH5SET"=w2025) -> (w2026:T34)
              }
              frame 6 {
                n513 = Bundle By Name(cluster=w2030, "CH6SET"=w2028) -> (w2029:T34)
              }
              frame 7 {
                n514 = Bundle By Name(cluster=w2033, "CH7SET"=w2031) -> (w2032:T34)
              }
              frame 8 {
                n515 = Bundle By Name(cluster=w2036, "CH8SET"=w2034) -> (w2035:T34)
              }
            }
          }
          frame "CONFIG1" {
            n516 = Index Array(array=w2046, index #3=2 ("index")) -> (element #1=w2040:u8, element #2=w2039:u8, element #3=w2038:u8)  [unwired: 2 in]
            n517 = in-place "In Place Element Structure" {
              in-place-border: w2040 -> [w2050]
              in-place-border: w2039 -> [w2049]
              in-place-border: w2038 -> [w2048]
              n518 = in-place-cluster #2(w2047) -> ()  [unwired: 3 out]
              n519 = in-place-cluster #2("Config1.DAISY_EN"=w2050, "Config1.CLK_EN"=w2049, "Config1.DR"=w2048) -> (w2045:T34)
            }
            n520 = Unbundle By Name(w2045) -> ("Config1"=w2042:T6)
            n521 = local write "CONFIG1"(w2042) -> ()
            n522 = call-poly <userlib>:"Enqueue - ClusterQueue.vi"("error in (no error)"=w2043, "Data"=w2042, "Command"="User Input - Update Data Rate", "Queue with Cluster Reference"=w2044) -> ()  [unwired: 2 in, 6 out]
          }
          frame "CONFIG2" {
            n523 = Index Array(array=w2052, index #3=2 ("index")) -> (element #1=w2057:u8, element #2=w2056:u8, element #3=w2055:u8)  [unwired: 2 in]
            n524 = in-place "In Place Element Structure" {
              in-place-border: w2057 -> [w2061]
              in-place-border: w2056 -> [w2059]
              in-place-border: w2055 -> [w2060]
              n525 = in-place-cluster #3(w2058) -> ()  [unwired: 3 out]
              n526 = in-place-cluster #3("Config2.INT_CAL"=w2061, "Config2.CAL_AMP"=w2059, "Config2.CAL_FREQ"=w2060) -> (w2054:T34)
            }
            n527 = Unbundle By Name(w2054) -> ("Config2"=w2053:T5)
            n528 = local write "CONFIG2"(w2053) -> ()
          }
          frame "CONFIG3" {
            n529 = Index Array(array=w2066, index #4=3 ("index")) -> (element #1=w2069:u8, element #2=w2065:u8, element #3=w2064:u8, element #4=w2063:u8)  [unwired: 3 in]
            n530 = in-place "In Place Element Structure" {
              in-place-border: w2069 -> [w2071]
              in-place-border: w2065 -> [w2074]
              in-place-border: w2063 -> [w2072]
              in-place-border: w2064 -> [w2073]
              n531 = in-place-cluster #4(w2070) -> ()  [unwired: 4 out]
              n532 = in-place-cluster #4("Config3.PD_REFBUF"=w2071, "Config3.BIAS_MEAS"=w2074, "Config3.BIASREF_INT"=w2073, "Config3.PD_BIAS"=w2072) -> (w2068:T34)
            }
            n533 = Unbundle By Name(w2068) -> ("Config3"=w2067:T4)
            n534 = local write "CONFIG3"(w2067) -> ()
          }
          frame "CONFIG4" {
            n535 = Index Array(array=w2077, index=0) -> (element=w2075:u8)
            n536 = in-place "In Place Element Structure" {
              in-place-border: w2075 -> [w2081]
              n537 = in-place-cluster #5(w2080) -> ()  [unwired: 1 out]
              n538 = in-place-cluster #5("Config4.PD_LOFF_COMP"=w2081) -> (w2079:T34)
            }
            n539 = Unbundle By Name(w2079) -> ("Config4"=w2078:T10)
            n540 = local write "CONFIG4"(w2078) -> ()
          }
          frame "LOFF" {
            n541 = Index Array(array=w2085, index #3=2 ("index")) -> (element #1=w2088:u8, element #2=w2084:u8, element #3=w2083:u8)  [unwired: 2 in]
            n542 = in-place "In Place Element Structure" {
              in-place-border: w2088 -> [w2090]
              in-place-border: w2084 -> [w2092]
              in-place-border: w2083 -> [w2091]
              n543 = in-place-cluster #6(w2089) -> ()  [unwired: 3 out]
              n544 = in-place-cluster #6("LOFF.COMP_TH"=w2090, "LOFF.ILEAD_OFF"=w2092, "LOFF.FLEAD_OFF"=w2091) -> (w2087:T34)
            }
            n545 = Unbundle By Name(w2087) -> ("LOFF"=w2086:T7)
            n546 = local write "LOFF"(w2086) -> ()
          }
          frame "PACE" {
            n547 = Index Array(array=w2095, index #1=0 ("index")) -> (element #3=w2094:u8)  [unwired: 2 in, 2 out]
            n548 = in-place "In Place Element Structure" {
              in-place-border: w2094 -> [w2099]
              n549 = in-place-cluster #7(w2098) -> ()  [unwired: 1 out]
              n550 = in-place-cluster #7("MISC1.SRB1"=w2099) -> (w2097:T34)
            }
            n551 = Unbundle By Name(w2097) -> ("MISC2"=w2096:T36)
            n552 = local write "MISC1"(w2096) -> ()
          }
          frame "BIAS_SENSN", "BIAS_SENSP", "GPIO", "LOFF_FLIP", "LOFF_SENSN", "LOFF_SENSP", "LOFF_STATN", "LOFF_STATP" {
            n553 = Not Equal To 0?(x=w2104) -> (x != 0?=w2100:bool[])
            n554 = case shown="\"BIAS_SENSP\"" w2101 {
              tunnel: w2103 -> [w2105 w2112 w2126 w2129 w2133 w2137 w2141 w2145 w2149]
              tunnel: w2100 -> [_ w2110 w2125 w2128 w2131 w2135 w2139 w2143 w2147]
              tunnel: [w2105 w2113 w2127 w2130 w2134 w2138 w2142 w2146 w2150] -> w2102
              frame Default {
              }
              frame "GPIO" {
                n555 = control-ref of="GPIO"() -> (w2109:refnum<vi>)
                n556 = property class="Clust (strict)"(reference=w2109) -> ("Controls[]"=w2108:refnum<vi>[])  [unwired: 1 in, 2 out]
                n557 = Split 1D Array(array=w2110, index=4) -> (first subarray=w2107:bool[], second subarray=w2106:bool[])
                n558 = for "Set GPIO value and direction.  Disable/Gray value if GPIO is input" {
                  tunnel: w2108 -> [w2124]
                  tunnel: w2107 -> [w2116] mode=indexing
                  tunnel: w2106 -> [w2118] mode=indexing
                  i -> [w2123]
                  w2114 = T14 2 items=["Enable", "Disable", "Disable/Gray"] ("Disable Property")
                  w2115 = T14 0 items=["Enable", "Disable", "Disable/Gray"] ("Disable Property")
                  n559 = Add(x=w2123, y=4) -> (x+y=w2122:i32)
                  n560 = Index Array(array=w2124, index #1=w2123, index #2=w2122) -> (element #1=w2119:refnum<vi>, element #2=w2120:refnum<vi>)
                  n561 = Select(t=w2114, s=w2116, f=w2115) -> (s? t:f=w2117:T14)
                  n562 = property class="Ctl"(reference=w2120, "Value"=w2118, "Disabled"=w2117) -> ()  [unwired: 1 in, 2 out]
                  n563 = property class="Ctl"(reference=w2119, "Value"=w2116) -> ()  [unwired: 1 in, 2 out]
                }
                n564 = Bundle By Name(cluster=w2112, "GPIO.Direction"=w2107, "GPIO.Data"=w2106) -> (w2113:T34)
              }
              frame "LOFF_STATN" {
                n565 = Bundle By Name(cluster=w2126, "LOFF_STATN"=w2125) -> (w2127:T34)
              }
              frame "LOFF_STATP " {
                n566 = Bundle By Name(cluster=w2129, "LOFF_STATP"=w2128) -> (w2130:T34)
              }
              frame "LOFF_SENSN" {
                n567 = local write "LOFF_SENSN"(w2131) -> ()
                n568 = Bundle By Name(cluster=w2133, "LOFF_SENSN"=w2131) -> (w2134:T34)
                n569 = And Array Elements(Boolean array=w2131) -> (logical AND=w2132:bool)
                n570 = local write "LOFFN_All"(w2132) -> ()
              }
              frame "LOFF_SENSP" {
                n571 = local write "LOFF_SENSP"(w2135) -> ()
                n572 = Bundle By Name(cluster=w2137, "LOFF_SENSP"=w2135) -> (w2138:T34)
                n573 = And Array Elements(Boolean array=w2135) -> (logical AND=w2136:bool)
                n574 = local write "LOFFP_All"(w2136) -> ()
              }
              frame "LOFF_FLIP" {
                n575 = And Array Elements(Boolean array=w2139) -> (logical AND=w2140:bool)
                n576 = local write "LOFF_FLIP"(w2139) -> ()
                n577 = Bundle By Name(cluster=w2141, "LOFF_FLIP"=w2139) -> (w2142:T34)
                n578 = local write "LOFF_FLIP_All"(w2140) -> ()
              }
              frame "BIAS_SENSN" {
                n579 = Bundle By Name(cluster=w2145, "BIASSENSN"=w2143) -> (w2146:T34)
                n580 = And Array Elements(Boolean array=w2143) -> (logical AND=w2144:bool)
                n581 = local write "BIASSENSN"(w2143) -> ()
                n582 = local write "BIASSENSN_All"(w2144) -> ()
              }
              frame "BIAS_SENSP" {
                n583 = Bundle By Name(cluster=w2149, "BIASSENSP"=w2147) -> (w2150:T34)
                n584 = And Array Elements(Boolean array=w2147) -> (logical AND=w2148:bool)
                n585 = local write "BIASSENSP_All"(w2148) -> ()
                n586 = local write "BIASSENSP"(w2147) -> ()
              }
            }
          }
        }
        n587 = Send Notification(notification="Sync Complete...Ready" ("Message"), notifier=w1970, error in (no error)=w1969) -> ()  [unwired: 2 out]
      }
      frame ">-----Plugin State Actions--------------------" {
        # "List separator case"
      }
      frame "Read Version Info" {
        n588 = Unbundle By Name(w2170) -> ("Client ptr"=w2165:u32)
        n589 = call "FG_ADS1299EVMEstyxFiles.vi"("Storage Info"=TYP_ADS1299Estyx_File_Enum."|version" ("Styx File Tags - Enum")) -> ("File Path"=w2164:string)  [unwired: 2 in, 8 out]
        n590 = call-poly "lvstyx_file_read.vi"("path"=w2164, "client ptr"=w2165) -> ("buf"=→"About_FW_Ver":string)  [unwired: 7 in, 2 out]
      }
      frame "State - Connected" {
        n591 = call <userlib>:"Enqueue - ClusterCommand.vi"("error in (no error)"=w2182, "Command"="State - Initialize", "Queue with Cluster Reference"=w2193) -> ("error out"=w2187:errorcluster, "Queue Out (dup)"=w2188:T31)  [unwired: 2 in, 5 out]
        n592 = call <userlib>:"Enqueue - ClusterCommand.vi"("error in (no error)"=w2187, "Command"="State - Initialize2", "Queue with Cluster Reference"=w2188) -> ("error out"=w2186:errorcluster, "Queue Out (dup)"=w2185:T31)  [unwired: 2 in, 5 out]
      }
      frame "State - Delayed Insert" {
        n593 = Variant To Data(error in=w2214, Variant=w2212, type=1.0 ("Wait Time (s)")) -> (error out=w2198:errorcluster, data=w2200:dbl)
        n594 = call <userlib>:"Timer.vi"("error in (no error)"=w2198, "Command"=enum16{"Reset", "Get Time", "Check Time"}."Check Time", "Wait Time (s)"=w2200) -> ("error out"=w2203:errorcluster, "Time Expired?"=w2204:bool)  [unwired: 7 out]
        n595 = Concatenate Strings("State - Delayed Insert:", w2197) -> (w2202:string)
        n596 = Select(t=w2197, s=w2204, f=w2202) -> (s? t:f=w2205:string)
        n597 = call <userlib>:"CST_Queue.vi"() -> ("Queue Cluster Element"=w2207:T40)  [unwired: 1 out]
        n598 = Bundle By Name(cluster=w2207, "Data"=w2212, "Command"=w2205) -> (w2206:T40)
        n599 = Enqueue Element At Opposite End(queue=w2220, element=w2206, error in (no error)=w2203) -> (queue out=w2219:T31, error out=w2218:errorcluster)  [unwired: 2 out]
      }
      frame "State - Enable Controls" {
        w2229 = u16 2 items=["Enabled", "Disabled", "Disabled and Grayed"]
        n600 = Variant To Data(Variant=w2230, type=w2229) -> (data=w2224:u16)  [unwired: 1 in, 1 out]
        n601 = property on="MainTab" class="TabCtl (strict)"("Disabled"=w2224) -> ()  [unwired: 2 in, 2 out]
        n602 = property on="Registers Tab" class="TabCtl (strict)"("Disabled"=w2224) -> ()  [unwired: 2 in, 2 out]
      }
      frame "State - Enable Print" {
        w2244 = u16 2 items=["Enabled", "Disabled", "Disabled and Grayed"]
        n603 = Variant To Data(Variant=w2245, type=w2244) -> (data=w2239:u16)  [unwired: 1 in, 1 out]
        n604 = property on="Save Analysis:Scope" class="Bool (strict)"("Disabled"=w2239) -> ()  [unwired: 2 in, 2 out]
        n605 = property on="Save Analysis:FFT" class="Bool (strict)"("Disabled"=w2239) -> ()  [unwired: 2 in, 2 out]
        n606 = property on="Save Analysis:Histogram" class="Bool (strict)"("Disabled"=w2239) -> ()  [unwired: 2 in, 2 out]
        n607 = property on="Save Data:Histogram" class="Bool (strict)"("Disabled"=w2239) -> ()  [unwired: 2 in, 2 out]
        n608 = property on="Save Data:FFT" class="Bool (strict)"("Disabled"=w2239) -> ()  [unwired: 2 in, 2 out]
        n609 = property on="Save Data:Codes" class="Bool (strict)"("Disabled"=w2239) -> ()  [unwired: 2 in, 2 out]
        n610 = property on="Save Data:Volts" class="Bool (strict)"("Disabled"=w2239) -> ()  [unwired: 2 in, 2 out]
      }
      frame "State - Initialize" {
        w2255 = 4.5  # Vref
        w2256 = 2048000.0  # fCLK
        w2276 = u16 0 items=["Enabled", "Disabled", "Disabled and Grayed"]
        # "Initialize the control window"
        n611 = Unbundle By Name(w2263) -> ("INI Info.Startup Dir"=w2262:path)
        n612 = Build Path(base path=w2262, name or relative path="ADS1299 Register Map.txt") -> (appended path=w2259:path)
        n613 = call "RegisterMap_ADSxxxx.vi"("error in (no error)"=w2261, "Register Map File"=w2259) -> ("error out"=w2260:errorcluster, "Register Names"=w2258:string[], "ADSxxxx Register Data"=w2257:T22[])  [unwired: 7 in]
        n614 = call <userlib>:"Enqueue - ClusterBoth.vi"("error in (no error)"=w2260, "Command"="State - Reconcile Registers", "Queue with Cluster Reference"=w2269) -> ("error out"=w2267:errorcluster, "Queue Out (dup)"=w2268:T31)  [unwired: 3 in, 4 out]
        n615 = call <userlib>:"Enqueue - ClusterBoth.vi"("error in (no error)"=w2267, "Data"=w2276, "Command"="State - Enable Controls", "Queue with Cluster Reference"=w2268) -> ("error out"=w2264:errorcluster, "Queue Out (dup)"=w2265:T31)  [unwired: 2 in, 4 out]
        n616 = Bundle By Name(cluster=w2263, "RegMap Data"=w2257, "Register Names"=w2258, "f(CLK)"=w2256, "Vref"=w2255, "Word Bits"=w2254) -> (w2271:T21)
      }
      frame "State - Reconcile Registers" {
        w2286 = string[] ["ID", "LOFF_STATP", "LOFF_STATN", "GPIO", "MISC2"]  # Registers to ignore error when reconciling
        # "Test register controls to make sure typdefs match the register map."
        n617 = Unbundle By Name(w2291) -> ("Reg - AllCtrls.References"=w2289:refnum<vi>[], "Reg - AllCtrls.Names/Labels"=w2290:string[])
        n618 = Unbundle By Name(w2292) -> ("Register Names"=w2284:string[], "RegMap Data"=w2287:T22[])
        n619 = for "Loop through each register from register map file and reconcile number of controls with groups in register definition" {
          tunnel: w2284 -> [w2314] mode=indexing
          tunnel: w2287 -> [w2315] mode=indexing
          tunnel: w2290 -> [w2320]
          tunnel: w2289 -> [w2319]
          shift-right: [w2304] -> w2285
          shift-left: bool[] [] -> [w2316]
          tunnel: w2286 -> [w2313]
          # "Replace FALSE with TRUE for registers\nto be ignored"
          n620 = Search 1D Array(1D array=w2313, element=w2314) -> (index of element=w2309:i32)  [unwired: 1 out]
          n621 = Search 1D Array(1D array=w2320, element=w2314) -> (index of element=w2318:i32)  [unwired: 1 out]
          n622 = Less Than 0?(x=w2318) -> (x < 0?=w2317:bool)
          n623 = Unbundle By Name(w2315) -> ("Item Count"=w2305:u8)
          n624 = case "FALSE = Control found that matches register name\nTRUE = no control" shown="False" w2317 {
            tunnel: w2319 -> [w2328 _]
            tunnel: w2318 -> [w2327 _]
            tunnel: w2305 -> [w2326 _]
            tunnel: w2316 -> [w2322 w2345]
            tunnel: [w2323 w2346] -> w2311
            frame False {
              n625 = Index Array(array=w2328, index=w2327) -> (element=w2325:refnum<vi>)
              n626 = property class="Gen"(reference=w2325) -> (reference out=w2324:refnum<vi>, "ClassName"=w2321:string)  [unwired: 1 in, 1 out]
              n627 = case "Reconcile control & register accordingly\n  - Cluster -> compare number of controls & functional groups\n  - Array -> compare # functional groups to # bits\n  - Default -> don't add anything" shown="\"Cluster\"" w2321 {
                tunnel: w2326 -> [_ w2334 w2343]
                tunnel: w2324 -> [_ w2333 _]
                tunnel: [w2329 w2332 w2342] -> w2323
                tunnel: w2322 -> [w2329 w2331 w2341]
                frame Default {
                }
                frame "Cluster" {
                  w2337 = refnum<vi> refnum  # Cluster
                  n628 = To More Specific Class(target class=w2337, reference=w2333) -> (specific class reference=w2338:refnum<vi>)  [unwired: 1 in, 1 out]
                  n629 = property class="Clust"(reference=w2338) -> ("Controls[]"=w2336:refnum<vi>[])  [unwired: 1 in, 2 out]
                  n630 = Array Size(array=w2336) -> (size(s)=w2335:i32)
                  n631 = Equal?(x=w2335, y=w2334) -> (x = y?=w2330:bool)
                  n632 = Insert Into Array(array=w2331, new element=w2330) -> (w2332:bool[])  [unwired: 1 in]
                }
                frame "Array" {
                  w2339 = 8  # #bits in control register
                  n633 = Equal?(x=w2339, y=w2343) -> (x = y?=w2340:bool)
                  n634 = Insert Into Array(array=w2341, new element=w2340) -> (w2342:bool[])  [unwired: 1 in]
                }
              }
            }
            frame True {
              n635 = Insert Into Array(array=w2345, new element=FALSE ("new element/subarray")) -> (w2346:bool[])  [unwired: 1 in]
            }
          }
          n636 = Array Size(array=w2311) -> (size(s)=w2307:i32)
          n637 = Greater Or Equal To 0?(x=w2309) -> (x >= 0?=w2310:bool)
          n638 = Decrement(x=w2307) -> (x-1=w2306:i32)
          n639 = Select(t=w2306, s=w2310, f=w2309) -> (s? t:f=w2308:i32)
          n640 = Replace Array Subset(array=w2311, new element=TRUE, index=w2308) -> (w2304:bool[])
        }
        n641 = And Array Elements(Boolean array=w2285) -> (logical AND=w2283:bool)
        n642 = case "Display warning if all registers do pass test" shown="False" w2283 {
          frame False {
            n643 = One Button Dialog(message="Register controls and register map do not match. \nVerify the correct register settings/definitions.") -> ()  [unwired: 2 out]
          }
          frame True {
          }
        }
      }
      frame "State - Initialize2" {
        w2347 = T14 2 items=["Enable", "Disable", "Disable/Gray"] ("Disable Property")
        # "Initialize the control window"
        n644 = call-poly <userlib>:"Enqueue - ClusterQueue.vi"("error in (no error)"=w2350, "Data"=w2347, "Command"="State - Enable Print", "Queue with Cluster Reference"=w2352) -> ("error out"=w2349:errorcluster, "Queue Out (dup)"=w2351:T31)  [unwired: 2 in, 4 out]
        n645 = call-poly <userlib>:"Enqueue - ClusterQueue.vi"("error in (no error)"=w2349, "Command"="Read Version Info", "Queue with Cluster Reference"=w2351) -> ("error out"=w2358:errorcluster, "Queue Out (dup)"=w2357:T31)  [unwired: 2 in, 5 out]
        n646 = Bundle By Name(cluster=w2369, "Data File ptr"=u32 0 ("data file pointer")) -> (w2368:T32)
        n647 = local read "CONFIG1"() -> (w2353:T6)
        n648 = call-poly <userlib>:"Enqueue - ClusterQueue.vi"("error in (no error)"=w2358, "Data"=w2353, "Command"="User Input - Update Data Rate", "Queue with Cluster Reference"=w2357) -> ("error out"=w2366:errorcluster, "Queue Out (dup)"=w2367:T31)  [unwired: 2 in, 4 out]
        n649 = call-poly <userlib>:"Enqueue - ClusterQueue.vi"("error in (no error)"=w2366, "Data"=TRUE ("At Front?"), "Command"="State - ReadUserRegisters", "Queue with Cluster Reference"=w2367) -> ("error out"=w2365:errorcluster, "Queue Out (dup)"=w2364:T31)  [unwired: 2 in, 4 out]
      }
      frame "State - Load Firmware" {
        n650 = Current VI's Path() -> (path=w2387:path)
        n651 = property class="App"() -> ("App.Kind"=w2377:T18)  [unwired: 2 in, 2 out]
        n652 = property on="Property Node" class="App"() -> ("App.Kind"=w2386:T18)  [unwired: 2 in, 2 out]
        n653 = Strip Path(path=w2387) -> (stripped path=w2385:path)  [unwired: 1 out]
        n654 = case shown="\"Run Time System\"" w2377 {
          tunnel: ["fw\\ads1299evm-pdk.bin" ("name or relative path") "fw_1299\\ads1299evm-pdk.bin" ("name or relative path")] -> w2376
          frame "Run Time System" {
          }
          frame "Development System", Default {
          }
        }
        n655 = case shown="\"Run Time System\"" w2386 {
          tunnel: w2385 -> [w2433 w2435]
          tunnel: [w2433 w2434] -> w2384
          frame "Development System", Default {
          }
          frame "Run Time System" {
            n656 = Strip Path(path=w2435) -> (stripped path=w2434:path)  [unwired: 1 out]
          }
        }
        n657 = Build Path(base path=w2384, name or relative path=w2376) -> (appended path=w2397:path)
        n658 = call "Plugin FWLoader_A.vi"("error in (no error)"=w2391, "Firmware file"=w2397, "Messaging Notifier"=w2379) -> ("error out"=w2390:errorcluster, "client ptr"=w2381:i32, "connection ptr"=w2393:i32, "Connected"=w2378:bool)  [unwired: 1 in]
        n659 = case "Firmware Load Success\nTRUE = continue\nFALSE = failed" shown="False" w2378 {
          tunnel: w2401 -> [w2419 w2432]
          tunnel: [w2413 w2431] -> w2400
          tunnel: [w2411 w2430] -> w2399
          tunnel: w2395 -> [w2420 w2429]
          tunnel: [w2420 w2428] -> w2394
          tunnel: w2393 -> [_ w2427]
          tunnel: w2390 -> [w2418 w2425]
          tunnel: w2382 -> [_ w2424]
          tunnel: w2381 -> [_ w2421]
          tunnel: w2379 -> [w2417 _]
          frame False {
            w2408 = "Exit" ("T button name (\"OK\")")
            n660 = Send Notification(notification="Connection Failure", notifier=w2417) -> ()  [unwired: 1 in, 2 out]
            n661 = Two Button Dialog(message="Connection and FW Load Failed!\nPlease check your connections/configuration and try again", 1:w2408, 2:"Retry" ("T button name (\"OK\")")) -> (T button?=w2409:bool)
            n662 = Flush Queue(queue=w2419, error in (no error)=w2418) -> (queue out=w2414:T31, error out=w2412:errorcluster)  [unwired: 1 out]
            n663 = Select(t="State - Load Firmware" ("T button name (\"OK\")"), s=w2409, f=w2408) -> (s? t:f=w2410:string)
            n664 = call-poly <userlib>:"Enqueue - ClusterQueue.vi"("error in (no error)"=w2412, "Command"=w2410, "Queue with Cluster Reference"=w2414) -> ("error out"=w2411:errorcluster, "Queue Out (dup)"=w2413:T31)  [unwired: 2 in, 5 out]
          }
          frame True {
            n665 = Bundle By Name(cluster=T15 {"State"=enum."Init", "Data"=0} ("PollingNotifier"), "Data"=w2421) -> (w2423:T15)
            n666 = Bundle By Name(cluster=w2429, "Connection ptr"=w2427, "Client ptr"=w2421) -> (w2428:T32)
            n667 = Send Notification(notification=w2423, notifier=w2424) -> ()  [unwired: 1 in, 2 out]
            n668 = call <userlib>:"Enqueue - ClusterCommand.vi"("error in (no error)"=w2425, "Command"="State - Connected", "Queue with Cluster Reference"=w2432) -> ("error out"=w2430:errorcluster, "Queue Out (dup)"=w2431:T31)  [unwired: 2 in, 5 out]
          }
        }
      }
      frame "State - Update Status Info" {
        n669 = Variant To Data(Variant=w2443, type=T28 {"LOFF_STATP"=[], "LOFF_STATN"=[]} ("output cluster")) -> (data=w2440:T28)  [unwired: 1 in, 1 out]
        n670 = Unbundle By Name(w2440) -> ("LOFF_STATP"=w2437:bool[], "LOFF_STATN"=w2436:bool[])
        n671 = Bundle By Name(cluster=w2439, "LOFF_STATP"=w2437, "LOFF_STATN"=w2436) -> (w2438:T34)
      }
      frame "State - ReadUserRegisters" {
        w2456 = T13[] [enum."conf|reset", enum."conf|sleep"] items=["|version", "|id", "ads1299evm|blocksize_samples", "ads1299evm|acquire", "ads1299evm|data", "conf|ch1set", "conf|ch2set", "conf|ch3set", "conf|ch4set", "conf|ch5set", "conf|ch6set", "conf|ch7set", "conf|ch8set", "conf|config1", "conf|config2", "conf|config3", "conf|devid", "conf|gpio", "conf|loff", "conf|loffflip", "conf|loffsensn", "conf|loffsensp", "conf|loffstatn", "conf|loffstatp", "conf|misc2", "conf|misc1", "conf|biassensn", "conf|biassensp", "conf|reset", "conf|sleep", "conf|config4", "led|dp", "led|seg", "led|ch", "mmb0|pll", "mmb0|clkout", "mmb0|clkfreq"]  # Do not add info from these files to shift register (table)
        n672 = Variant To Data(Variant=w2469, type=FALSE) -> (data=w2465:bool)  [unwired: 1 in, 1 out]
        n673 = Send Notification(notification="Reading Registers..." ("Message"), notifier=w2477, error in (no error)=w2473) -> (notifier out=w2474:refnum<notifier>, error out=w2476:errorcluster)
        n674 = Unbundle By Name(w2480) -> ("Client ptr"=w2479:u32)
        n675 = while "Read data from estyx registers and send to correct \"Update Front Panel\" action" {
          tunnel: w2479 -> [w2512]
          tunnel: w2476 -> [w2503]
          tunnel: [w2499] -> w2461
          shift-right: [w2509] -> _
          shift-left: TYP_ADS1299Estyx_File_Enum."conf|ch1set" ("Styx File Tags - Enum") -> [w2495]
          tunnel: w2467 -> [w2502]
          tunnel: [w2501] -> w2466
          tunnel: w2465 -> [w2500]
          tunnel: w2456 -> [w2496]
          shift-right: [w2494] -> w2454
          shift-left: cluster{"String":string, "uint32":u32}[] [] -> [w2493]
          i -> [w2511]
          stop <- w2507 stop-if-true
          # "Update progress bar"
          # "> loop through estyx files >"
          n676 = call "EVM_ProgressBar.vi"("Goal points"=u32 20, "Current points"=w2511) -> ("Progress Caption Text"=w2513:string, "Progress Value"=w2514:dbl)  [unwired: 1 in, 7 out]
          n677 = property on="Progress" class="Slide (strict)"("Value"=w2514, "Caption.Text"=w2513) -> ()  [unwired: 2 in, 2 out]
          n678 = call "FG_ADS1299EVMEstyxFiles.vi"("Storage Info"=w2495) -> ("File Path"=w2489:string)  [unwired: 2 in, 8 out]
          n679 = call-poly "lvstyx_file_read.vi"("path"=w2489, "client ptr"=w2512) -> ("uint32"=w2488:u32)  [unwired: 7 in, 2 out]
          n680 = call "Convert_Styx2Register.vi"("Styx File Tags - Enum"=w2495) -> ("String"=w2498:string)  [unwired: 1 in, 9 out]
          n681 = Increment(x=w2495) -> (x+1=w2509:T13)
          n682 = Greater?(x=w2509, y=TYP_ADS1299Estyx_File_Enum."conf|config4") -> (0:w2507:bool)
          n683 = Format Into String(format string=":%s", initial string="Update Front Panel" ("Message"), w2498) -> (resulting string=w2497:string)  [unwired: 1 in, 1 out]
          n684 = Bundle("String"=w2498, "uint32"=w2488) -> (w2492:cluster{"String":string, "uint32":u32})  [unwired: 1 out]
          n685 = Search 1D Array(1D array=w2496, element=w2495) -> (index of element=w2491:i32)  [unwired: 1 out]
          n686 = case "Update UI control\nTRUE = update\nFALSE = no update (update table only)" shown="True" w2500 {
            tunnel: w2503 -> [w2519 w2526]
            tunnel: w2497 -> [_ w2525]
            tunnel: w2488 -> [_ w2524]
            tunnel: w2502 -> [w2520 w2523]
            tunnel: [w2520 w2522] -> w2501
            tunnel: [w2519 w2521] -> w2499
            frame False {
            }
            frame True {
              n687 = call-poly <userlib>:"Enqueue - ClusterQueue.vi"("error in (no error)"=w2526, "Data"=w2524, "Command"=w2525, "Queue with Cluster Reference"=w2523) -> ("error out"=w2521:errorcluster, "Queue Out (dup)"=w2522:T31)  [unwired: 2 in, 4 out]
            }
          }
          n688 = Less Than 0?(x=w2491) -> (x < 0?=w2490:bool)
          n689 = case "Add if a control register" shown="True" w2490 {
            tunnel: [w2515 w2518] -> w2494
            tunnel: w2493 -> [w2515 w2517]
            tunnel: w2492 -> [_ w2516]
            frame False {
            }
            frame True {
              n690 = Insert Into Array(array=w2517, new element=w2516) -> (w2518:cluster{"String":string, "uint32":u32}[])  [unwired: 1 in]
            }
          }
          n691 = Wait (ms)(milliseconds to wait=u32 10) -> ()  [unwired: 1 out]
        }
        n692 = Unbundle By Name(w2464) -> ("RegMap Data"=w2463:T22[], "Register Names"=w2462:string[])
        n693 = call "Format_RegisterTable.vi"("Register Names"=w2462, "RegMap Data"=w2463, "error in (no error)"=w2461, "Register Data Array"=w2454) -> ("error out"=w2460:errorcluster, "Register Table"=→"ShadowRegister":string[][])  [unwired: 1 in, 5 out]
        n694 = Send Notification(notification="Registers Read Complete" ("Message"), notifier=w2474, error in (no error)=w2460) -> (error out=w2459:errorcluster)  [unwired: 1 out]
        n695 = property on="Progress" class="Slide (strict)"(error in=w2459, "Value"=u8 0 ("Collecting"), "Caption.Text"="0%") -> ()  [unwired: 1 in, 2 out]
      }
      frame "State - Save Config" {
        w2545 = refnum<vi> refnum  # Table
        # "Get register map control and data"
        n696 = Variant To Data(Variant=w2550, type=path "") -> (data=w2539:path)  [unwired: 1 in, 1 out]
        n697 = Unbundle By Name(w2540) -> ("Reg - AllCtrls.References"=w2542:refnum<vi>[], "Reg - AllCtrls.Names/Labels"=w2541:string[])
        n698 = Send Notification(notification="Writing Config to File..." ("Message"), notifier=w2553, error in (no error)=w2551) -> (notifier out=w2531:refnum<notifier>, error out=w2538:errorcluster)
        n699 = Search 1D Array(1D array=w2541, element=w2530) -> (index of element=w2543:i32)  [unwired: 1 out]
        n700 = Index Array(array=w2542, index=w2543) -> (element=w2544:refnum<vi>)
        n701 = To More Specific Class(target class=w2545, reference=w2544) -> (specific class reference=w2546:refnum<vi>)  [unwired: 1 in, 1 out]
        n702 = property class="Tbl"(reference=w2546) -> ("Value"=w2529:string[][])  [unwired: 1 in, 2 out]
        n703 = Unbundle By Name(w2528) -> ("Styx Enum Strings"=w2527:string[])
        n704 = Open/Create/Replace File(file path (use dialog)=w2539, error in=w2538, operation (0:open)=T27."replace or create") -> (refnum out=w2536:refnum<file>, error out=w2535:errorcluster)  [unwired: 3 in, 1 out]
        n705 = for "Save configuration data to file" {
          tunnel: w2536 -> [w2587]
          tunnel: w2535 -> [w2588]
          tunnel: [w2583] -> w2533
          tunnel: [w2582] -> w2534
          tunnel: w2529 -> [w2575] mode=indexing
          tunnel: w2527 -> [w2569]
          w2565 = string[] ["loffstatp", "loffstatn"]  # Read only registers
          # "compare enum strings with register map registers and write data if matches"
          n706 = Index Array(array=w2575, index #3=2 ("index")) -> (element #1=w2572:string, element #2=w2574:string, element #3=w2573:string)  [unwired: 2 in]
          n707 = To Lower Case(string=w2572) -> (all lower case string=w2576:string)
          n708 = Search and Replace String(replace all?=TRUE ("replace all? (F)"), input string=w2576, search string="_", replace string="") -> (result string=w2566:string)  [unwired: 4 in, 3 out]
          n709 = Format Into String(format string="%s", initial string="conf|", w2566) -> (resulting string=w2568:string)  [unwired: 1 in, 1 out]
          n710 = Match First String(2:w2565, 3:w2566) -> (0:w2564:i32)  [unwired: 1 out]
          n711 = Search 1D Array(1D array=w2569, element=w2568) -> (index of element=w2581:i32)  [unwired: 1 in]
          n712 = Set File Position(refnum=w2587, from (0:start)=enum16{"start", "end", "current"}."end", error in=w2588) -> (refnum out=w2585:refnum<file>, error out=w2584:errorcluster)  [unwired: 1 in]
          n713 = Less Than 0?(x=w2564) -> (x < 0?=w2563:bool)
          n714 = Greater Than 0?(x=w2581) -> (x > 0?=w2589:bool)
          n715 = And(x=w2589, y=w2563) -> (x .and. y?=w2567:bool)
          n716 = case "Write to config file if matches AND\nnot read-only register" shown="True" w2567 {
            tunnel: w2585 -> [w2591 w2595]
            tunnel: w2584 -> [w2590 w2596]
            tunnel: w2574 -> [_ w2600]
            tunnel: w2568 -> [_ w2599]
            tunnel: w2573 -> [_ w2598]
            tunnel: [w2591 w2593] -> w2583
            tunnel: [w2590 w2592] -> w2582
            frame False {
            }
            frame True {
              n717 = Format Into String(format string="%s\t%s\t%s\n", w2599, w2600, w2598) -> (resulting string=w2594:string)  [unwired: 2 in, 1 out]
              n718 = Write to Text File(file (use dialog)=w2595, text=w2594, error in=w2596) -> (refnum out=w2593:refnum<file>, error out=w2592:errorcluster)  [unwired: 1 in, 1 out]
            }
          }
        }
        n719 = Close File(refnum=w2533, error in=w2534) -> (error out=w2532:errorcluster)  [unwired: 1 out]
        n720 = Send Notification(notification="Config File Written" ("Message"), notifier=w2531, error in (no error)=w2532) -> (error out=w2549:errorcluster)  [unwired: 1 out]
      }
      frame ">---Analysis---------" {
        # "List separator case"
      }
      frame "Analysis - Convert Data" {
        w2613 = T41 {"Cutoff"=0.0, "Order"=0} ("Filter Settings")
        n721 = local read "Analysis Control"() -> (w2621:enum32{"Scope", "Histogram", "FFT"})
        n722 = Format Into String(initial string="Calculating ..." ("Message"), w2621) -> (resulting string=w2639:string)  [unwired: 2 in, 1 out]
        n723 = Send Notification(notification=w2639, notifier=w2638, error in (no error)=w2637) -> (error out=w2633:errorcluster)  [unwired: 1 out]
        n724 = Bundle By Name(cluster=w2613, "Cutoff"="LPF Cutoff", "Order"="LPF Order") -> (w2623:T41)
        n725 = Bundle By Name(cluster=w2613, "Cutoff"="HPF Cutoff", "Order"="HPF Order") -> (w2622:T41)
        n726 = local read "Samples/CH"() -> (w2644:u32)
        n727 = Unbundle By Name(w2643) -> ("Data (Codes)"=w2647:i32[][])
        n728 = Unbundle By Name(w2645) -> ("Word Bits"=w2615:i32, "Vref"=w2614:dbl)
        n729 = local read "Data Rate"() -> (w2628:dbl)
        n730 = for {
          tunnel: w2647 -> [w2667] mode=indexing
          shift-right: [w2672] -> w2641
          shift-left: ext[][] [] -> [w2673]
          tunnel: w2644 -> [w2684]
          tunnel: w2628 -> [w2668]
          tunnel: w2623 -> [w2666]
          tunnel: w2622 -> [w2665]
          tunnel: w2621 -> [w2664]
          tunnel: "Notch Freq" -> [w2663]
          tunnel: "Notch Order" -> [w2662]
          tunnel: "LPF Enable" -> [w2661]
          tunnel: "Notch Enable" -> [w2660]
          tunnel: "HPF Enable" -> [w2659]
          tunnel: w2615 -> [w2657]
          tunnel: w2614 -> [w2656]
          i -> [w2683]
          n731 = case shown="\"Scope\"" w2664 {
            tunnel: w2667 -> [w2686 w2696]
            tunnel: [w2685 w2695] -> w2658
            tunnel: w2668 -> [_ w2694]
            tunnel: w2663 -> [_ w2693]
            tunnel: w2662 -> [_ w2692]
            tunnel: w2666 -> [_ w2691]
            tunnel: w2665 -> [_ w2690]
            tunnel: w2661 -> [_ w2689]
            tunnel: w2660 -> [_ w2688]
            tunnel: w2659 -> [_ w2687]
            frame Default {
              n732 = To Double Precision Float(number=w2686) -> (double precision float=w2685:dbl[])
            }
            frame "Scope" {
              n733 = call "Filter_3Way.vi"("Data IN"=w2696, "DataRate (SPS)"=w2694, "Low Pass Filter Settings"=w2691, "High Pass Filter Settings"=w2690, "Notch Filter"=w2693, "Notch Order"=w2692, "LPF Enable"=w2689, "50/60 Notch Enable"=w2688, "HPF Enable"=w2687) -> ("Data OUT"=w2695:dbl[])  [unwired: 6 in]
            }
          }
          n734 = Increment(x=w2683) -> (x+1=w2682:i32)
          n735 = Array Subset(array=w2658, length=w2684) -> (w2675:dbl[])  [unwired: 1 in]
          n736 = control-ref of="This VI"() -> (w2680:refnum<vi>)
          n737 = Format Into String(format string="CH%dSET" ("initial string"), w2682) -> (resulting string=w2679:string)  [unwired: 2 in, 1 out]
          n738 = invoke on="Invoke Node" class="VI" method="Ctrl Val.Get"(reference=w2680, "Control Name"=w2679) -> ("Get Control Value Variant"=w2677:variant)  [unwired: 2 in, 3 out]
          n739 = call "CST_Reg_CHxSET.vi"() -> ("CH1SET"=w2678:T3)  [unwired: 1 out]
          n740 = Variant To Data(Variant=w2677, type=w2678) -> (data=w2676:T3)  [unwired: 1 in, 1 out]
          n741 = Unbundle By Name(w2676) -> ("GAIN#"=w2674:enum16{"1", "2", "4", "6", "8", "12", "24"})
          n742 = call "2'scomplementPGAconv.vi"("Normalize Data"="Normalize Data", "VREF Ratio"=1.0, "RefVoltage"=w2656, "Bits"=w2657, "GAIN#"=w2674, "Data In"=w2675) -> ("Data Out"=w2671:dbl[])  [unwired: 5 in]
          n743 = Insert Into Array(array=w2673, new element=w2671) -> (w2672:ext[][])  [unwired: 2 in]
        }
        n744 = Format Into String(format string="%s", initial string="Analysis - ", w2621) -> (resulting string=w2630:string)  [unwired: 1 in, 1 out]
        n745 = call-poly <userlib>:"Enqueue - ClusterQueue.vi"("At Front? (F)"=TRUE, "error in (no error)"=w2633, "Command"=w2630, "Queue with Cluster Reference"=w2629) -> ("error out"=w2636:errorcluster, "Queue Out (dup)"=w2635:T31)  [unwired: 2 in, 4 out]
        n746 = Bundle By Name(cluster=w2643, "Temp - Data (Volts)"=w2641) -> (w2642:T20)
      }
      frame "Analysis - FFT" {
        n747 = local read "AinFreq_Ideal"() -> (w2723:dbl)
        n748 = local read "Data Rate"() -> (w2722:dbl)
        n749 = local read "Samples/CH"() -> (w2724:u32)
        n750 = Unbundle By Name(w2718) -> ("Temp - Data (Volts)"=w2719:dbl[][])
        n751 = Unbundle By Name(w2703) -> ("Vref"=w2702:dbl)
        n752 = Bundle By Name(cluster="AC Analysis Parameters", "HiFreq (Hz)"="High Frequency", "LoFreq (Hz)"="Low Frequency") -> (w2699:T12)
        n753 = for "Perform FFT analysis on all channels" {
          tunnel: w2719 -> [w2762] mode=indexing
          tunnel: [w2769] -> w2716 mode=indexing
          tunnel: w2724 -> [w2768]
          tunnel: w2704 -> [w2767]
          tunnel: w2722 -> [w2766]
          tunnel: w2723 -> [w2765]
          tunnel: w2702 -> [w2743]
          tunnel: "Input Amplitude(Vpp)" -> [w2764]
          tunnel: w2699 -> [w2763]
          shift-right: [w2752] -> w2715
          shift-left: string[][] [] ("AC Analysis [] out") -> [w2753]
          tunnel: [w2748] -> w2714 mode=indexing
          tunnel: [w2747] -> w2706 mode=indexing
          i -> [w2750]
          n754 = Increment(x=w2750) -> (x+1=w2736:i32)
          n755 = control-ref of="This VI"() -> (w2741:refnum<vi>)
          n756 = Format Into String(format string="CH%dSET" ("initial string"), w2736) -> (resulting string=w2740:string)  [unwired: 2 in, 1 out]
          n757 = Multiply(x=ext 2.0, y=w2743) -> (x*y=w2758:ext)
          n758 = Divide(x=w2762, y=w2758) -> (x/y=w2757:ext[])
          n759 = Power Of 2(x=w2767) -> (2^x=w2756:dbl)
          n760 = invoke on="Invoke Node" class="VI" method="Ctrl Val.Get"(reference=w2741, "Control Name"=w2740) -> ("Get Control Value Variant"=w2738:variant)  [unwired: 2 in, 3 out]
          n761 = Multiply(x=w2757, y=w2756) -> (x*y=w2755:ext[])
          n762 = call "CST_Reg_CHxSET.vi"() -> ("CH1SET"=w2737:T3)  [unwired: 1 out]
          n763 = Variant To Data(Variant=w2738, type=w2737) -> (data=w2735:T3)  [unwired: 1 in, 1 out]
          n764 = Unbundle By Name(w2735) -> ("GAIN#"=w2760:enum16{"1", "2", "4", "6", "8", "12", "24"})
          n765 = Format Into String(w2760) -> (resulting string=w2761:string)  [unwired: 3 in, 1 out]
          n766 = Format Into String(format string="Channel %d", w2736) -> (resulting string=w2748:string)  [unwired: 2 in, 1 out]
          n767 = Decimal String To Number(string=w2761) -> (number=w2731:i32)  [unwired: 3 out]
          n768 = Multiply(x=w2755, y=w2731) -> (x*y=w2754:ext[])
          n769 = call "SNR_Analysis.vi"("Ain (Input)"=w2754, "Input Ain Freq. (Hz)"=w2765, "AC Analysis Parameters"=w2763, "Ideal Sampling Rate"=w2766, "Number of Bits"=w2767, "Number of Samples"=w2768) -> ("PSRR/CMRR/BW"=w2745:T42, "FFT Magnitude Plot (dB)"=w2769:cluster{i32, dbl, dbl[]}, "ACParameter"=w2746:T43)  [unwired: 1 in, 2 out]
          n770 = call "Format_CMRR_BW.vi"("Range Count"=2 ("First Range"), "First Range"=5, "PSRR/CMRR/BW"=w2745) -> ("CMRR/BW Table"=w2747:string[][])  [unwired: 8 out]
          n771 = Unbundle By Name(w2745) -> ("Fund(dB)"=w2744:dbl)
          n772 = call "Calc_CMRR.vi"("PGA"=w2731, "Enable"=TRUE, "Input Amplitude(Vpp)"=w2743, "Vref (User Entered)"=w2764, "Fund(dB)"=w2744) -> ("CMRR"=w2751:ext, "PGA Out"=w2742:i32)  [unwired: 2 in, 3 out]
          n773 = call "Format_ACAnalysis.vi"("CMRR"=w2751, "PGA"=w2742, "ACParameter"=w2746, "AC Analysis [] in"=w2753) -> ("AC Analysis [] out"=w2752:string[][])  [unwired: 7 out]
        }
        n774 = Bundle By Name(cluster=w2718, "FFT.CMRR/BW Table"=w2706, "FFT.FFT Data"=w2716, "FFT.Table Col Hdrs"=w2714, "FFT.Table Row Hdrs"=string[] ["SNR (dBFS)", "SNRD(dB)", "THD (dBc)", "SFDR (dBc)", "ENOB", "enob", "# of Harmonics (SNR)", "Worst Spur (dB)", "2nd HD (dBc)", "3rd HD (dBc)", "4th HD (dBc)", "5th HD (dBc)", "Fundamental (dB)", "", "PGA Setting", "CMRR"] ("Column Header Strings[]"), "FFT.Analysis Data"=w2715) -> (w2717:T20)
        n775 = call <userlib>:"Enqueue - ClusterCommand.vi"("At Front?"=TRUE, "error in (no error)"=w2709, "Command"="Plot - Update FFT", "Queue with Cluster Reference"=w2710) -> ("error out"=w2707:errorcluster, "Queue Out (dup)"=w2708:T31)  [unwired: 1 in, 5 out]
      }
      frame "Analysis - Histogram", "Analysis - Scope" {
        n776 = Unbundle By Name(w2773) -> ("Temp - Data (Volts)"=w2770:dbl[][])
        n777 = case "Select analysis to perform" shown="\"Analysis - Histogram\"" w2771 {
          tunnel: ["Plot - Update Scope" ("Command") "Plot - Update Histogram" ("Command")] -> w2776
          tunnel: w2773 -> [w2795 w2806]
          tunnel: [w2794 w2805] -> w2772
          tunnel: w2770 -> [_ w2804]
          tunnel: w2770 -> [w2789 w2797]
          frame "Analysis - Scope", Default {
            n778 = call "BasicAnalysis.vi"("Units"=enum16{"True RMS", "Noise RMS"}."True RMS", "Data (Volts)"=w2789) -> ("Analysis Data"=w2790:string[][], "Row Headers"=w2791:string[], "Column Headers"=w2792:string[])  [unwired: 7 out]
            n779 = Bundle By Name(cluster=w2795, "Scope.Table Col Hdrs"=w2792, "Scope.Table Row Hdrs"=w2791, "Scope.Analysis Data"=w2790) -> (w2794:T20)
          }
          frame "Analysis - Histogram" {
            n780 = for {
              tunnel: w2804 -> [w2810] mode=indexing
              tunnel: "Histogram Bins" -> [w2809]
              tunnel: [w2808] -> w2802 mode=indexing
              n781 = call <vilib>:"Histogram.vi"("intervals"=w2809, "X"=w2810) -> ("Histogram Graph"=w2808:T44)  [unwired: 9 out]
            }
            n782 = call "BasicAnalysis.vi"("Units"=enum16{"True RMS", "Noise RMS"}."Noise RMS", "Data (Volts)"=w2797) -> ("Analysis Data"=w2800:string[][], "Row Headers"=w2799:string[], "Column Headers"=w2798:string[])  [unwired: 7 out]
            n783 = Bundle By Name(cluster=w2806, "Histogram.Table Col Hdrs"=w2798, "Histogram.Table Row Hdrs"=w2799, "Histogram.Analysis Data"=w2800, "Histogram.Histogram Data"=w2802) -> (w2805:T20)
          }
        }
        n784 = call <userlib>:"Enqueue - ClusterCommand.vi"("At Front?"=TRUE, "error in (no error)"=w2785, "Command"=w2776, "Queue with Cluster Reference"=w2786) -> ("error out"=w2783:errorcluster, "Queue Out (dup)"=w2784:T31)  [unwired: 1 in, 5 out]
      }
      frame "Analysis Table" {
        n785 = Variant To Data(Variant=w2821, type="") -> (data=w2814:string)  [unwired: 1 in, 1 out]
        n786 = case "Select analysis data to show in table" shown="\"Histogram\"" w2814 {
          tunnel: w2822 -> [_ w2838 w2842 w2847]
          tunnel: [_ w2837 w2841 w2846] -> w2817
          tunnel: [_ w2836 w2840 w2845] -> w2818
          tunnel: [_ w2834 w2839 w2843] -> w2819
          frame Default {
          }
          frame "Histogram" {
            n787 = Unbundle By Name(w2838) -> ("Histogram.Analysis Data"=w2835:string[][], "Histogram.Table Row Hdrs"=w2836:string[], "Histogram.Table Col Hdrs"=w2837:string[])
            n788 = Transpose 2D Array(2D array=w2835) -> (transposed array=w2834:string[][])
          }
          frame "FFT" {
            n789 = Unbundle By Name(w2842) -> ("FFT.Analysis Data"=w2839:string[][], "FFT.Table Col Hdrs"=w2840:string[], "FFT.Table Row Hdrs"=w2841:string[])
          }
          frame "Scope" {
            n790 = Unbundle By Name(w2847) -> ("Scope.Analysis Data"=w2844:string[][], "Scope.Table Row Hdrs"=w2845:string[], "Scope.Table Col Hdrs"=w2846:string[])
            n791 = Transpose 2D Array(2D array=w2844) -> (transposed array=w2843:string[][])
          }
        }
        n792 = Format Into String(format string="%s Analysis", w2814) -> (resulting string=w2815:string)  [unwired: 2 in, 1 out]
        n793 = Build Path(base path=w2811, name or relative path="Modules\\StatTable_Popup.vi") -> (appended path=w2812:path)
        n794 = call "StatTable_Prep.vi"("Window Title"=w2815, "Path"=w2812, "Table Row Hdrs[]"=w2817, "Table Col Hdrs[]"=w2818, "Table Data"=w2819) -> ()  [unwired: 7 out]
      }
      frame ">-----Plot/Update Graphs ---------------------" {
        # "List separator case"
      }
      frame "Plot - Update Scope" {
        w2865 = T14 0 items=["Enable", "Disable", "Disable/Gray"] ("Disable Property")
        n795 = Unbundle By Name(w2872) -> ("Temp - Data (Volts)"=w2869:dbl[][])
        "Graph - Scope" <- w2869
        n796 = Send Notification(notification="Displaying Scope Data" ("Message"), notifier=w2862, error in (no error)=w2861) -> (error out=w2860:errorcluster)  [unwired: 1 out]
        n797 = Array Size(array=w2869) -> (size(s)=w2868:i32[])
        n798 = Equal To 0?(x="Plot Selector - Scope") -> (x = 0?=w2870:bool)
        n799 = Index Array(array=w2868, index=0) -> (element=w2866:i32)
        n800 = Decrement(x="Plot Selector - Scope") -> (x-1=w2864:u16)
        n801 = for "Show desired channels" {
          N: w2866 -> [_]
          tunnel: w2864 -> [w2888]
          tunnel: w2870 -> [w2886]
          i -> [w2885]
          n802 = Equal?(x=w2888, y=w2885) -> (x = y?=w2887:bool)
          n803 = Or(x=w2886, y=w2887) -> (x .or. y?=w2884:bool)
          n804 = property on="Graph - Scope" class="WFGraph (strict)"("Active Plot"=w2885) -> (error out=w2883:errorcluster)  [unwired: 2 in, 1 out]
          n805 = property on="Graph - Scope" class="WFGraph (strict)"(error in=w2883, "Plot.Visible?"=w2884) -> ()  [unwired: 1 in, 2 out]
        }
        n806 = property on="Save Analysis:Scope" class="Bool (strict)"("Disabled"=w2865) -> ()  [unwired: 2 in, 2 out]
      }
      frame "Plot - Update Histogram" {
        w2893 = T14 0 items=["Enable", "Disable", "Disable/Gray"] ("Disable Property")
        n807 = Unbundle By Name(w2899) -> ("Histogram.Histogram Data"=w2896:T11)
        "Graph - Histogram" <- w2896
        n808 = Send Notification(notification="Displaying Histogram Data" ("Message"), notifier=w2891, error in (no error)=w2890) -> (error out=w2889:errorcluster)  [unwired: 1 out]
        n809 = Equal To 0?(x="Plot Selector - Histogram") -> (x = 0?=w2898:bool)
        n810 = Array Size(array=w2896) -> (size(s)=w2894:i32)
        n811 = Decrement(x="Plot Selector - Histogram") -> (x-1=w2897:u16)
        n812 = for {
          N: w2894 -> [_]
          tunnel: w2897 -> [w2915]
          tunnel: w2898 -> [w2913]
          i -> [w2912]
          n813 = Equal?(x=w2915, y=w2912) -> (x = y?=w2914:bool)
          n814 = Or(x=w2913, y=w2914) -> (x .or. y?=w2911:bool)
          n815 = property on="Graph - Histogram" class="XYGraph (strict)"("Active Plot"=w2912) -> (error out=w2910:errorcluster)  [unwired: 2 in, 1 out]
          n816 = property on="Graph - Histogram" class="XYGraph (strict)"(error in=w2910, "Plot.Visible?"=w2911) -> ()  [unwired: 1 in, 2 out]
        }
        n817 = property on="Save Analysis:Histogram" class="Bool (strict)"("Disabled"=w2893) -> ()  [unwired: 2 in, 2 out]
        n818 = property on="Save Data:Histogram" class="Bool (strict)"("Disabled"=w2893) -> ()  [unwired: 2 in, 2 out]
      }
      frame "Plot - Update FFT" {
        w2921 = T14 0 items=["Enable", "Disable", "Disable/Gray"] ("Disable Property")
        n819 = Unbundle By Name(w2929) -> ("FFT.FFT Data"=w2926:cluster{i32, dbl, dbl[]}[], "FFT.CMRR/BW Table"=w2923:string[][][])
        "Graph - FFT" <- w2926
        n820 = Equal To 0?(x="Plot Selector - FFT") -> (x = 0?=w2925:bool)
        n821 = Send Notification(notification="Displaying FFT Data" ("Message"), notifier=w2916, error in (no error)=w2918) -> (error out=w2917:errorcluster)  [unwired: 1 out]
        n822 = Array Size(array=w2926) -> (size(s)=w2927:i32)
        n823 = Decrement(x="Plot Selector - FFT") -> (x-1=w2922:u16)
        n824 = for {
          N: w2927 -> [_]
          tunnel: w2922 -> [w2951]
          tunnel: w2925 -> [w2949]
          i -> [w2948]
          n825 = Equal?(x=w2951, y=w2948) -> (x = y?=w2950:bool)
          n826 = Or(x=w2949, y=w2950) -> (x .or. y?=w2947:bool)
          n827 = property on="Graph - FFT" class="WFGraph (strict)"("Active Plot"=w2948) -> (error out=w2946:errorcluster)  [unwired: 2 in, 1 out]
          n828 = property on="Graph - FFT" class="WFGraph (strict)"(error in=w2946, "Plot.Visible?"=w2947) -> ()  [unwired: 1 in, 2 out]
        }
        n829 = case shown="False" w2925 {
          tunnel: [w2941 string[][] [] ("CMRR/BW Table")] -> w2924
          tunnel: w2923 -> [w2943 _]
          tunnel: w2922 -> [w2942 _]
          tunnel: [w2940 w2944] -> w2920
          frame False {
            w2940 = T14 0 items=["Enable", "Disable", "Disable/Gray"] ("Disable Property")
            n830 = Index Array(array=w2943, index (dim 0)=w2942) -> (element=w2941:string[][])  [unwired: 2 in]
          }
          frame True {
            w2944 = T14 2 items=["Enable", "Disable", "Disable/Gray"] ("Disable Property")
          }
        }
        "Analysis - Dynamic Range" <- w2924
        n831 = property on="Analysis - Dynamic Range" class="Tbl (strict)"("Disabled"=w2920) -> ()  [unwired: 2 in, 2 out]
        n832 = property on="Save Data:FFT" class="Bool (strict)"("Disabled"=w2921) -> ()  [unwired: 2 in, 2 out]
        n833 = property on="Save Analysis:FFT" class="Bool (strict)"("Disabled"=w2921) -> ()  [unwired: 2 in, 2 out]
      }
      frame ">---- User Input ------------" {
        # "List separator case"
      }
      frame "User Input - <Blank>" {
        # "Blank user input case\nUse this case and create duplicates which can be coded to handle\nthe user actions from the user event structure."
      }
      frame "User Input - Filter Data" {
        w2988 = T14 2 items=["Enable", "Disable", "Disable/Gray"] ("Disable Property")
        w2989 = T14 0 items=["Enable", "Disable", "Disable/Gray"] ("Disable Property")
        n834 = Variant To Data(error in=w2985, Variant=w2986, type=TRUE) -> (error out=w2984:errorcluster, data=w2983:bool)
        n835 = Select(t=w2989, s=w2983, f=w2988) -> (s? t:f=w2987:T14)
        n836 = case shown="\"HPF Enable\"" w2981 {
          tunnel: w2987 -> [w3003 w3004 w3011]
          tunnel: [w3000 w3005 w3009] -> w2978
          tunnel: w2984 -> [w3002 w3007 w3008]
          frame "LPF Enable" {
            n837 = property on="LPF Cutoff" class="DigNum (strict)"(error in=w3002, "DisabledEnum"=w3003) -> (error out=w3001:errorcluster)  [unwired: 1 in, 1 out]
            n838 = property on="LPF Order" class="DigNum (strict)"(error in=w3001, "DisabledEnum"=w3003) -> (error out=w3000:errorcluster)  [unwired: 1 in, 1 out]
          }
          frame "HPF Enable" {
            n839 = property on="HPF Cutoff" class="DigNum (strict)"(error in=w3007, "DisabledEnum"=w3004) -> (error out=w3006:errorcluster)  [unwired: 1 in, 1 out]
            n840 = property on="HPF Order" class="DigNum (strict)"(error in=w3006, "DisabledEnum"=w3004) -> (error out=w3005:errorcluster)  [unwired: 1 in, 1 out]
          }
          frame "Notch Enable", Default {
            n841 = property on="Notch Order" class="DigNum (strict)"(error in=w3008, "DisabledEnum"=w3011) -> (error out=w3010:errorcluster)  [unwired: 1 in, 1 out]
            n842 = property on="Notch Freq" class="Ring (strict)"(error in=w3010, "DisabledEnum"=w3011) -> (error out=w3009:errorcluster)  [unwired: 1 in, 1 out]
          }
        }
        n843 = call-poly <userlib>:"Enqueue - ClusterQueue.vi"("error in (no error)"=w2978, "Command"="Analysis - Convert Data", "Queue with Cluster Reference"=w2979) -> ("error out"=w2977:errorcluster, "Queue Out (dup)"=w2976:T31)  [unwired: 2 in, 5 out]
      }
      frame "User Input - Device Status" {
        # "SPI Commands"
        n844 = Variant To Data(Variant=w3024, type=FALSE) -> (data=w3020:bool)  [unwired: 1 in, 1 out]
        n845 = To Upper Case(1:w3012) -> (0:w3021:string)
        n846 = case shown="\"RESET\"" w3021 {
          tunnel: w3020 -> [_ w3065]
          tunnel: w3019 -> [w3052 w3076]
          tunnel: w3016 -> [w3051 w3075]
          tunnel: w3018 -> [w3050 w3070]
          tunnel: [w3049 w3070] -> w3017
          tunnel: [w3047 w3069] -> w3015
          tunnel: w3014 -> [w3046 _]
          tunnel: w3013 -> [w3045 w3074]
          frame "RESET" {
            n847 = Unbundle By Name(w3052) -> ("Client ptr"=w3037:u32)
            n848 = call "FG_ADS1299EVMEstyxFiles.vi"("Storage Info"=TYP_ADS1299Estyx_File_Enum."conf|reset" ("Styx File Tags - Enum")) -> ("File Path"=w3036:string)  [unwired: 2 in, 8 out]
            n849 = To Byte Integer(number="Reset Mode") -> (8bit integer=w3034:i8)
            n850 = Increment(x=w3034) -> (x+1=w3033:i8)
            n851 = call-poly "lvstyx_file_write.vi"("error in (no error)"=w3051, "int64"=w3033, "path"=w3036, "client ptr"=w3037) -> ("error out"=w3048:errorcluster)  [unwired: 6 in, 1 out]
            n852 = invoke class="VI" method="Default Vals.Reinit All"(error in=w3048) -> (error out=w3039:errorcluster)  [unwired: 2 in, 2 out]
            n853 = Send Notification(notification=T15 {"State"=enum."Pause", "Data"=0}, notifier=w3046) -> ()  [unwired: 1 in, 2 out]
            n854 = Send Notification(notification="Resetting the device....", notifier=w3045) -> ()  [unwired: 1 in, 2 out]
            n855 = while "Wait for \"reset\" to read back as \"0\" (or timeout at 50sec)" {
              tunnel: w3039 -> [w3064]
              tunnel: [w3063] -> w3038
              tunnel: w3037 -> [w3062]
              tunnel: w3036 -> [w3055]
              i -> [w3059]
              stop <- w3061 continue-if-true
              n856 = call-poly "lvstyx_file_read.vi"("error in (no error)"=w3064, "path"=w3055, "client ptr"=w3062) -> ("error out"=w3063:errorcluster, "int32"=w3054:i32)  [unwired: 6 in, 1 out]
              n857 = Not Equal To 0?(x=w3054) -> (x != 0?=w3056:bool)
              n858 = Greater Or Equal?(x=5000, y=w3059) -> (x >= y?=w3060:bool)
              n859 = And(x=w3060, y=w3056) -> (x .and. y?=w3061:bool)
              n860 = Wait (ms)(milliseconds to wait=u32 10) -> ()  [unwired: 1 out]
            }
            n861 = Flush Queue(queue=w3050, error in (no error)=w3038) -> (queue out=w3042:T31, error out=w3041:errorcluster)  [unwired: 1 out]
            n862 = call-poly <userlib>:"Enqueue - ClusterQueue.vi"("error in"=w3041, "Array of Commands"=string[] ["State - Initialize", "State - Initialize2"], "Queue with Cluster Reference"=w3042) -> ("error out"=w3047:errorcluster, "Queue (dup)"=w3049:T31)  [unwired: 2 in, 5 out]
          }
          frame "STANDBY", Default {
            w3066 = T14 2 items=["Enable", "Disable", "Disable/Gray"] ("Disable Property")
            w3068 = T14 0 items=["Enable", "Disable", "Disable/Gray"] ("Disable Property")
            n863 = Unbundle By Name(w3076) -> ("Client ptr"=w3078:u32)
            n864 = call "FG_ADS1299EVMEstyxFiles.vi"("Storage Info"=TYP_ADS1299Estyx_File_Enum."conf|sleep" ("Styx File Tags - Enum")) -> ("File Path"=w3079:string)  [unwired: 2 in, 8 out]
            n865 = Select(t="Device is sleeping..." ("notification"), s=w3065, f="Device is awake..." ("notification")) -> (s? t:f=w3072:string)
            n866 = Send Notification(notification=w3072, notifier=w3074) -> ()  [unwired: 1 in, 2 out]
            n867 = call-poly "lvstyx_file_write.vi"("error in (no error)"=w3075, "boolean"=w3065, "path"=w3079, "client ptr"=w3078) -> ("error out"=w3069:errorcluster)  [unwired: 6 in, 1 out]
            n868 = Select(t=w3066, s=w3065, f=w3068) -> (s? t:f=w3067:T14)
            n869 = property on="Acq - Single" class="Bool"("Disabled"=w3067) -> ()  [unwired: 2 in, 2 out]
            n870 = property on="Acq - Continuous" class="Bool (strict)"("Disabled"=w3067) -> ()  [unwired: 2 in, 2 out]
          }
        }
      }
      frame "User Input - Channel Set" {
        w3092 = refnum<vi> refnum  # Cluster
        n871 = Variant To Data(Variant=w3105, type=w3092) -> (data=w3090:refnum<vi>)  [unwired: 1 in, 1 out]
        n872 = property on="Property Node" class="Clust"(reference=w3090) -> ("Label.Text"=w3087:string, "Controls[]"=w3082:refnum<vi>[], "Value"=w3095:variant)  [unwired: 1 in, 2 out]
        n873 = Unbundle By Name(w3088) -> ("Register Names"=w3089:string[], "RegMap Data"=w3085:T22[])
        n874 = Scan From String(format string="CH%dSET", input string=w3087) -> (output 1=w3080:i32)  [unwired: 2 in, 4 out]
        n875 = Search 1D Array(1D array=w3089, element=w3087) -> (index of element=w3086:i32)  [unwired: 1 out]
        n876 = call "CST_Reg_CHxSET.vi"() -> ("CH1SET"=w3084:T3)  [unwired: 1 out]
        n877 = Variant To Data(Variant=w3095, type=w3084) -> (data=w3091:T3)  [unwired: 1 in, 1 out]
        n878 = Index Array(array=w3085, index=w3086) -> (element=w3083:T22)
        n879 = case "Select shift data to modify" shown="3" w3080 {
          tunnel: w3101 -> [w3116 w3119 w3122 w3125 w3128 w3131 w3134 w3137]
          tunnel: [w3115 w3118 w3121 w3124 w3127 w3130 w3133 w3136] -> w3100
          tunnel: w3091 -> [w3114 w3117 w3120 w3123 w3126 w3129 w3132 w3135]
          frame 1, Default {
            n880 = Bundle By Name(cluster=w3116, "CH1SET"=w3114) -> (w3115:T34)
          }
          frame 2 {
            n881 = Bundle By Name(cluster=w3119, "CH2SET"=w3117) -> (w3118:T34)
          }
          frame 3 {
            n882 = Bundle By Name(cluster=w3122, "CH3SET"=w3120) -> (w3121:T34)
          }
          frame 4 {
            n883 = Bundle By Name(cluster=w3125, "CH4SET"=w3123) -> (w3124:T34)
          }
          frame 5 {
            n884 = Bundle By Name(cluster=w3128, "CH5SET"=w3126) -> (w3127:T34)
          }
          frame 6 {
            n885 = Bundle By Name(cluster=w3131, "CH6SET"=w3129) -> (w3130:T34)
          }
          frame 7 {
            n886 = Bundle By Name(cluster=w3134, "CH7SET"=w3132) -> (w3133:T34)
          }
          frame 8 {
            n887 = Bundle By Name(cluster=w3137, "CH8SET"=w3135) -> (w3136:T34)
          }
        }
        n888 = call "Register_ValueCalc.vi"("Index"=w3080, "ADSxxxx Register Data"=w3083, "Register Controls[]"=w3082) -> ("Register Value Calculated"=w3081:u32)  [unwired: 8 in]
        n889 = Decrement(x=w3080) -> (x-1=w3097:i32)
        n890 = Add(x=TYP_ADS1299Estyx_File_Enum."conf|ch1set" ("Styx File Tags - Enum"), y=w3097) -> (x+y=w3096:i32)
        n891 = Unbundle By Name(w3107) -> ("Client ptr"=w3103:u32)
        n892 = call "FG_ADS1299EVMEstyxFiles.vi"("Storage Info"=w3096) -> ("File Path"=w3102:string)  [unwired: 2 in, 8 out]
        n893 = call-poly "lvstyx_file_write.vi"("error in (no error)"=w3094, "int64"=w3081, "path"=w3102, "client ptr"=w3103) -> ("error out"=w3093:errorcluster)  [unwired: 6 in, 1 out]
      }
      frame "User Input - Config Set" {
        n894 = Variant To Data(Variant=w3160, type="" ("Empty String Constant")) -> (data=w3157:string)  [unwired: 1 in, 1 out]
        n895 = To Upper Case(1:w3157) -> (0:w3144:string)
        n896 = Unbundle By Name(w3146) -> ("Reg - AllCtrls.References"=w3143:refnum<vi>[], "Reg - AllCtrls.Names/Labels"=w3145:string[])
        n897 = Unbundle By Name(w3149) -> ("Register Names"=w3148:string[], "RegMap Data"=w3147:T22[])
        n898 = Search 1D Array(1D array=w3145, element=w3144) -> (index of element=w3142:i32)  [unwired: 1 out]
        n899 = Search 1D Array(1D array=w3148, element=w3144) -> (index of element=w3158:i32)  [unwired: 1 out]
        n900 = Index Array(array=w3143, index=w3142) -> (element=w3141:refnum<vi>)
        n901 = case "Update shifter values and get register control references" shown="\"CONFIG1\", Default" w3144 {
          tunnel: [TYP_ADS1299Estyx_File_Enum."conf|config1" ("Styx File Tags - Enum") TYP_ADS1299Estyx_File_Enum."conf|config2" ("Styx File Tags - Enum") TYP_ADS1299Estyx_File_Enum."conf|config3" ("Styx File Tags - Enum") TYP_ADS1299Estyx_File_Enum."conf|config4" ("Styx File Tags - Enum")] -> w3154
          tunnel: [w3174 w3182 w3190 w3198] -> w3153
          tunnel: w3152 -> [w3173 w3180 w3189 w3196]
          tunnel: w3141 -> [w3172 w3176 w3186 w3194]
          tunnel: [w3169 w3178 w3187 w3193] -> w3140
          tunnel: w3151 -> [_ _ _ _]
          frame "CONFIG1", Default {
            n902 = control-ref of="CONFIG1"() -> (w3171:refnum<vi>)
            n903 = To More Specific Class(target class=w3171, reference=w3172) -> (specific class reference=w3170:refnum<vi>)  [unwired: 1 in, 1 out]
            n904 = property on="Property Node" class="Clust (strict)"(reference=w3171) -> ("Value"=w3168:T45)  [unwired: 1 in, 2 out]
            n905 = property on="Property Node" class="Clust (strict)"(reference=w3170) -> ("Controls[]"=w3169:refnum<vi>[])  [unwired: 1 in, 2 out]
            n906 = Bundle By Name(cluster=w3173, "Config1"=w3168) -> (w3174:T34)
          }
          frame "CONFIG2" {
            n907 = control-ref of="CONFIG2"() -> (w3177:refnum<vi>)
            n908 = To More Specific Class(target class=w3177, reference=w3176) -> (specific class reference=w3179:refnum<vi>)  [unwired: 1 in, 1 out]
            n909 = property on="Property Node" class="Clust (strict)"(reference=w3177) -> ("Value"=w3181:T46)  [unwired: 1 in, 2 out]
            n910 = property on="Property Node" class="Clust (strict)"(reference=w3179) -> ("Controls[]"=w3178:refnum<vi>[])  [unwired: 1 in, 2 out]
            n911 = Bundle By Name(cluster=w3180, "Config2"=w3181) -> (w3182:T34)
          }
          frame "CONFIG3" {
            n912 = control-ref of="CONFIG3"() -> (w3185:refnum<vi>)
            n913 = To More Specific Class(target class=w3185, reference=w3186) -> (specific class reference=w3188:refnum<vi>)  [unwired: 1 in, 1 out]
            n914 = property on="Property Node" class="Clust (strict)"(reference=w3185) -> ("Value"=w3184:T47)  [unwired: 1 in, 2 out]
            n915 = property on="Property Node" class="Clust (strict)"(reference=w3188) -> ("Controls[]"=w3187:refnum<vi>[])  [unwired: 1 in, 2 out]
            n916 = Bundle By Name(cluster=w3189, "Config3"=w3184) -> (w3190:T34)
          }
          frame "CONFIG4" {
            n917 = control-ref of="CONFIG4"() -> (w3192:refnum<vi>)
            n918 = To More Specific Class(target class=w3192, reference=w3194) -> (specific class reference=w3195:refnum<vi>)  [unwired: 1 in, 1 out]
            n919 = property on="Property Node" class="Clust (strict)"(reference=w3192) -> ("Value"=w3197:T48)  [unwired: 1 in, 2 out]
            n920 = property on="Property Node" class="Clust (strict)"(reference=w3195) -> ("Controls[]"=w3193:refnum<vi>[])  [unwired: 1 in, 2 out]
            n921 = Bundle By Name(cluster=w3196, "Config4"=w3197) -> (w3198:T34)
          }
        }
        n922 = Index Array(array=w3147, index=w3158) -> (element=w3139:T22)
        n923 = call "Register_ValueCalc.vi"("ADSxxxx Register Data"=w3139, "Register Controls[]"=w3140) -> ("Register Value Calculated"=w3138:u32)  [unwired: 9 in]
        n924 = Unbundle By Name(w3162) -> ("Client ptr"=w3156:u32)
        n925 = call "FG_ADS1299EVMEstyxFiles.vi"("Storage Info"=w3154) -> ("File Path"=w3155:string)  [unwired: 2 in, 8 out]
        n926 = call-poly "lvstyx_file_write.vi"("int64"=w3138, "path"=w3155, "client ptr"=w3156) -> ()  [unwired: 7 in, 2 out]
      }
      frame "User Input - Update Data Rate" {
        w3211 = 4  # Base frequency divisor (2^n)
        n927 = call "CST_Reg_CONFIG1.vi"() -> ("CONFIG1"=w3212:T6)  [unwired: 1 out]
        n928 = Variant To Data(Variant=w3214, type=w3212) -> (data=w3213:T6)  [unwired: 1 in, 1 out]
        n929 = Unbundle By Name(w3213) -> ("DR"=w3205:T49)
        n930 = Add(x=w3205, y=w3211) -> (x+y=w3210:i32)
        n931 = Power Of 2(x=w3210) -> (2^x=w3208:dbl)
        n932 = Unbundle By Name(w3203) -> ("f(CLK)"=w3206:dbl)
        n933 = Multiply(x=8, y=w3208) -> (x*y=w3207:dbl)
        n934 = Divide(x=w3206, y=w3207) -> (x/y=→"Data Rate":dbl)
        n935 = case "Handle data bit change for high-speed\noperation" shown="\"f(MOD) /64\", \"f(MOD) /128\"" w3205 {
          tunnel: w3204 -> [_ w3231]
          tunnel: [24 ("#bits") w3231] -> w3201
          frame "f(MOD) /64", "f(MOD) /128" {
          }
          frame Default {
          }
        }
        n936 = Bundle By Name(cluster=w3203, "Word Bits"=w3201) -> (w3202:T21)
        n937 = call <userlib>:"Enqueue - ClusterBoth.vi"("At Front? (F)"=TRUE, "error in (no error)"=w3220, "Command"="CalculateFin", "Queue with Cluster Reference"=w3221) -> ("error out"=w3218:errorcluster, "Queue Out (dup)"=w3219:T31)  [unwired: 2 in, 4 out]
      }
      frame "User Input - Update VREF" {
        # "2.4 or 4.0 minimum\nuser selected desired"
        # "?"
        n938 = Variant To Data(Variant=w3239, type=enum16{"VREFP = 2.4V", "VREFP = 4V"}."VREFP = 2.4V" ("VREFP")) -> (data=w3232:enum16{"VREFP = 2.4V", "VREFP = 4V"})  [unwired: 1 in, 1 out]
        n939 = Format Into String(w3232) -> (resulting string=w3238:string)  [unwired: 3 in, 1 out]
        n940 = Scan From String(format string="%[^=]=\\s%f", input string=w3238) -> (output 2=w3234:dbl)  [unwired: 2 in, 6 out]
        n941 = Bundle By Name(cluster=w3236, "Vref"=w3234) -> (w3235:T21)
        n942 = call-poly <userlib>:"Enqueue - ClusterQueue.vi"("error in (no error)"=w3249, "Command"="Idle", "Queue with Cluster Reference"=w3250) -> ("error out"=w3247:errorcluster, "Queue Out (dup)"=w3248:T31)  [unwired: 3 in, 4 out]
      }
      frame "User Input - BIAS Enable" {
        n943 = Variant To Data(Variant=w3262, type=enum16{"Disabled", "Enabled"}."Enabled" ("PD_BIAS")) -> (data=w3255:enum16{"Disabled", "Enabled"})  [unwired: 1 in, 1 out]
        n944 = case shown="\"Enabled\"" w3255 {
          tunnel: w3260 -> [w3272 w3298]
          tunnel: w3259 -> [w3271 w3297]
          tunnel: [w3272 w3279] -> w3258
          tunnel: [w3271 w3278] -> w3257
          frame "Disabled" {
          }
          frame "Enabled" {
            n945 = local read "CONFIG3"() -> (w3293:T4)
            n946 = Bundle By Name(cluster=w3293, "BIAS_MEAS"=enum16{"Open", "BIASIN Routed"}."BIASIN Routed" ("RLD_MEAS"), "BIASREF_INT"=T29."BIASREF = (AVDD-AVSS)/2" ("RLDREF_INT")) -> (w3296:T4)
            n947 = call-poly <userlib>:"Enqueue - ClusterQueue.vi"("error in (no error)"=w3297, "Data"="CONFIG3", "Command"="User Input - Config Set", "Queue with Cluster Reference"=w3298) -> ("error out"=w3284:errorcluster, "Queue Out (dup)"=w3285:T31)  [unwired: 2 in, 4 out]
            n948 = local write "CONFIG3"(w3296) -> ()
            n949 = local read "BIASSENSP"() -> (w3292:bool[])
            n950 = Replace Array Subset(array=w3292, new element=bool[] [TRUE, TRUE], index=5) -> (w3283:bool[])
            n951 = Reverse 1D Array(array=w3283) -> (reversed array=w3277:bool[])
            n952 = local write "BIASSENSP"(w3283) -> ()
            n953 = call-poly <userlib>:"Enqueue - ClusterQueue.vi"("error in (no error)"=w3284, "Data"=w3277, "Command"="User Input - BIAS_SENSE:BIAS_SENSP", "Queue with Cluster Reference"=w3285) -> ("error out"=w3280:errorcluster, "Queue Out (dup)"=w3281:T31)  [unwired: 2 in, 4 out]
            n954 = local read "BIASSENSN"() -> (w3288:bool[])
            n955 = Replace Array Subset(array=w3288, new element=TRUE, index=6) -> (w3276:bool[])
            n956 = local write "BIASSENSN"(w3276) -> ()
            n957 = Reverse 1D Array(array=w3276) -> (reversed array=w3275:bool[])
            n958 = call-poly <userlib>:"Enqueue - ClusterQueue.vi"("error in (no error)"=w3280, "Data"=w3275, "Command"="User Input - BIAS_SENSE:BIAS_SENSN", "Queue with Cluster Reference"=w3281) -> ("error out"=w3278:errorcluster, "Queue Out (dup)"=w3279:T31)  [unwired: 2 in, 4 out]
          }
        }
      }
      frame "User Input - BIAS_SENSE" {
        n959 = Variant To Data(Variant=w3307, type=bool[] [FALSE, FALSE, FALSE, FALSE, FALSE, FALSE, FALSE, FALSE] ("RLD_SENSP")) -> (data=w3301:bool[])  [unwired: 1 in, 1 out]
        n960 = Boolean Array To Number(Boolean array=w3301) -> (number=w3299:u32)
        n961 = case shown="\"BIAS_SENSN\"" w3300 {
          tunnel: w3310 -> [w3323 w3327]
          tunnel: [w3322 w3326] -> w3309
          tunnel: [TYP_ADS1299Estyx_File_Enum."conf|biassensp" ("Styx File Tags - Enum") TYP_ADS1299Estyx_File_Enum."conf|biassensn" ("Styx File Tags - Enum")] -> w3305
          tunnel: w3301 -> [w3320 w3324]
          frame "BIAS_SENSP", Default {
            n962 = Bundle By Name(cluster=w3323, "BIASSENSP"=w3320) -> (w3322:T34)
          }
          frame "BIAS_SENSN" {
            n963 = Bundle By Name(cluster=w3327, "BIASSENSN"=w3324) -> (w3326:T34)
          }
        }
        n964 = call "FG_ADS1299EVMEstyxFiles.vi"("Storage Info"=w3305) -> ("File Path"=w3302:string)  [unwired: 2 in, 8 out]
        n965 = Unbundle By Name(w3311) -> ("Client ptr"=w3303:u32)
        n966 = call-poly "lvstyx_file_write.vi"("int64"=w3299, "path"=w3302, "client ptr"=w3303) -> ()  [unwired: 7 in, 2 out]
      }
      frame "User Input - LOFF_ARRAY" {
        n967 = Variant To Data(Variant=w3336, type=bool[] [FALSE, FALSE, FALSE, FALSE, FALSE, FALSE, FALSE, FALSE] ("RLD_SENSP")) -> (data=w3330:bool[])  [unwired: 1 in, 1 out]
        n968 = Boolean Array To Number(Boolean array=w3330) -> (number=w3328:u32)
        n969 = case shown="\"LOFF_SENSP\", Default" w3329 {
          tunnel: w3339 -> [w3352 w3356 w3360]
          tunnel: [w3351 w3355 w3359] -> w3338
          tunnel: [TYP_ADS1299Estyx_File_Enum."conf|loffsensp" ("Styx File Tags - Enum") TYP_ADS1299Estyx_File_Enum."conf|loffsensn" ("Styx File Tags - Enum") TYP_ADS1299Estyx_File_Enum."conf|loffflip" ("Styx File Tags - Enum")] -> w3334
          tunnel: w3330 -> [w3349 w3353 w3357]
          frame "LOFF_SENSP", Default {
            n970 = Bundle By Name(cluster=w3352, "LOFF_SENSP"=w3349) -> (w3351:T34)
          }
          frame "LOFF_SENSN" {
            n971 = Bundle By Name(cluster=w3356, "LOFF_SENSN"=w3353) -> (w3355:T34)
          }
          frame "LOFF_FLIP" {
            n972 = Bundle By Name(cluster=w3360, "LOFF_FLIP"=w3357) -> (w3359:T34)
          }
        }
        n973 = call "FG_ADS1299EVMEstyxFiles.vi"("Storage Info"=w3334) -> ("File Path"=w3331:string)  [unwired: 2 in, 8 out]
        n974 = Unbundle By Name(w3340) -> ("Client ptr"=w3332:u32)
        n975 = call-poly "lvstyx_file_write.vi"("int64"=w3328, "path"=w3331, "client ptr"=w3332) -> ()  [unwired: 7 in, 2 out]
      }
      frame "User Input - Globally Set Channels" {
        n976 = local read "Globally Set Channels"() -> (w3370:T3)
        n977 = Variant To Data(Variant=w3373, type=w3370) -> (data=w3364:T3)  [unwired: 1 in, 1 out]
        n978 = Bundle By Name(cluster=w3372, "CH1SET"=w3364, "CH2SET"=w3364, "CH3SET"=w3364, "CH4SET"=w3364, "CH5SET"=w3364, "CH6SET"=w3364, "CH7SET"=w3364, "CH8SET"=w3364) -> (w3371:T34)
        n979 = Unbundle By Name(w3363) -> ("Reg - AllCtrls.References"=w3362:refnum<vi>[], "Reg - AllCtrls.Names/Labels"=w3361:string[])
        n980 = for "Loop through each channel set control and set the values" {
          N: 8 -> [_]
          shift-right: [w3398] -> w3369
          shift-left: w3367 -> [w3396]
          shift-right: [w3397] -> w3368
          shift-left: w3366 -> [w3395]
          tunnel: w3364 -> [w3384]
          tunnel: w3362 -> [w3387]
          tunnel: w3361 -> [w3390]
          i -> [w3393]
          n981 = Increment(x=w3393) -> (x+1=w3394:i32)
          n982 = Format Into String(format string="%dSET", initial string="CH", w3394) -> (resulting string=w3389:string)  [unwired: 1 in, 1 out]
          n983 = Search 1D Array(1D array=w3390, element=w3389) -> (index of element=w3388:i32)  [unwired: 1 out]
          n984 = Index Array(array=w3387, index=w3388) -> (element=w3386:refnum<vi>)
          n985 = control-ref of="CH1SET"() -> (w3385:refnum<vi>)
          n986 = To More Specific Class(target class=w3385, reference=w3386) -> (specific class reference=w3382:refnum<vi>)  [unwired: 1 in, 1 out]
          n987 = property on="Property Node" class="Clust (strict)"(reference=w3382, "Value"=w3384) -> ()  [unwired: 1 in, 2 out]
          n988 = call-poly <userlib>:"Enqueue - ClusterQueue.vi"("error in (no error)"=w3395, "Data"=w3382, "Command"="User Input - Channel Set" ("string"), "Queue with Cluster Reference"=w3396) -> ("error out"=w3397:errorcluster, "Queue Out (dup)"=w3398:T31)  [unwired: 2 in, 4 out]
        }
      }
      frame "User Input - GPIO Data Change" {
        n989 = Variant To Data(error in=w3407, Variant=w3417, type=u32 0) -> (data=w3399:u32)  [unwired: 1 out]
        n990 = Number To Boolean Array(number=w3399) -> (Boolean array=w3403:bool[])
        n991 = Array Subset(array=w3403, index=4 ("length"), length=4) -> (w3400:bool[])
        n992 = Bundle By Name(cluster=w3413, "GPIO.Data"=w3400) -> (w3412:T34)
        n993 = Unbundle By Name(w3414) -> ("Client ptr"=w3409:u32)
        n994 = call "FG_ADS1299EVMEstyxFiles.vi"("Storage Info"=TYP_ADS1299Estyx_File_Enum."conf|gpio" ("Styx File Tags - Enum")) -> ("File Path"=w3408:string)  [unwired: 2 in, 8 out]
        n995 = call-poly "lvstyx_file_write.vi"("error in (no error)"=w3407, "int64"=w3399, "path"=w3408, "client ptr"=w3409) -> ("error out"=w3406:errorcluster)  [unwired: 6 in, 1 out]
      }
      frame "User Input - GPIO Direction Change" {
        w3437 = refnum<vi> refnum  # Boolean
        w3430 = T14 2 items=["Enable", "Disable", "Disable/Gray"] ("Disable Property")
        w3431 = T14 0 items=["Enable", "Disable", "Disable/Gray"] ("Disable Property")
        n996 = Variant To Data(error in=w3446, Variant=w3456, type=u32 0) -> (data=w3423:u32)  [unwired: 1 out]
        n997 = control-ref of="GPIO"() -> (w3429:refnum<vi>)
        n998 = property class="Clust (strict)"(reference=w3429) -> ("Controls[]"=w3428:refnum<vi>[])  [unwired: 1 in, 2 out]
        n999 = Number To Boolean Array(number=w3423) -> (Boolean array=w3442:bool[])
        n1000 = Array Subset(array=w3442, index=0, length=4) -> (w3434:bool[])
        n1001 = Scan From String(format string="GPIOC%d", input string=w3424) -> (output 1=w3435:i32)  [unwired: 2 in, 4 out]
        n1002 = Decrement(x=w3435) -> (x-1=w3426:i32)
        n1003 = Add(x=w3426, y=4) -> (x+y=w3427:i32)
        n1004 = Bundle By Name(cluster=w3452, "GPIO.Direction"=w3434) -> (w3451:T34)
        n1005 = Index Array(array=w3428, index=w3427) -> (element=w3439:refnum<vi>)
        n1006 = Index Array(array=w3434, index=w3426) -> (element=w3432:bool)
        n1007 = To More Specific Class(target class=w3437, reference=w3439) -> (specific class reference=w3438:refnum<vi>)  [unwired: 1 in, 1 out]
        n1008 = Select(t=w3430, s=w3432, f=w3431) -> (s? t:f=w3433:T14)
        n1009 = property class="Bool"(reference=w3438, "Disabled"=w3433) -> ()  [unwired: 1 in, 2 out]
        n1010 = Unbundle By Name(w3453) -> ("Client ptr"=w3448:u32)
        n1011 = call "FG_ADS1299EVMEstyxFiles.vi"("Storage Info"=TYP_ADS1299Estyx_File_Enum."conf|gpio" ("Styx File Tags - Enum")) -> ("File Path"=w3447:string)  [unwired: 2 in, 8 out]
        n1012 = call-poly "lvstyx_file_write.vi"("error in (no error)"=w3446, "int64"=w3423, "path"=w3447, "client ptr"=w3448) -> ("error out"=w3445:errorcluster)  [unwired: 6 in, 1 out]
      }
      frame "User Input - LOFF", "User Input - MISC1" {
        n1013 = Variant To Data(Variant=w3484, type="" ("Empty String Constant")) -> (data=w3481:string)  [unwired: 1 in, 1 out]
        n1014 = To Upper Case(1:w3481) -> (0:w3469:string)
        n1015 = Unbundle By Name(w3471) -> ("Reg - AllCtrls.References"=w3468:refnum<vi>[], "Reg - AllCtrls.Names/Labels"=w3470:string[])
        n1016 = Unbundle By Name(w3474) -> ("Register Names"=w3473:string[], "RegMap Data"=w3472:T22[])
        n1017 = Search 1D Array(1D array=w3470, element=w3469) -> (index of element=w3467:i32)  [unwired: 1 out]
        n1018 = Search 1D Array(1D array=w3473, element=w3469) -> (index of element=w3482:i32)  [unwired: 1 out]
        n1019 = Index Array(array=w3468, index=w3467) -> (element=w3466:refnum<vi>)
        n1020 = case "Update shifter values and get register control references" shown="\"MISC1\"" w3469 {
          tunnel: [TYP_ADS1299Estyx_File_Enum."conf|loff" ("Styx File Tags - Enum") TYP_ADS1299Estyx_File_Enum."conf|misc1" ("Styx File Tags - Enum")] -> w3478
          tunnel: [w3498 w3506] -> w3477
          tunnel: w3476 -> [w3497 w3504]
          tunnel: w3466 -> [w3496 w3500]
          tunnel: [w3493 w3502] -> w3463
          tunnel: w3465 -> [_ _]
          frame "LOFF", Default {
            n1021 = control-ref of="LOFF"() -> (w3495:refnum<vi>)
            n1022 = To More Specific Class(target class=w3495, reference=w3496) -> (specific class reference=w3494:refnum<vi>)  [unwired: 1 in, 1 out]
            n1023 = property on="Property Node" class="Clust (strict)"(reference=w3495) -> ("Value"=w3492:T50)  [unwired: 1 in, 2 out]
            n1024 = property on="Property Node" class="Clust (strict)"(reference=w3494) -> ("Controls[]"=w3493:refnum<vi>[])  [unwired: 1 in, 2 out]
            n1025 = Bundle By Name(cluster=w3497, "LOFF"=w3492) -> (w3498:T34)
          }
          frame "MISC1" {
            n1026 = control-ref of="MISC1"() -> (w3501:refnum<vi>)
            n1027 = To More Specific Class(target class=w3501, reference=w3500) -> (specific class reference=w3503:refnum<vi>)  [unwired: 1 in, 1 out]
            n1028 = property on="Property Node" class="Clust (strict)"(reference=w3501) -> ("Value"=w3505:T51)  [unwired: 1 in, 2 out]
            n1029 = property on="Property Node" class="Clust (strict)"(reference=w3503) -> ("Controls[]"=w3502:refnum<vi>[])  [unwired: 1 in, 2 out]
            n1030 = Bundle By Name(cluster=w3504, "MISC1"=w3505) -> (w3506:T34)
          }
        }
        n1031 = Index Array(array=w3472, index=w3482) -> (element=w3464:T22)
        n1032 = call "Register_ValueCalc.vi"("ADSxxxx Register Data"=w3464, "Register Controls[]"=w3463) -> ("Register Value Calculated"=w3462:u32)  [unwired: 9 in]
        n1033 = Unbundle By Name(w3486) -> ("Client ptr"=w3480:u32)
        n1034 = call "FG_ADS1299EVMEstyxFiles.vi"("Storage Info"=w3478) -> ("File Path"=w3479:string)  [unwired: 2 in, 8 out]
        n1035 = call-poly "lvstyx_file_write.vi"("int64"=w3462, "path"=w3479, "client ptr"=w3480) -> ()  [unwired: 7 in, 2 out]
      }
      frame "User Input - Lead-off Detect Enable" {
        n1036 = Variant To Data(Variant=w3516, type=T26."DC lead-off detection" ("NewVal")) -> (data=w3509:T26)  [unwired: 1 in, 1 out]
        n1037 = case shown="\"AC lead-off detection at fdr/4\"" w3509 {
          tunnel: w3514 -> [w3526 w3533]
          tunnel: w3513 -> [w3525 w3532]
          tunnel: [w3526 w3535] -> w3512
          tunnel: [w3525 w3534] -> w3511
          frame Default {
          }
          frame "AC lead-off detection at fdr/4" {
            n1038 = local read "CONFIG4"() -> (w3528:T10)
            n1039 = Bundle By Name(cluster=w3528, "PD_LOFF_COMP"=T30."Comparator Enabled") -> (w3531:T10)
            n1040 = call-poly <userlib>:"Enqueue - ClusterQueue.vi"("error in (no error)"=w3532, "Data"="CONFIG4", "Command"="User Input - Config Set", "Queue with Cluster Reference"=w3533) -> ("error out"=w3534:errorcluster, "Queue Out (dup)"=w3535:T31)  [unwired: 2 in, 4 out]
            n1041 = local write "CONFIG4"(w3531) -> ()
          }
        }
      }
      frame "User Input - WriteReadADC" {
        w3540 = "/ads1299bb/conf/rw24bit" ("initial string")
        # "abandoned in place"
        n1042 = Unbundle By Name(w3545) -> ("Client ptr"=w3542:u32)
        n1043 = Number To Decimal String(number="ADC_WriteValue") -> (decimal integer string=w3544:string)  [unwired: 1 out]
        n1044 = call "lvstyx_write_path.vi"("buf"=w3544, "path"=w3540, "client ptr"=w3542) -> ("dup client ptr"=w3541:u32)  [unwired: 6 in, 2 out]
        n1045 = call "lvstyx_read_all_path.vi"("path"=w3540, "client ptr"=w3541) -> ("buf"=w3539:string)  [unwired: 7 in, 2 out]
        n1046 = Decimal String To Number(string=w3539) -> (number=→"ADC_ReadbackValue":i32)  [unwired: 3 out]
        n1047 = call-poly <userlib>:"Enqueue - ClusterQueue.vi"("Command"="Idle", "Queue with Cluster Reference"=w3553) -> ("error out"=w3551:errorcluster, "Queue Out (dup)"=w3552:T31)  [unwired: 4 in, 4 out]
      }
    }
  }
  n1048 = call <vilib>:"Wait at Rendezvous.vi"("error in (no error)"=w11, "rendezvous"=w5) -> ("error out"=w10:errorcluster)  [unwired: 1 in, 4 out]
  n1049 = Release Notifier(notifier=w32, force destroy? (F)=TRUE, error in (no error)=w31) -> (error out=w7:errorcluster)  [unwired: 2 out]
  n1050 = call <vilib>:"Wait at Rendezvous.vi"("error in (no error)"=w7, "rendezvous"=w5) -> ("error out"=w6:errorcluster)  [unwired: 1 in, 4 out]
  n1051 = Unregister For Events(event registration refnum=w33, error in=w34) -> (error out=w9:errorcluster)
  n1052 = call <vilib>:"Wait at Rendezvous.vi"("error in (no error)"=w9, "rendezvous"=w5) -> ("error out"=w8:errorcluster)  [unwired: 1 in, 4 out]
  n1053 = Merge Errors(w6, w8) -> (w28:errorcluster)
  n1054 = flat-sequence "Combine errors and close references" {
    tunnel: w23 -> [w3568]
    tunnel: w21 -> [w3567]
    tunnel: w22 -> [w3565]
    tunnel: w28 -> [w3564]
    tunnel: w27 -> [w3558]
    tunnel: w10 -> [w3557]
    tunnel: [w3563] -> w14
    tunnel: [w3571] -> w13
    tunnel: w14 -> [w3571]
    tunnel: w12 -> [w3570]
    frame #0 {
      n1055 = Merge Errors(w3564, w3568, w3557) -> (w3561:errorcluster)
      n1056 = Flush Queue(queue=w3558, error in (no error)=w3561) -> (queue out=w3559:T31, error out=w3560:errorcluster)  [unwired: 1 out]
      n1057 = Release Queue(queue=w3559, error in (no error)=w3560) -> (error out=w3562:errorcluster)  [unwired: 3 out]
      n1058 = Destroy User Event(user event=w3567, error in=w3562) -> (error out=w3566:errorcluster)
      n1059 = Destroy User Event(user event=w3565, error in=w3566) -> (error out=w3563:errorcluster)
    }
    frame #1 {
      n1060 = Not(x=w3570) -> (.not. x?=w3569:bool)
      n1061 = Quit LabVIEW(quit? (T)=w3569) -> ()
    }
  }
  "error out" <- w13
